vi "RAMM_merFISH_Main.vi"() -> ()   [LabVIEW 2015]
uses:
  CONTROLS/Q_main_element.ctl
  CONTROLS/Q_camera_element.ctl
  CONTROLS/Global parameters.ctl
  CONTROLS/Illumination and filters.ctl
  CONTROLS/Q_DAQ_element.ctl
  CONTROLS/Q_ASI_stage_element.ctl
  CONTROLS/Q_MCL_piezo_element.ctl
  CONTROLS/Q_PUMP_element.ctl
  CONTROLS/Q_VALVE_element.ctl
  <vilib>/vision/Image Controls.llb/IMAQ Image.ctl
  CONTROLS/Q_FPGA_element.ctl
  CONTROLS/Laser emission status.ctl
  GLOBAL/Global_MAIN.vi
  GLOBAL/Global_ABORT.vi
  GLOBAL/Global_CAMERA.vi
  GLOBAL/Global_MCL_piezo.vi
  <vilib>/regexp/Match Regular Expression.xnode
panel:
  in  "Tab general":T1(tab)
  in  "merFISH mode":u16(ring) items=["Embryo", "Single ROI"]
  in  "Close LabView?":bool caption="Close LabView at the end?"
  in  "N movies":i32=1
  in  "Piezo step (um)":dbl=0.05
  in  "Tab small":enum32{"Scanning", "Autofocus", "Fluidics"}(tab)
  in  "Define mosaic":bool
  in  "Save embryo":bool
  in  "Abort scan":bool
  out "Number steps":i32
  out "Scan slider":u8(slide) scale=0.0..100.0
  out "Laser lines manager":i32(listbox)=-1
  in  "Start scan":bool
  in  "step length (nm)":u32=250
  in  "Total  range (nm)":u32=10000
  in  "Illumination source":bool
  in  "Select laser lines":bool
  in  "Discard ROIs":bool
  out "XY positions":cluster{dbl[], dbl[]}[](graph)
  in  "Save X/Y position":bool
  in  "Load X/Y positions":bool
  in  "ROI manager":i32(listbox)
  in  "Brightfield intensity":dbl
  in  "Mosaic size X":i32(ring) items=["1", "3", "5", "7", "9", "11"]
  in  "Mosaic size Y":i32(ring) items=["1", "3", "5", "7", "9", "11"]
  in  "FOV size (um)":dbl=200.0 min=0.0 step=0.1 format="%#.1f"
  in  "Measure QPD":bool
  in  "Init":bool
  in  "PID gains":T2={"proportional gain (Kc)"=10.0, "integral time (Ti, min)"=0.5, "derivative time (Td, min)"=0.0} {"derivative time (Td, min)" format="%.3f"; "integral time (Ti, min)" format="%.3f"; "proportional gain (Kc)" format="%.3f"}
  in  "Autofocus":bool
  in  "Switch":bool
  in  "Autotune?":bool
  in  "Calib autofocus":bool caption="Calibration"
  out "Sensitivity (nm)":dbl
  out "Calibration":cluster{"Y":dbl[], "Y":dbl[]}[](graph)
  in  "Save setpoint":bool
  out "merFISH setpoint":sgl
  in  "Ref channel":u16(ring) items=["X signal", "Y signal"]
  out "Photobleaching manager":i32(listbox)
  in  "Define list":bool
  in  "Two-way valve":bool
  in  "Probe list":i32(listbox)=1
  in  "Pressure (mbar)":dbl min=0.0 max=300.0
  in  "Define injections":bool
  out "Hybridization manager":i32(listbox)
  in  "Buffer list":i32(listbox)=1
  in  "Valve H":u8(knob)=1 min=1 max=22 scale=1.0..22.0
  out "Valve position OUT":u8
  in  "Initialized":bool
  out "Initialization status":T3
  in  "Image contrast":cluster{i32, i32}(slide)={16000, 0} scale=0.0..16000.0
  in  "stop":bool
  out "Error":bool
  in  "Illumination controls":T4 {"641" min=0.0 max=100.0 step=0.1 scale=0.0..100.0; "561" min=0.0 max=100.0 step=0.1 scale=0.0..100.0; "405" min=0.0 max=100.0 step=0.1 scale=0.0..100.0; "488" min=0.0 max=100.0 step=0.1 scale=0.0..100.0; "BF" min=0.0 max=100.0 step=0.1 scale=0.0..100.0}
  in  "Saving path":path=path "E:/DATA"
  in  "Sample name":string="RAMM_Test"
  in  "Save movie":bool
  in  "N frames":i32=100
  out "Slider save movie":u8(slide) scale=0.0..100.0
  out "Frames":i32
  in  "Abort movie":bool
  out "ROI":T5(plugin-control)
  out "Intensity range":cluster{sgl, sgl}(slide) scale=0.0..16000.0
  out "Cooler ON?":bool
  in  "Start acquisition":bool
  out "Sensor Temperature (°C)":sgl
  in  "Exp time (s)":sgl=0.05 format="%#_3g"
  out "Kin time (s)":sgl format="%.3f"
  out "Image":T5(plugin-control)
  in  "Set roi":bool
  in  "Reset roi":bool
  in  "Autofocus automatic correction":bool=TRUE
  out "instruction":string
  out "Autofocus lost":bool
  in  "Alert email adress":string="sergio.espinola@cbs.cnrs.fr " caption="Recipients"
  in  "Display?":bool=TRUE
  in  "DAPI":bool
  in  "Brightfield":bool
  out "merFISH init":T6
  in  "merFISH":bool
  in  "Abort merFISH":bool
  in  "Defaut injection photobleaching":i32[][](array[numeric])=[[10, 500, 350, 0], [0, 1200, 120, 0], [10, 500, 300, 21], [5, 2000, 222, 21], [10, 1200, 300, 22], [5, 800, 350, 1], [0, 150, 100, 1]]
  in  "Q_VALVE":T7={"variant"=variant, "Instruction"=enum."VALVE_initialize"}
  out "MAIN_consumer":errorcluster
  out "ASI":errorcluster
  in  "Q_ASI_stage":T8={"variant"=variant, "Instruction"=enum."ASI_initialize"}
  in  "VISA stage port :":refnum<visa-resource-name>="COM4"
  out "Global parameters":T9 {"# repetitions" min=0; "Dt (s)" min=0 step=1; "Filter list" items=["ET665lp", "zet405/488/561/640m", "None", "None", "None", "None"]}
  out "MAIN_producer":errorcluster
  in  "Q_CAMERA":T10={"variant"=variant, "Instruction"=enum."CAMERA_initialize"}
  in  "Q_main_element":T11={"variant"=variant, "Instruction"=enum."Main_CAMERA_initialization_results"}
  in  "Q_DAQ":T12
  in  "Q_MCL_Piezo":T13
  out "Piezo":errorcluster
  out "DAQ":errorcluster
  out "sCMOS":errorcluster
  in  "Q_PUMP":T14={"variant"=variant, "Instruction"=enum."PUMP_initialize"}
  in  "VISA valve port :":refnum<visa-resource-name>="COM1"
  out "Valve":errorcluster
  out "Pump":errorcluster
  in  "Defaut injection":i32[][](array[numeric])=[[10, 500, 350, 0], [0, 1200, 120, 0], [10, 500, 300, 21], [5, 2000, 222, 21], [10, 1200, 300, 22], [5, 800, 350, 1], [0, 150, 100, 1]]
  out "FPGA":errorcluster
  # "Hamilton valve"
  # "Two-way valve"
  # "Fluigent pump"
  # "First col = Pressure (mbar)\nSecond col = injected volume (ml)\nThird col = Flow rate (µl/min)\nFourth col = valve (#0 is RT)"
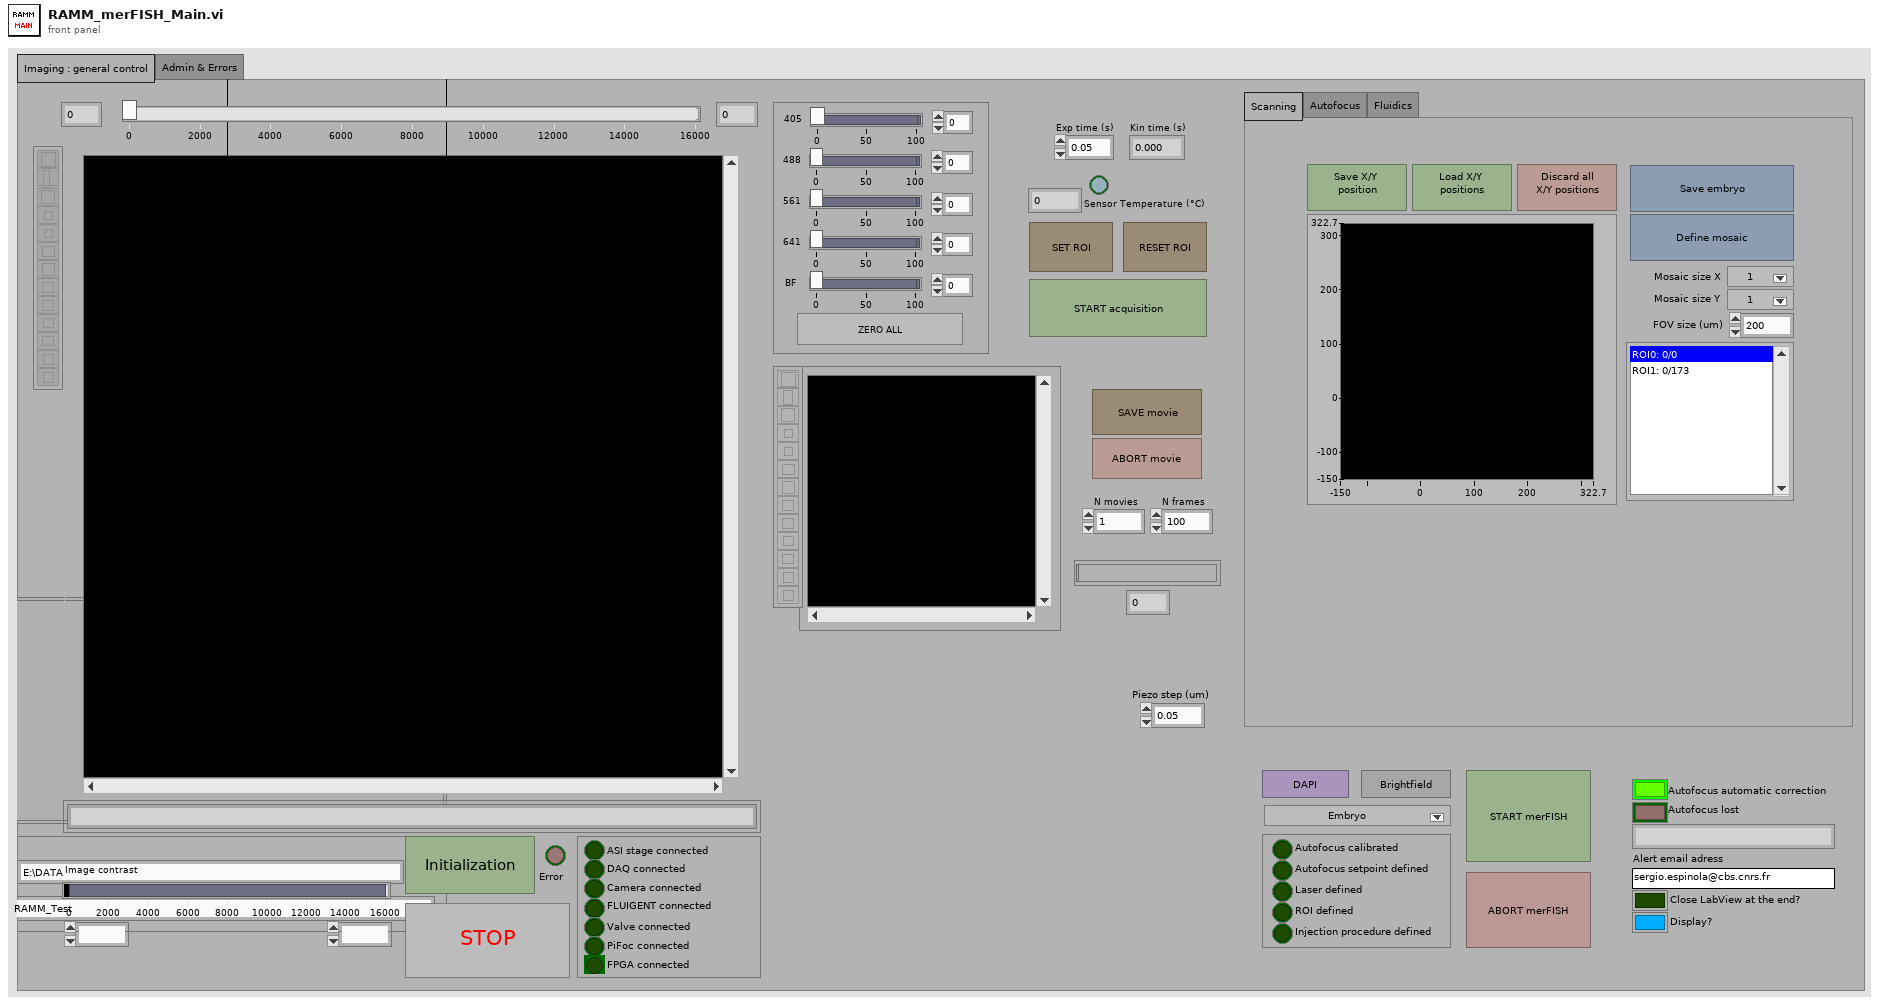
[diagram p1: front panel]
types:
  T1 = enum32{"Imaging : general control", "Admin & Errors"}
  T2 = cluster{"proportional gain (Kc)":dbl, "integral time (Ti, min)":dbl, "derivative time (Td, min)":dbl}
  T3 = cluster{"ASI":bool, "DAQ":bool, "Camera":bool, "Pump":bool, "Valve":bool, "PiFoc":bool, "FPGA":bool}
  T4 = typedef "Illumination and filters.ctl" = cluster{"BF ":dbl, "641":dbl, "561":dbl, "488":dbl, "405":dbl, "ZERO ALL":bool}
  T5 = typedef "IMAQ Image.ctl" = refnum<image>
  T6 = cluster{"Autofocus calibrated":bool, "Autofocus setpoint defined":bool, "Laser defined":bool, "ROI defined":bool, "Injection procedure defined":bool}
  T7 = typedef "Q_VALVE_element.ctl" = cluster{"variant":variant, "Instruction":enum16{"VALVE_idle", "VALVE_initialize", "VALVE_error", "VALVE_security_stop", "VALVE_change_position", "VALVE_two_way_valves", "VALVE_init_merFISH", "VALVE_stop"}}
  T8 = typedef "Q_ASI_stage_element.ctl" = cluster{"variant":variant, "Instruction":enum16{"ASI_idle", "ASI_initialize", "ASI_error", "ASI_security_stop", "ASI_read_XYZ", "ASI_up", "ASI_down", "ASI_left", "ASI_right", "ASI_save_XY", "ASI_move_to_XY", "ASI_brightfield", "ASI_init_scan", "ASI_init_merFISH", "ASI_move_to_XY_merFISH", "ASI_move_to_Z_merFISH", "ASI_init_autofocus_search_merFISH", "ASI_close_autofocus_search_merFISH", "ASI_adjust_piezo_autofocus_merFISH", "ASI_set_piezo_autofocus_to_reference_position_merFISH_TL", "ASI_close_merFISH", "ASI_stop"}}
  T9 = typedef "Global parameters.ctl" = cluster{"405":dbl, "488":dbl, "561":dbl, "641":dbl, "BF":dbl, "X":dbl, "Y":dbl, "Filter list":u16, "Exp time":sgl, "Kinetic time":sgl, "Gain":i32, "Step length (nm)":u32, "Total range (nm)":u32, "Scan illumination\n mode":bool, "Dt (s)":i32, "# repetitions":i32}
  T10 = typedef "Q_camera_element.ctl" = cluster{"variant":variant, "Instruction":enum16{"CAMERA_idle", "CAMERA_initialize", "CAMERA_error", "CAMERA_security_stop", "CAMERA_not_acquiring", "CAMERA_acquiring", "CAMERA_start_acquiring", "CAMERA_stop_acquiring", "CAMERA_change_exposure", "CAMERA_define_ROI", "CAMERA_cooler", "CAMERA_acquire_movie", "CAMERA_init_scan", "CAMERA_check_image_scan", "CAMERA_close_scan", "CAMERA_init_merFISH", "CAMERA_start_acquiring_merFISH", "CAMERA_close_scan_merFISH", "CAMERA_close_merFISH", "CAMERA_STOP"}}
  T11 = typedef "Q_main_element.ctl" = cluster{"variant":variant, "Instruction":enum16{"Main_idle", "Main_initialize", "Main_initialize_TDMS", "Main_initialize_Queue", "Main_error", "Main_DAQ_initialization_results", "Main_ASI_initialization_results", "Main_Piezo_initialization_results", "Main_Valve_initialization_results", "Main_Pump_initialization_results", "Main_CAMERA_initialization_results", "Main_FPGA_initialization_results", "Main_DAQ_error", "Main_ASI_error", "Main_Piezo_error", "Main_CAMERA_error", "Main_Valve_error", "Main_Pump_error", "Main_FPGA_error", "Main_start_acquiring", "Main_not_acquiring", "Main_acquiring", "Main_stop_acquiring", "Main_change_exposure", "Main_change_z_scan_parameters", "Main_define_ROI", "Main_define_mosaic", "Main_read_kinetic_time", "Main_cooler", "Main_read_temperature", "Main_save_XY", "Main_load_XY", "Main_discard_XY", "Main_move_to_XY", "Main_measure_QPD", "Main_autofocus_calibration", "Main_autofocus_initialization", "Main_autofocus_stop", "Main_save_PID", "Main_change_H_valve_position", "Main_two_way_valve", "Main_save_movie", "Main_init_single_scan", "Main_single_scan", "Main_stop_single_scan", "Main_merFISH_illumination_parameters", "Main_merFISH_buffer_probe_list", "Main_merFISH_injections_procedure", "Main_merFISH_save_setpoint", "Main_merFISH_DAPI_parameters", "Main_merFISH_Brightfield_parameters", "Main_merFISH_save_embryo_ROI", "Main_merFISH_init", "Main_merFISH_resume", "Main_merFISH_start_autofocus", "Main_merFISH_open_close_valve_merFISH", "Main_merFISH_open_close_valve_photobleaching", "Main_merFISH_hybridization", "Main_merFISH_move_to_ROI", "Main_merFISH_wait_stabilization", "Main_merFISH_move_to_REF", "Main_merFISH_scan", "Main_merFISH_photobleaching_injection", "Main_merFISH_photobleaching", "Main_merFISH_send_email", "Main_merFISH_close", "Main_STOP"}}
  T12 = typedef "Q_DAQ_element.ctl" = cluster{"variant":variant, "Instruction":enum16{"DAQ_idle", "DAQ_initialize", "DAQ_error", "DAQ_security_stop", "DAQ_init_single_scan", "DAQ_single_scan", "DAQ_init_merFISH", "DAQ_scan_merFISH", "DAQ_photobleaching_merFISH", "DAQ_close_merFISH", "DAQ_stop"}}
  T13 = typedef "Q_MCL_piezo_element.ctl" = cluster{"variant":variant, "Instruction":enum16{"Piezo_idle", "Piezo_initialize", "Piezo_error", "Piezo_security_stop", "Piezo_read_z", "Piezo_move_z", "Piezo_keyboard_move", "Piezo_close_autofocus_calibration_ramp", "Piezo_change_init_state", "Piezo_init_autofocus", "Piezo_init_autofocus_merFISH_TL", "Piezo_autofocus", "Piezo_autofocus_merFISH_TL", "Piezo_stop_autofocus", "Piezo_stop_autofocus_merFISH_TL", "Piezo_autofocus_lost", "Piezo_resume_autofocus_merFISH_TL", "Piezo_check_z_position_merFISH_TL", "Piezo_init_ramp", "Piezo_move_z_ramp", "Piezo_close_ramp", "Piezo_close_merFISH", "Piezo_stop"}}
  T14 = typedef "Q_PUMP_element.ctl" = cluster{"variant":variant, "Instruction":enum16{"PUMP_idle", "PUMP_initialize", "PUMP_error", "PUMP_security_stop", "PUMP_read_pressure", "PUMP_change_pressure", "PUMP_init_merFISH", "PUMP_change_presure_merFISH", "PUMP_zero_pressure_merFISH", "PUMP_close_merFISH", "PUMP_stop"}}
  T15 = typedef "Image Type" = u32
  T16 = cluster{"XY positions":dbl[][], "Laser lines array":dbl[][], "Ramp":dbl[], "Total # z steps":i32, "merFISH path":path, "merFISH init":cluster{"Autofocus calibrated":bool, "Autofocus setpoint defined":bool, "Laser defined":bool, "ROI defined":bool, "Injection procedure defined":bool}, "Hybridization procedure":i32[][], "Total # frames":i32, "Slope":dbl, "Photobleaching procedure":i32[][], "Log file":refnum<file>, "Starting time":dbl, "QPD ref":cluster{"X":sgl, "Y":sgl, "SUM":sgl, "count":u32}, "REF positions":dbl[][]}
  T17 = enum8{"Enabled", "Disabled", "Disabled and Grayed Out"}
  T18 = enum16{"Main_idle", "Main_initialize", "Main_initialize_TDMS", "Main_initialize_Queue", "Main_error", "Main_DAQ_initialization_results", "Main_ASI_initialization_results", "Main_Piezo_initialization_results", "Main_Valve_initialization_results", "Main_Pump_initialization_results", "Main_CAMERA_initialization_results", "Main_FPGA_initialization_results", "Main_DAQ_error", "Main_ASI_error", "Main_Piezo_error", "Main_CAMERA_error", "Main_Valve_error", "Main_Pump_error", "Main_FPGA_error", "Main_start_acquiring", "Main_not_acquiring", "Main_acquiring", "Main_stop_acquiring", "Main_change_exposure", "Main_change_z_scan_parameters", "Main_define_ROI", "Main_define_mosaic", "Main_read_kinetic_time", "Main_cooler", "Main_read_temperature", "Main_save_XY", "Main_load_XY", "Main_discard_XY", "Main_move_to_XY", "Main_measure_QPD", "Main_autofocus_calibration", "Main_autofocus_initialization", "Main_autofocus_stop", "Main_save_PID", "Main_change_H_valve_position", "Main_two_way_valve", "Main_save_movie", "Main_init_single_scan", "Main_single_scan", "Main_stop_single_scan", "Main_merFISH_illumination_parameters", "Main_merFISH_buffer_probe_list", "Main_merFISH_injections_procedure", "Main_merFISH_save_setpoint", "Main_merFISH_DAPI_parameters", "Main_merFISH_Brightfield_parameters", "Main_merFISH_save_embryo_ROI", "Main_merFISH_init", "Main_merFISH_resume", "Main_merFISH_start_autofocus", "Main_merFISH_open_close_valve_merFISH", "Main_merFISH_open_close_valve_photobleaching", "Main_merFISH_hybridization", "Main_merFISH_move_to_ROI", "Main_merFISH_wait_stabilization", "Main_merFISH_move_to_REF", "Main_merFISH_scan", "Main_merFISH_photobleaching_injection", "Main_merFISH_photobleaching", "Main_merFISH_send_email", "Main_merFISH_close", "Main_STOP"}
  T19 = cluster{"Saving path":path, "Sample name":string, "N frames":i32, "N movies":i32, "Start acquisition":bool, "Global parameters":T9}
  T20 = cluster{"XY positions":dbl[][], "REF positions":dbl[][]}
  T21 = cluster{"z step (nm)":u32, "Total range (nm)":u32, "N laser lines merFISH":i32, "Start acquisition":bool, "Brightfield intensity":dbl, "Autofocus":bool, "Probe List Refnum":refnum<vi>, "Injection procedure IN":i32[][], "Valve H":u8, "Measure QPD":bool, "Laser lines array":dbl[][], "Exp time (s)":sgl, "Illumination source":bool, "XY positions":dbl[][], "merFISH mode":u16}
  T22 = cluster{"Start acquisition":bool, "Frame transfer":bool, "Movie path":string}
  T23 = cluster{"Log file":refnum<file>, "Starting time":dbl, "Hybridization procedure":i32[][]}
  T24 = cluster{"XY positions":dbl[][], "Slope":dbl, "Starting time":dbl, "Log file":refnum<file>, "QPD ref":cluster{"X":sgl, "Y":sgl, "SUM":sgl, "count":u32}}
  T25 = cluster{"REF positions":dbl[][], "Slope":dbl, "Starting time":dbl, "Log file":refnum<file>, "XY positions":dbl[][], "QPD ref":cluster{"X":sgl, "Y":sgl, "SUM":sgl, "count":u32}}
  T26 = cluster{"QPD ref":cluster{"X":sgl, "Y":sgl, "SUM":sgl, "count":u32}, "Slope":dbl, "Log file":refnum<file>, "Starting time":dbl}
  T27 = cluster{"Ramp":dbl[], "merFISH path":path, "Total # frames":i32, "Display?":bool, "Probe list":refnum<vi>}
  T28 = cluster{"ROI #":i32, "Probe #":i32, "Folder# ":i32, "Embryo #":i32}
  T29 = cluster{"Photobleaching procedure":i32[][], "Log file":refnum<file>, "Starting time":dbl}
  T30 = cluster{"Hybridization procedure":i32[][], "Photobleaching procedure":i32[][], "Alert email adress":string, "Exp time (s)":sgl, "Total  range (nm)":u32, "step length (nm)":u32, "ROIs":dbl[][], "Laser lines array":dbl[][], "merFISH cluster":cluster{"Autofocus calibrated":bool, "Autofocus setpoint defined":bool, "Laser defined":bool, "ROI defined":bool, "Injection procedure defined":bool}, "Sample name":string, "FOV size":dbl, "Mosaic size":u16[], "PID gains":cluster{"proportional gain (Kc)":dbl, "integral time (Ti, min)":dbl, "derivative time (Td, min)":dbl}, "Illumination source":bool, "Brightfield intensity":dbl, "merFISH path":path, "QPD ref":cluster{"X":sgl, "Y":sgl, "SUM":sgl, "count":u32}, "REFs":dbl[][], "N movies":i32, "N frames":i32}
  T31 = cluster{"Hybridization name":string[], "Photobleaching name":string[], "Laser names":string[], "Buffer list names":string[][], "Probe list names":string[][]}
  T32 = cluster{"X":sgl, "Y":sgl, "SUM":sgl, "count":u32}
  T33 = cluster{"Global Rectangle":i32[], "Contours":cluster{"Contour Type":u32, "ROI Type":u32, "Points":i32[]}[]}
  T34 = cluster{"Maximal Value":sgl, "Minimal Value":sgl}
  T35 = cluster{"queue FPGA":refnum<queue>, "queue pump":refnum<queue>, "queue valve":refnum<queue>, "queue DAQ":refnum<queue>, "queue CAMERA":refnum<queue>, "queue ASI stage":refnum<queue>, "queue piezo":refnum<queue>}
  T36 = cluster{"Z_position_file path":path, "Movie path":path, "Acquisition_parameters path":path}
  T37 = enum16{"open", "open or create", "create or replace", "create", "open (read-only)"}
  T38 = typedef "Q_FPGA_element.ctl" = cluster{"variant":variant, "Instruction":enum16{"FPGA_idle", "FPGA_initialize", "FPGA_error", "FPGA_security_stop", "FPGA_laser", "FPGA_start_stop_measure_QPD", "FPGA_measure_QPD", "FPGA_measure_QPD_noise", "FPGA_stop_measure_QPD", "FPGA_init_autofocus", "FPGA_init_single_scan", "FPGA_stop_single_scan", "FPGA_init_merFISH", "FPGA_measure_QPD_merFISH", "FPGA_init_scan_merFISH", "FPGA_scan_merFISH", "FPGA_close_merFISH", "FPGA_stop"}}
  T39 = typedef "Laser emission status.ctl" = cluster{"405":bool, "488":bool, "561":bool, "641":bool, "BF":bool}
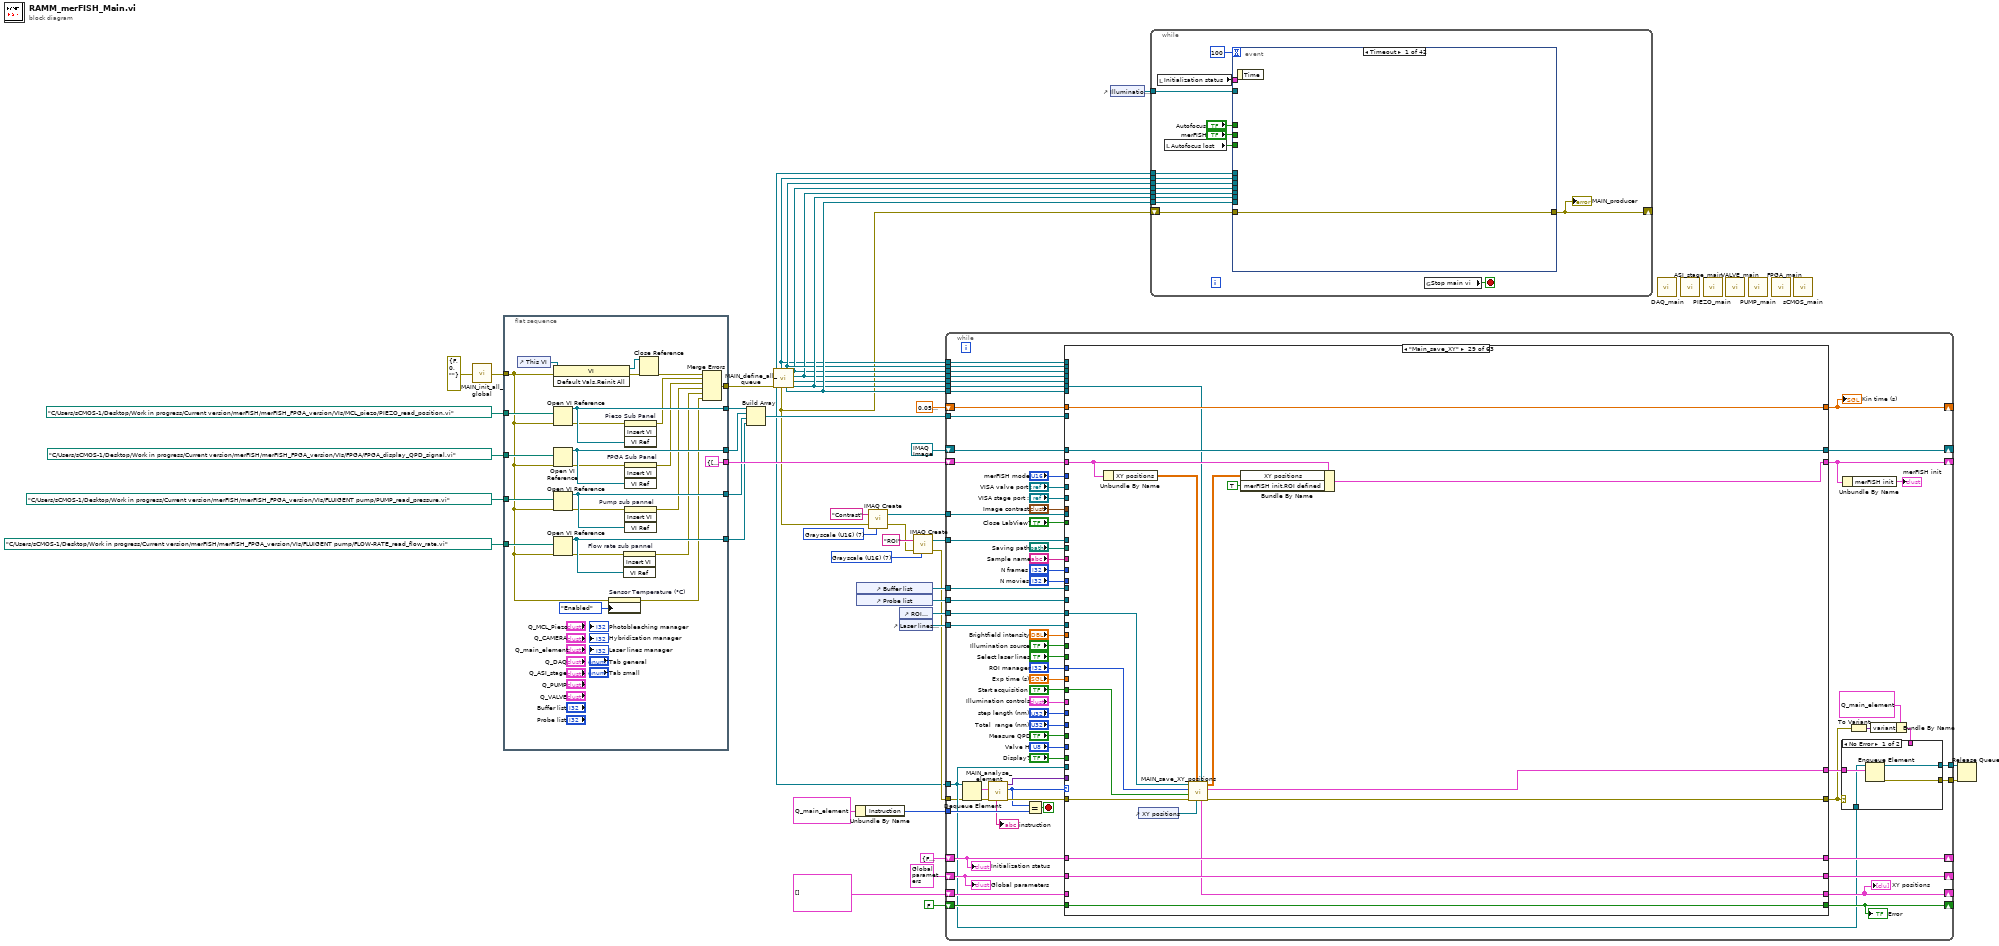
[diagram p0: block diagram]
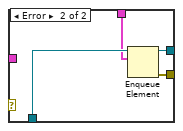
[diagram p2: hidden frame]
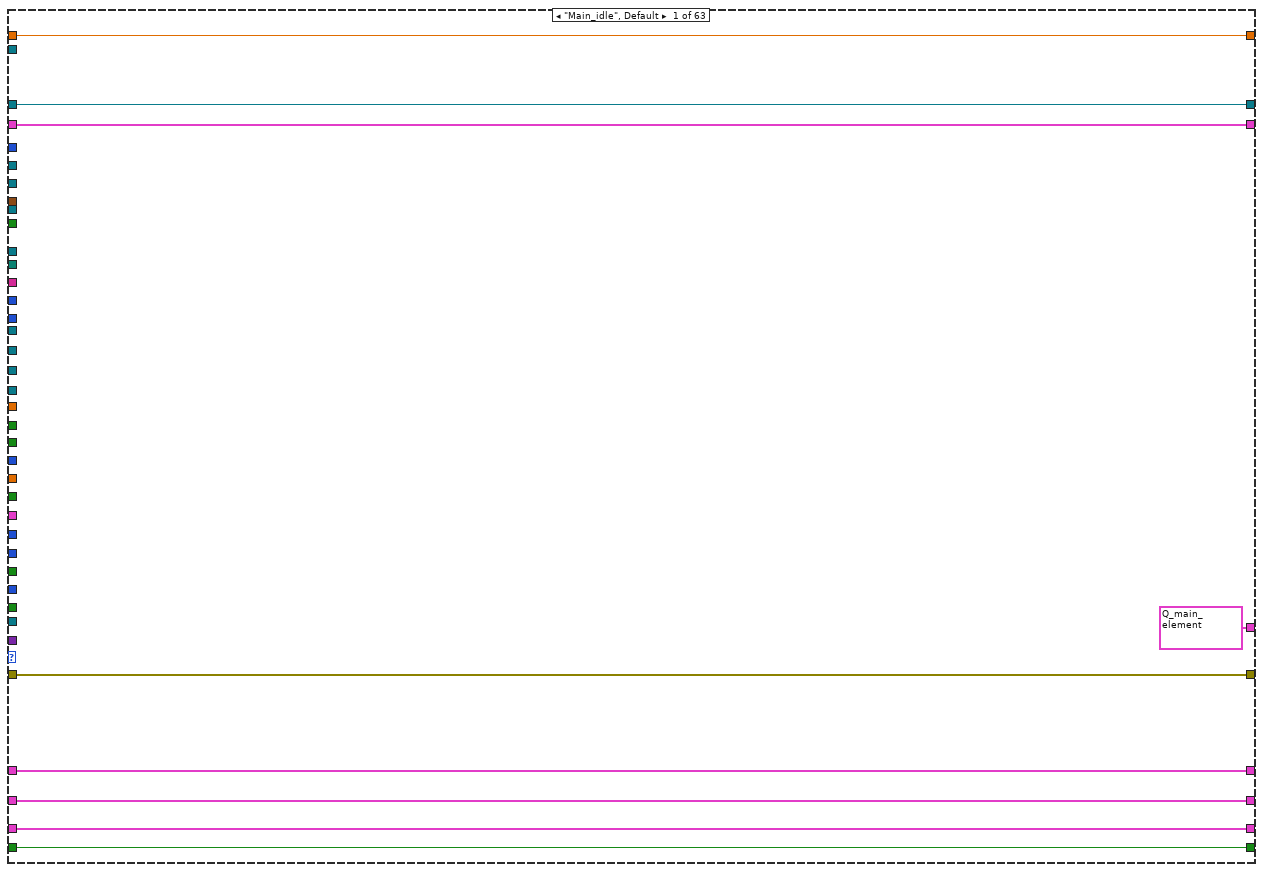
[diagram p3: hidden frame]
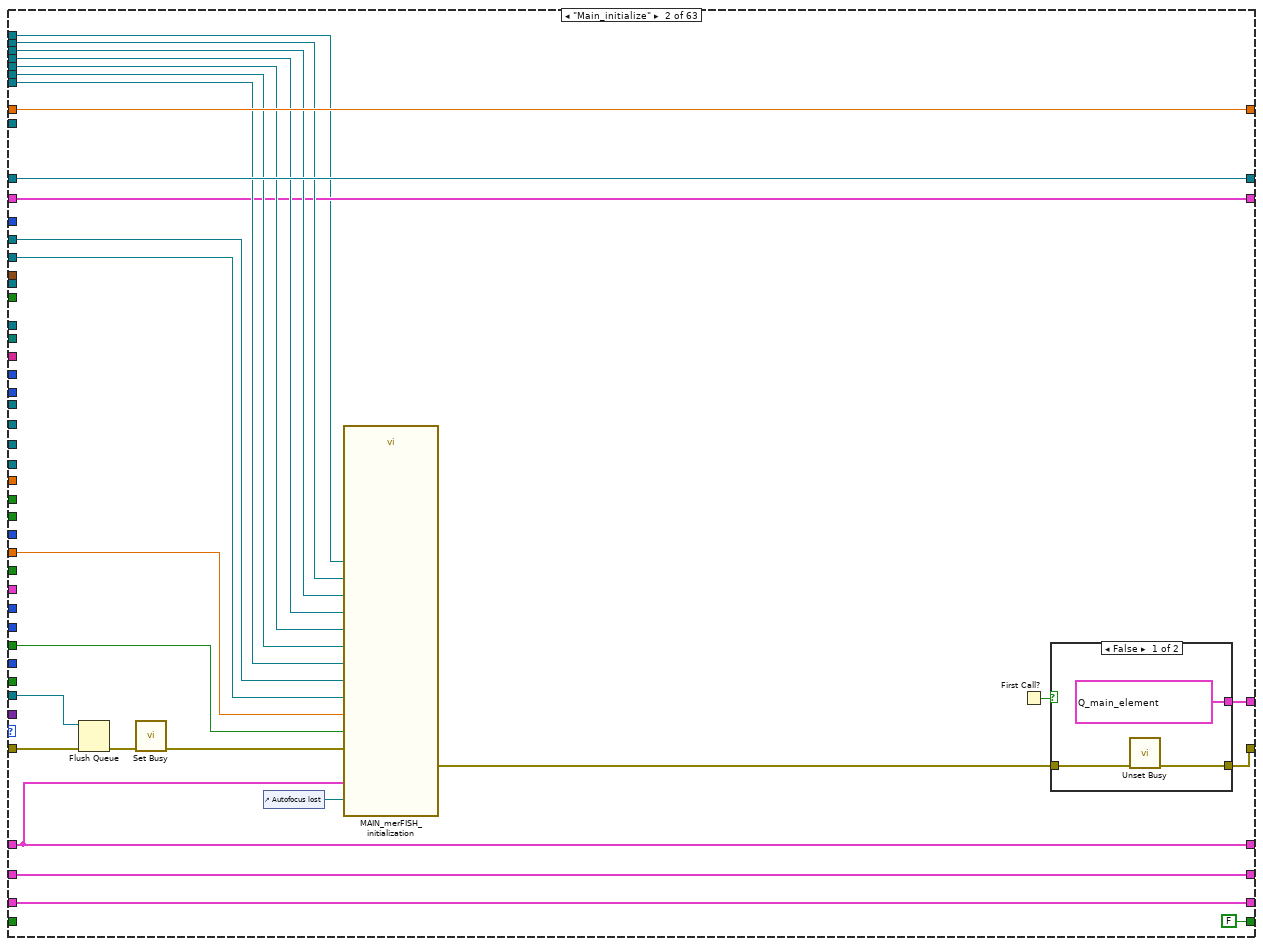
[diagram p4: hidden frame]
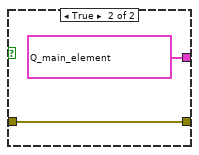
[diagram p5: hidden frame]
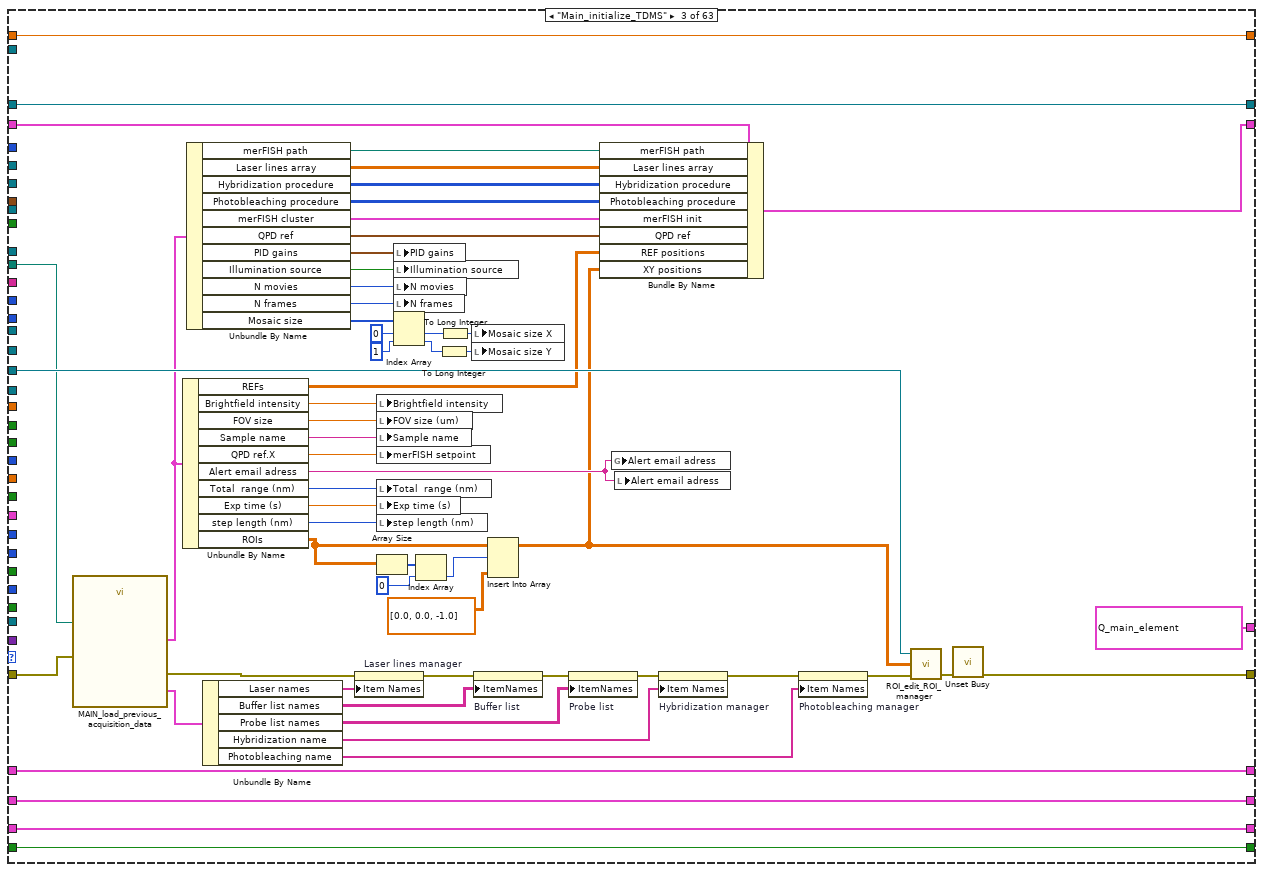
[diagram p6: hidden frame]
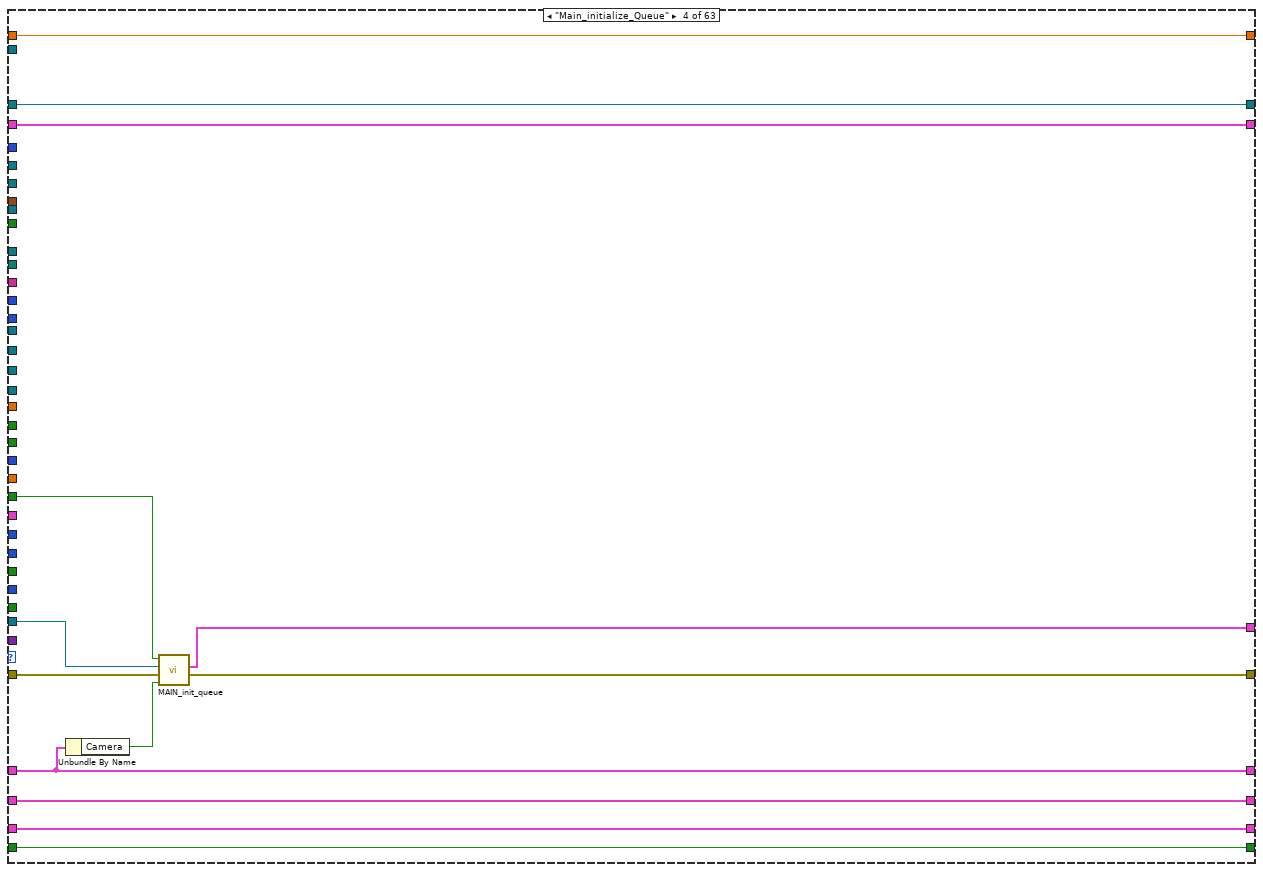
[diagram p7: hidden frame]
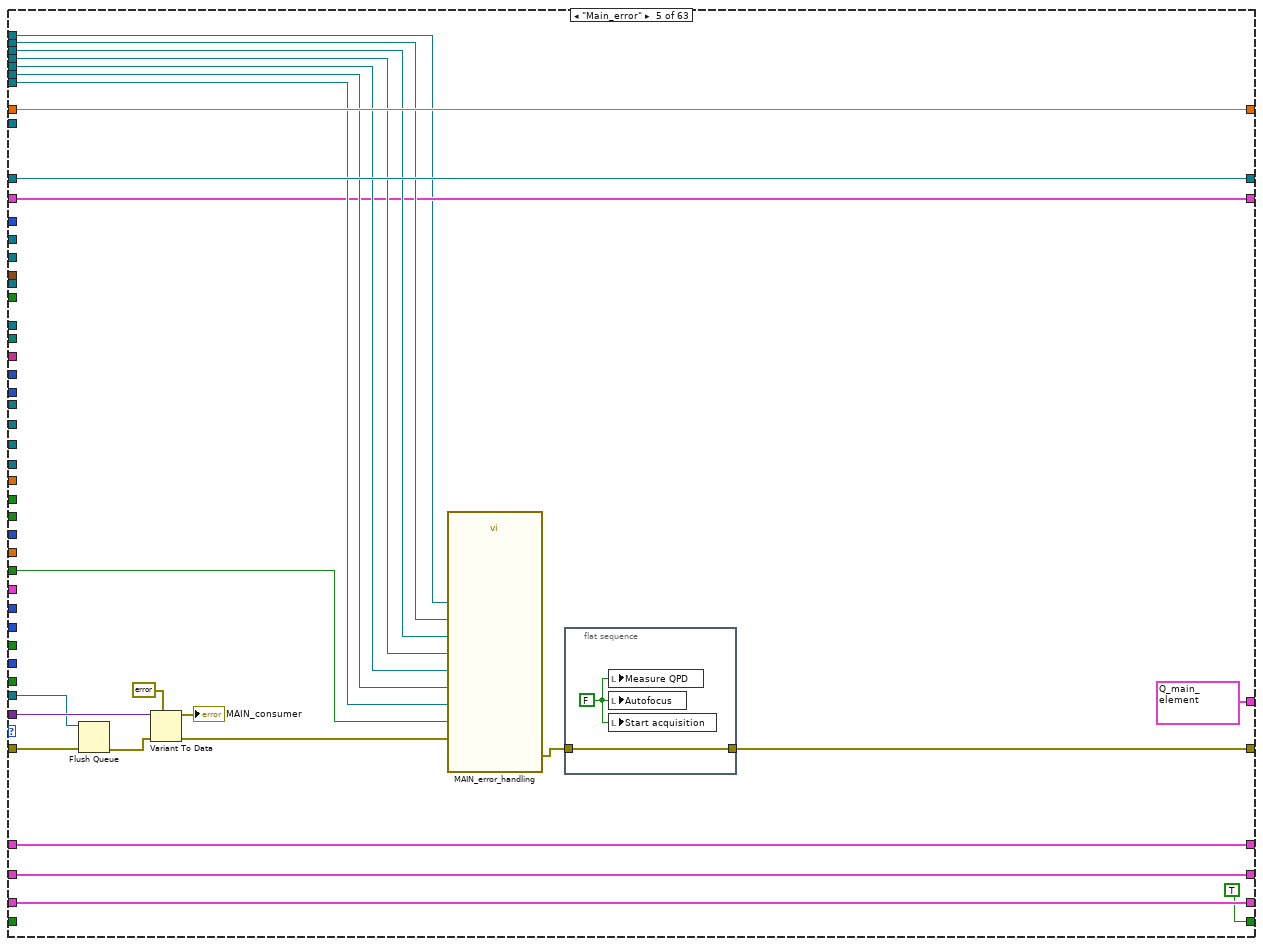
[diagram p8: hidden frame]
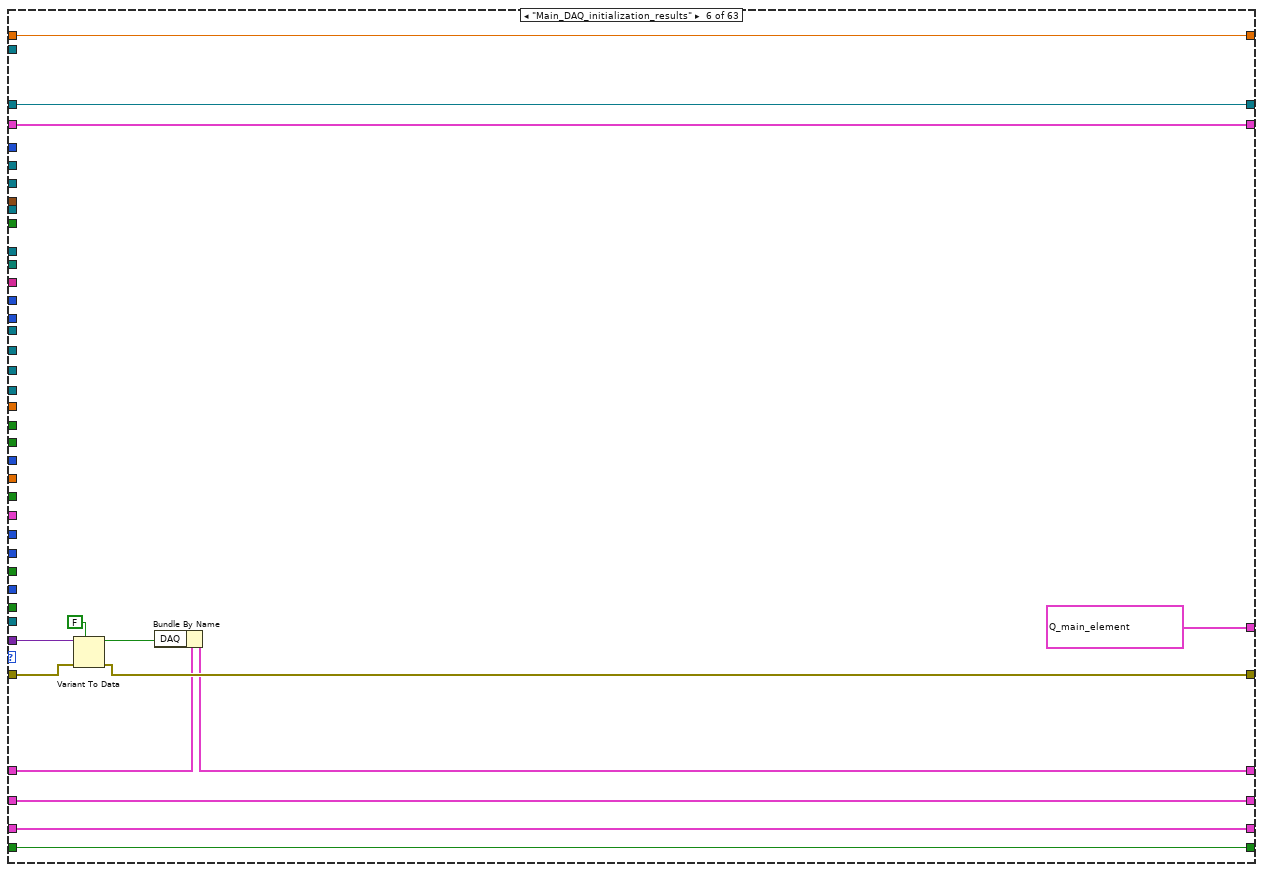
[diagram p9: hidden frame]
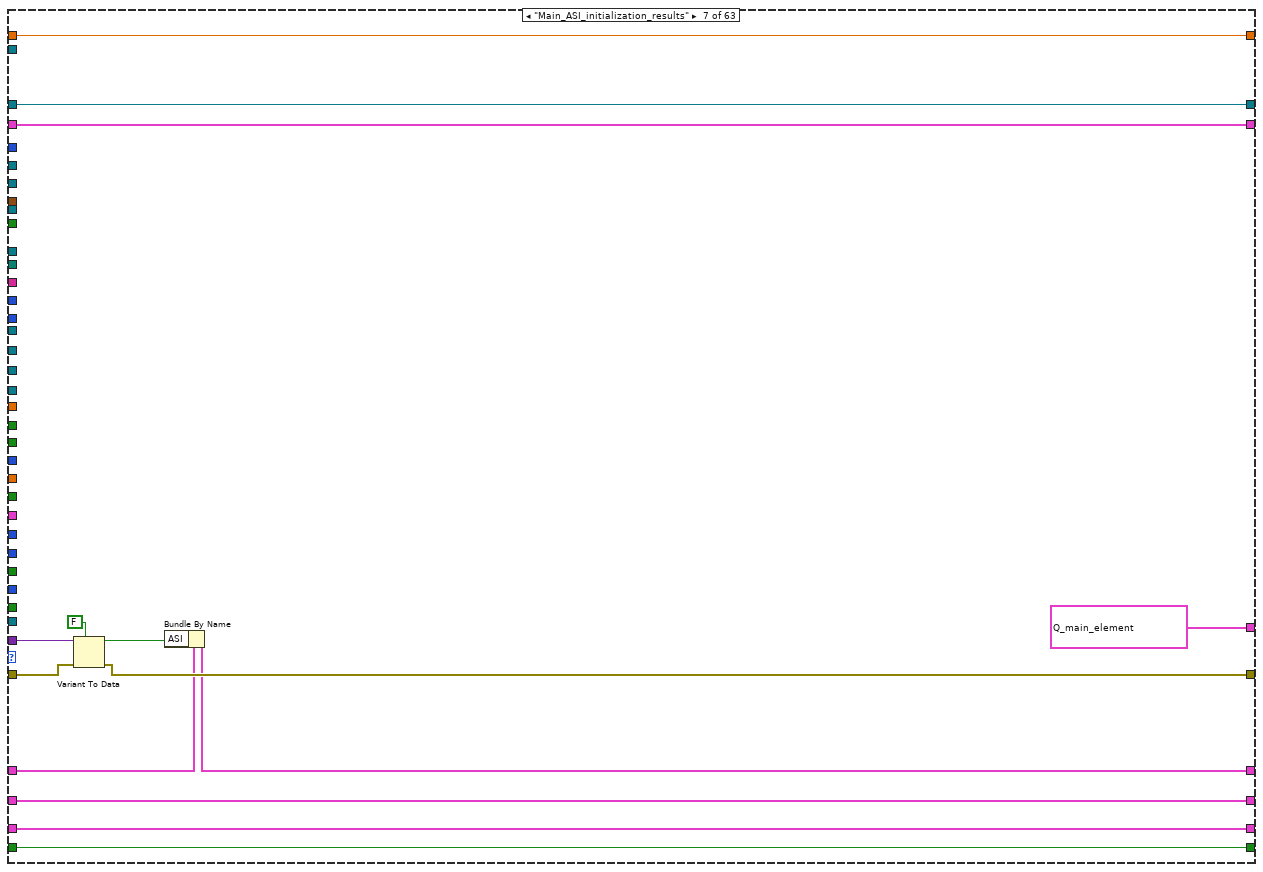
[diagram p10: hidden frame]
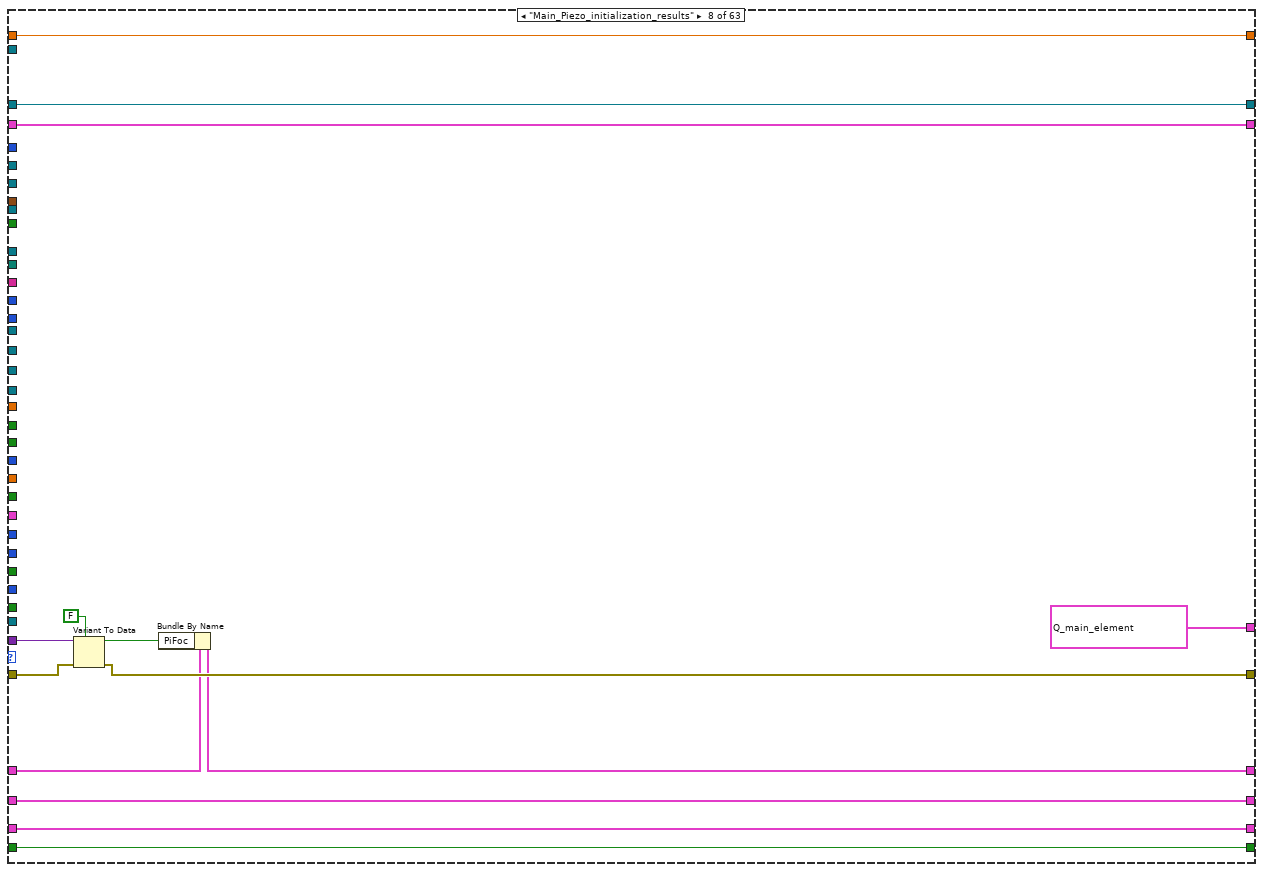
[diagram p11: hidden frame]
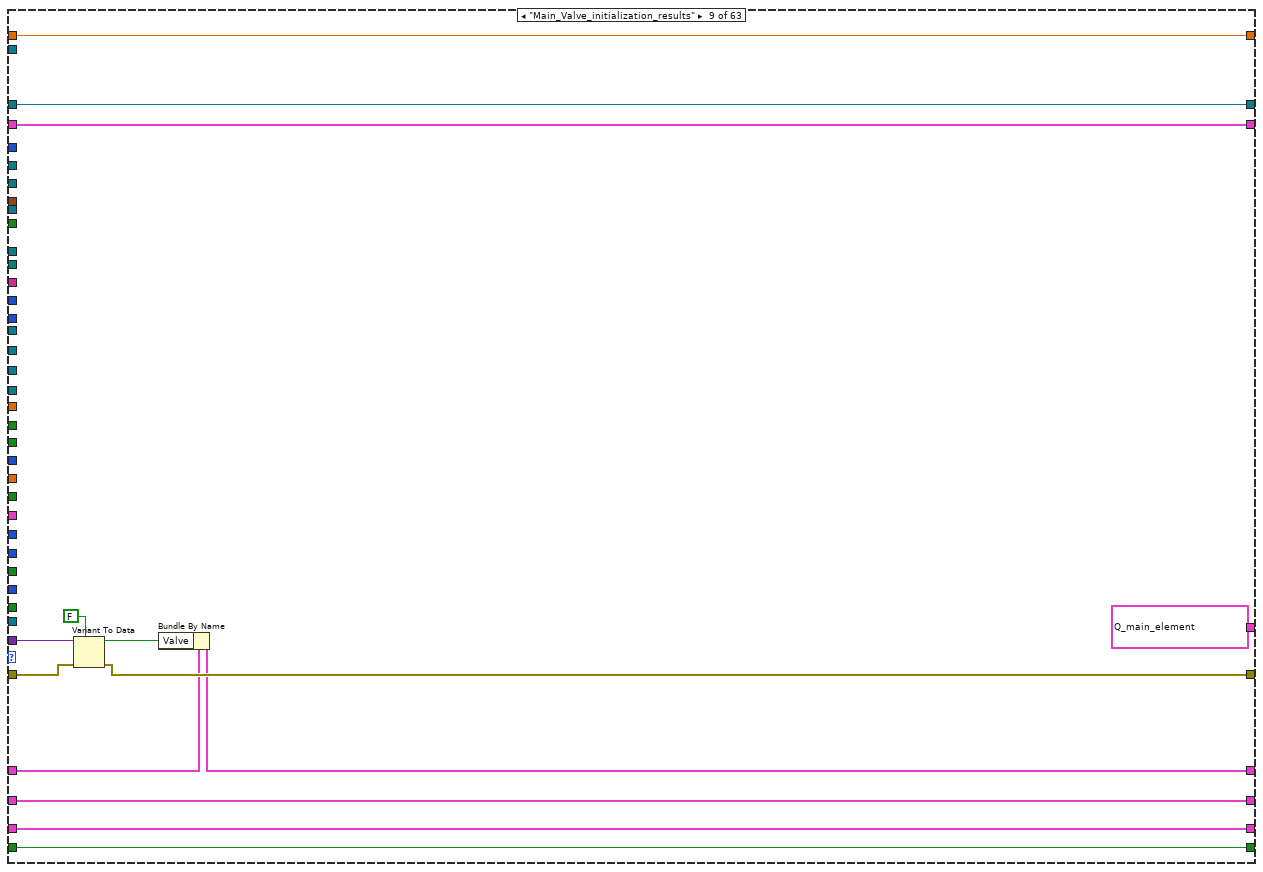
[diagram p12: hidden frame]
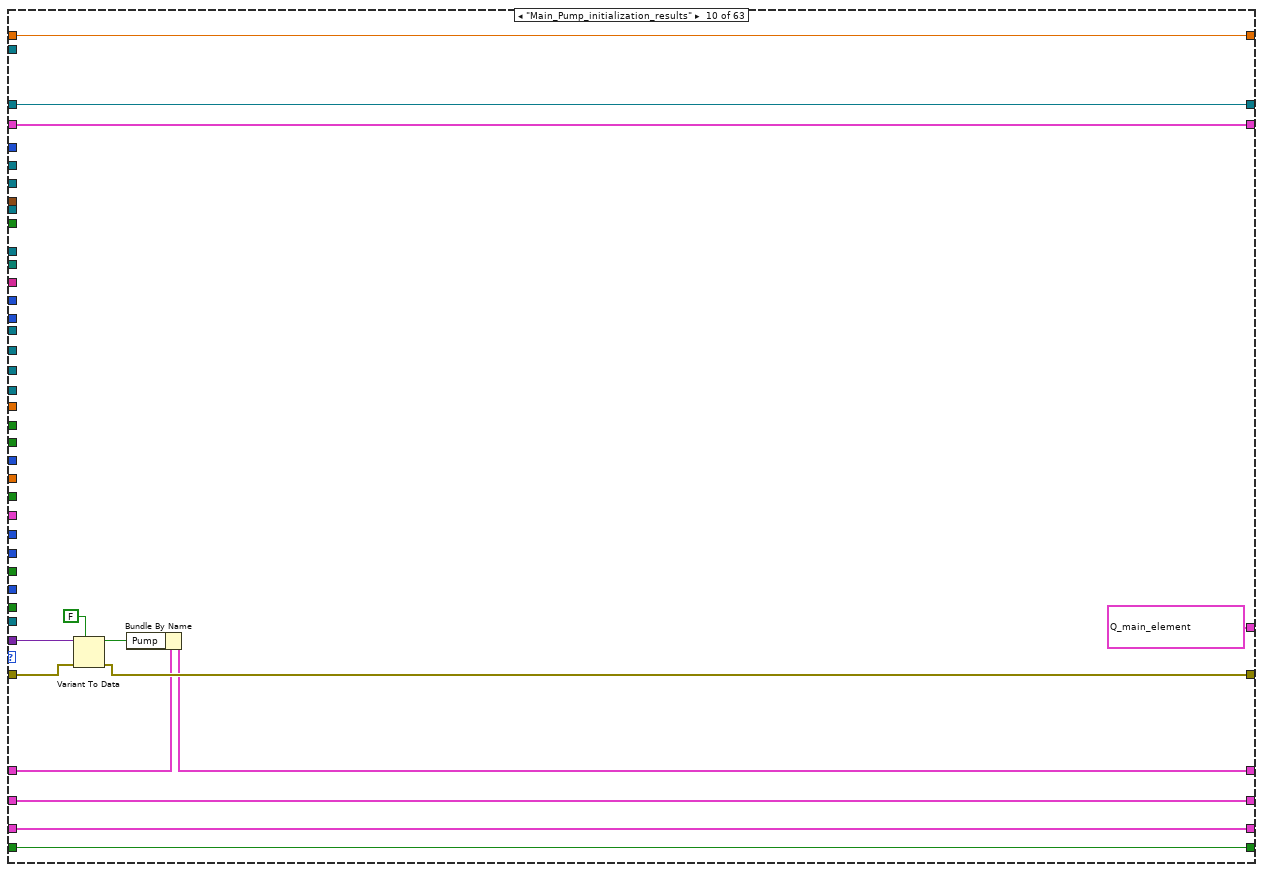
[diagram p13: hidden frame]
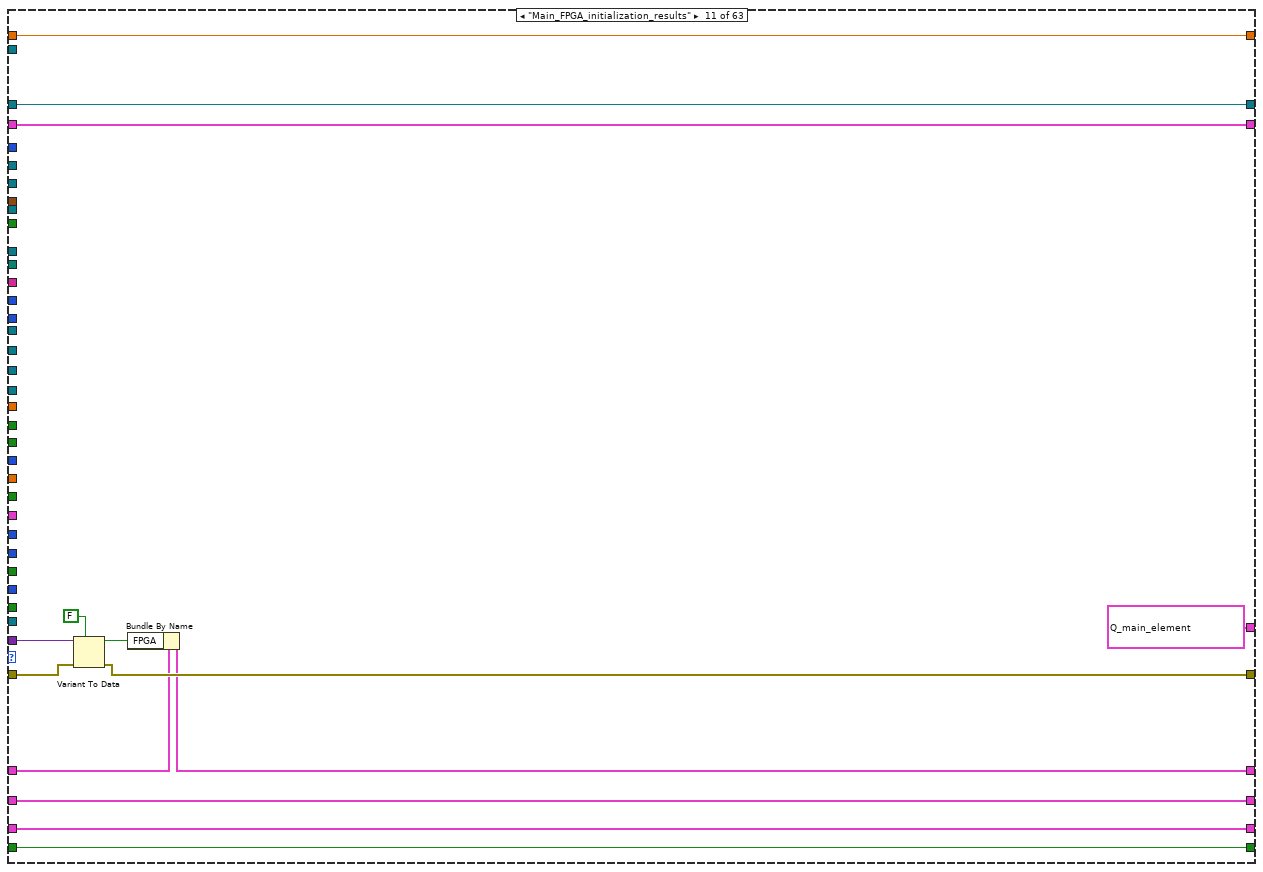
[diagram p14: hidden frame]
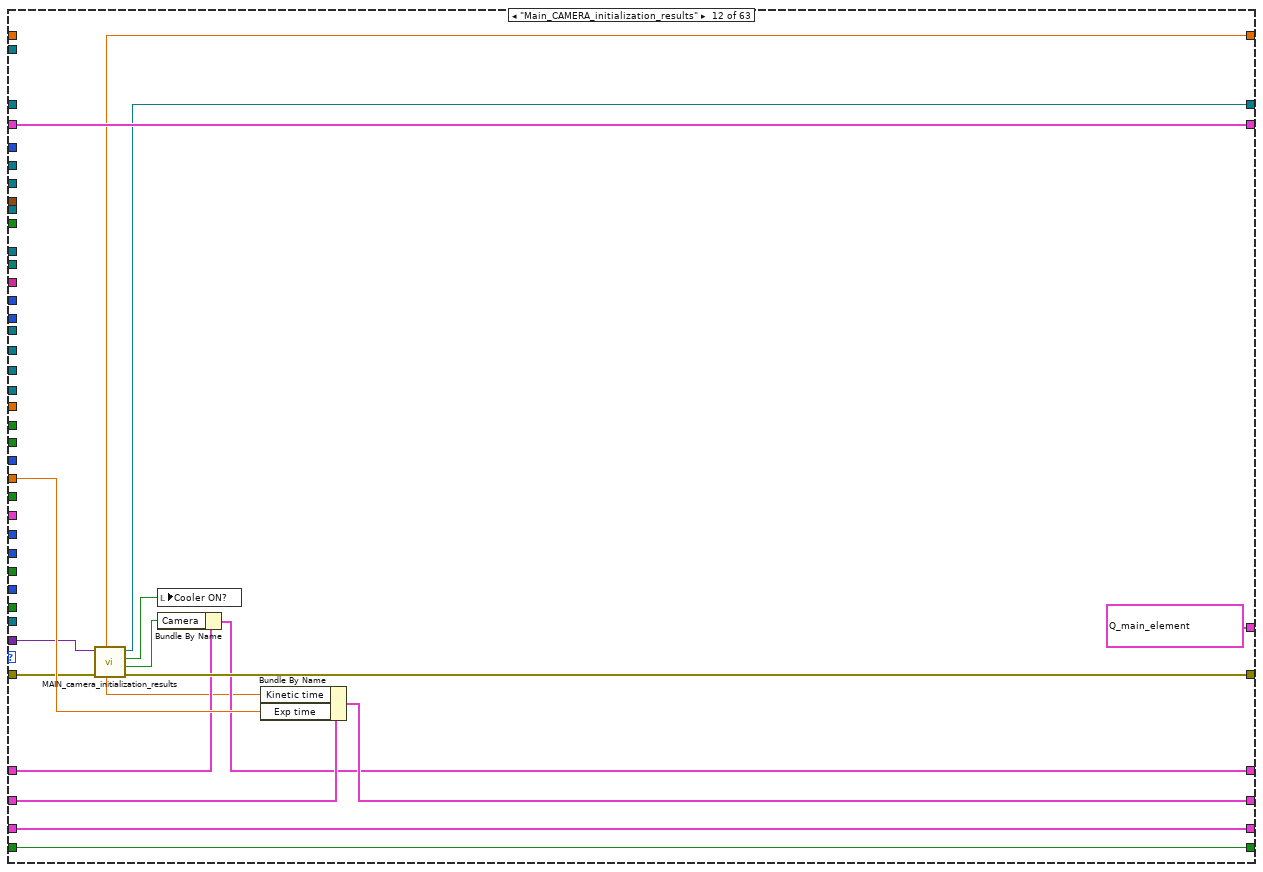
[diagram p15: hidden frame]
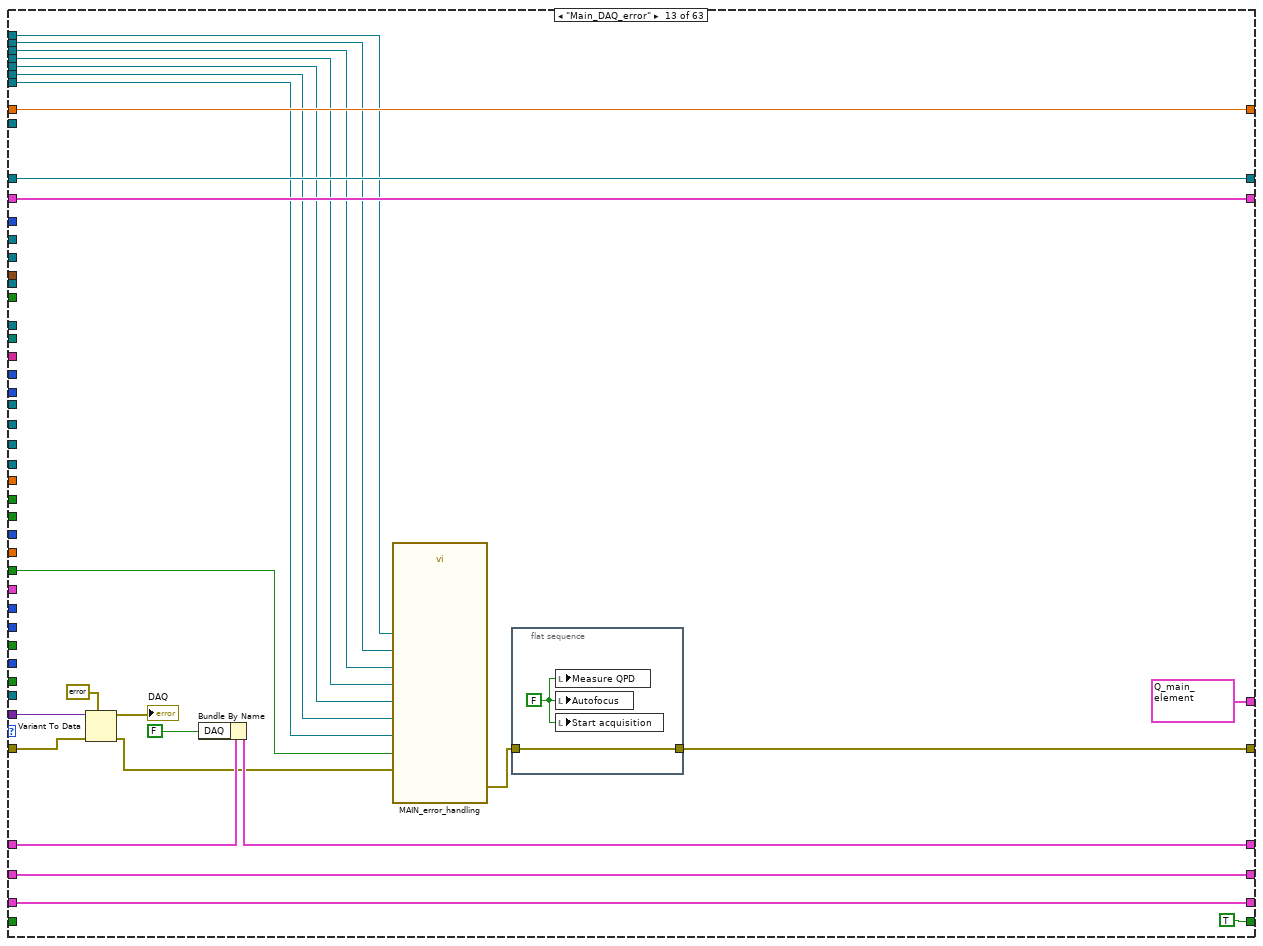
[diagram p16: hidden frame]
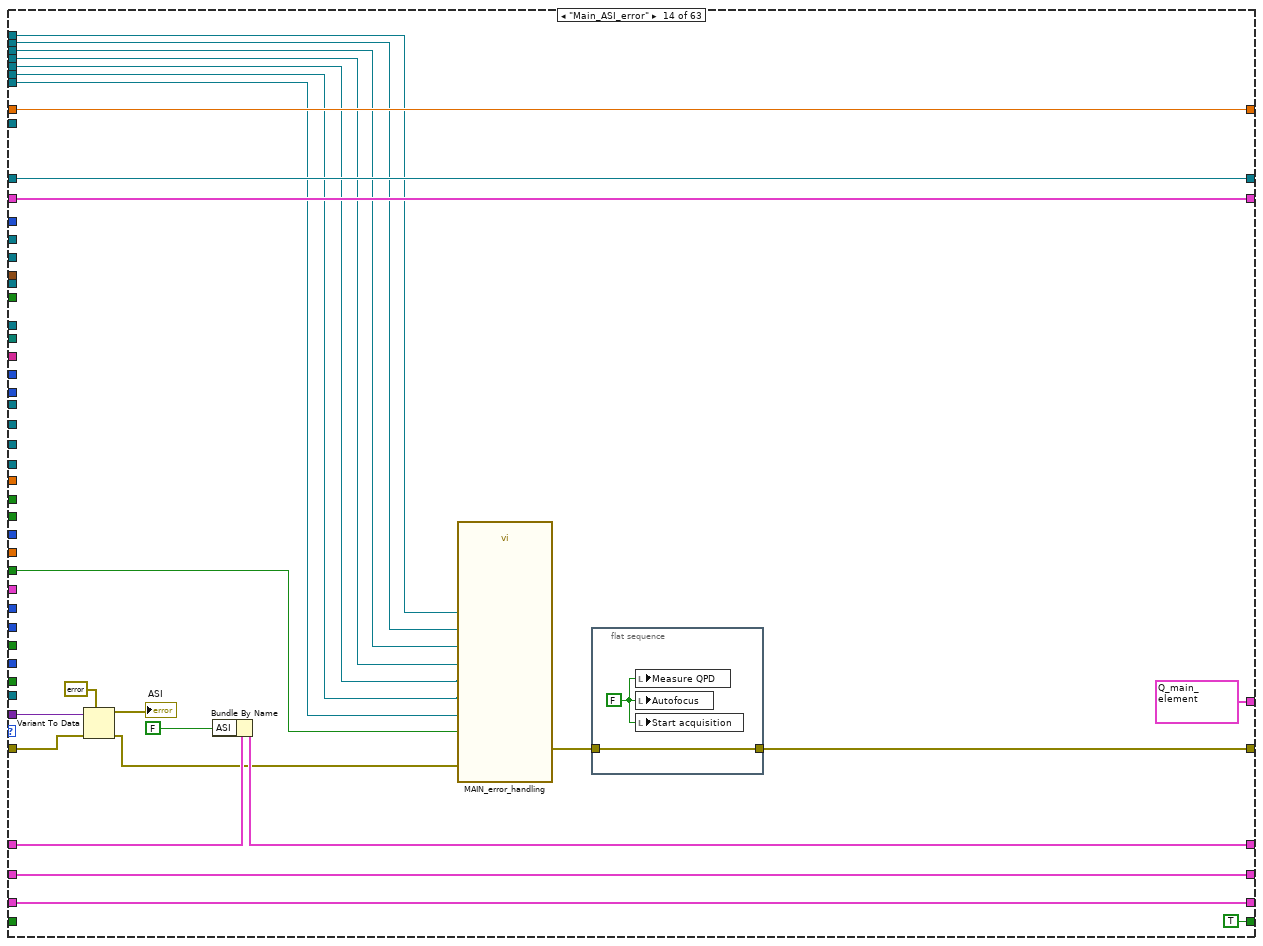
[diagram p17: hidden frame]
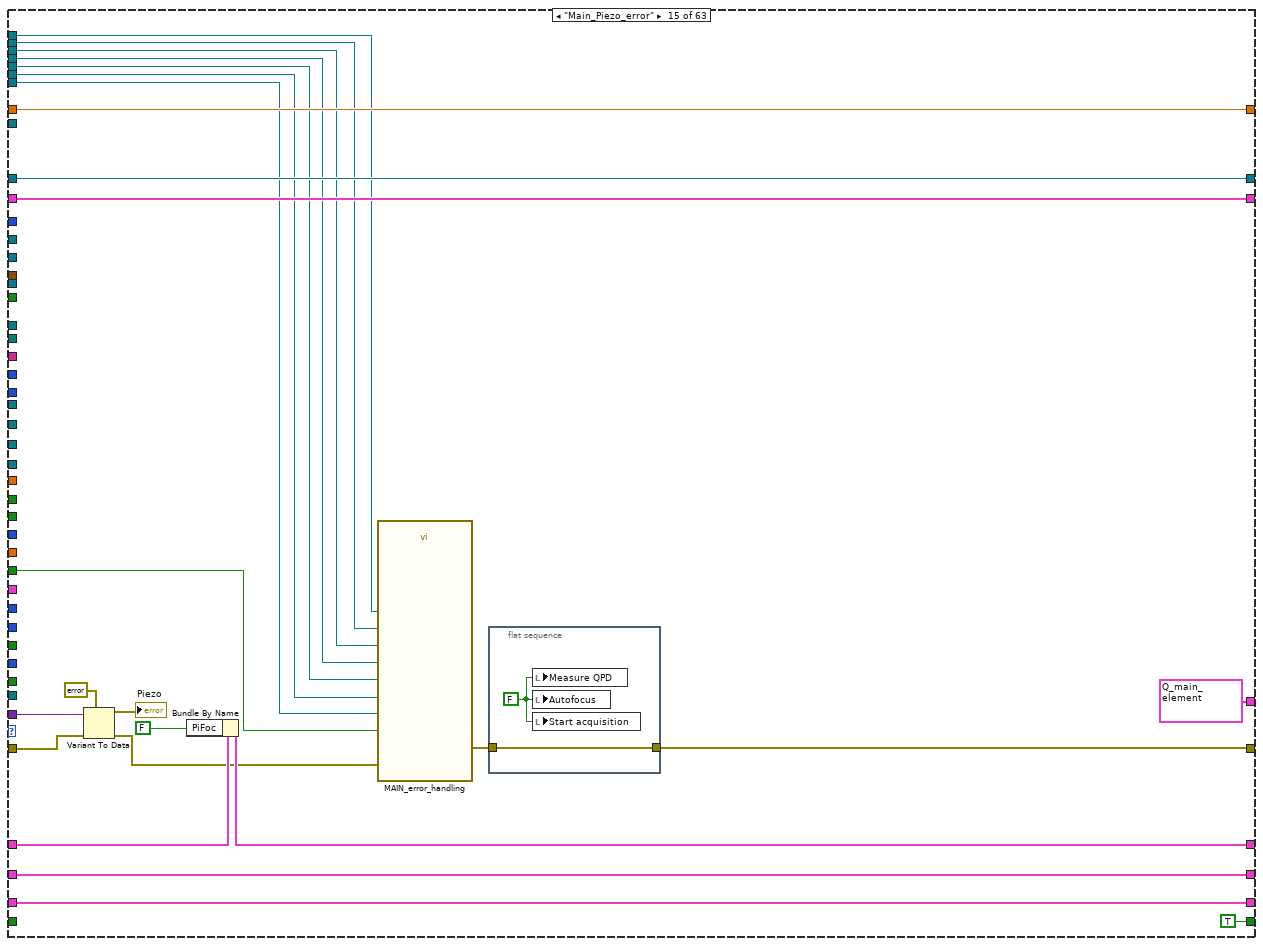
[diagram p18: hidden frame]
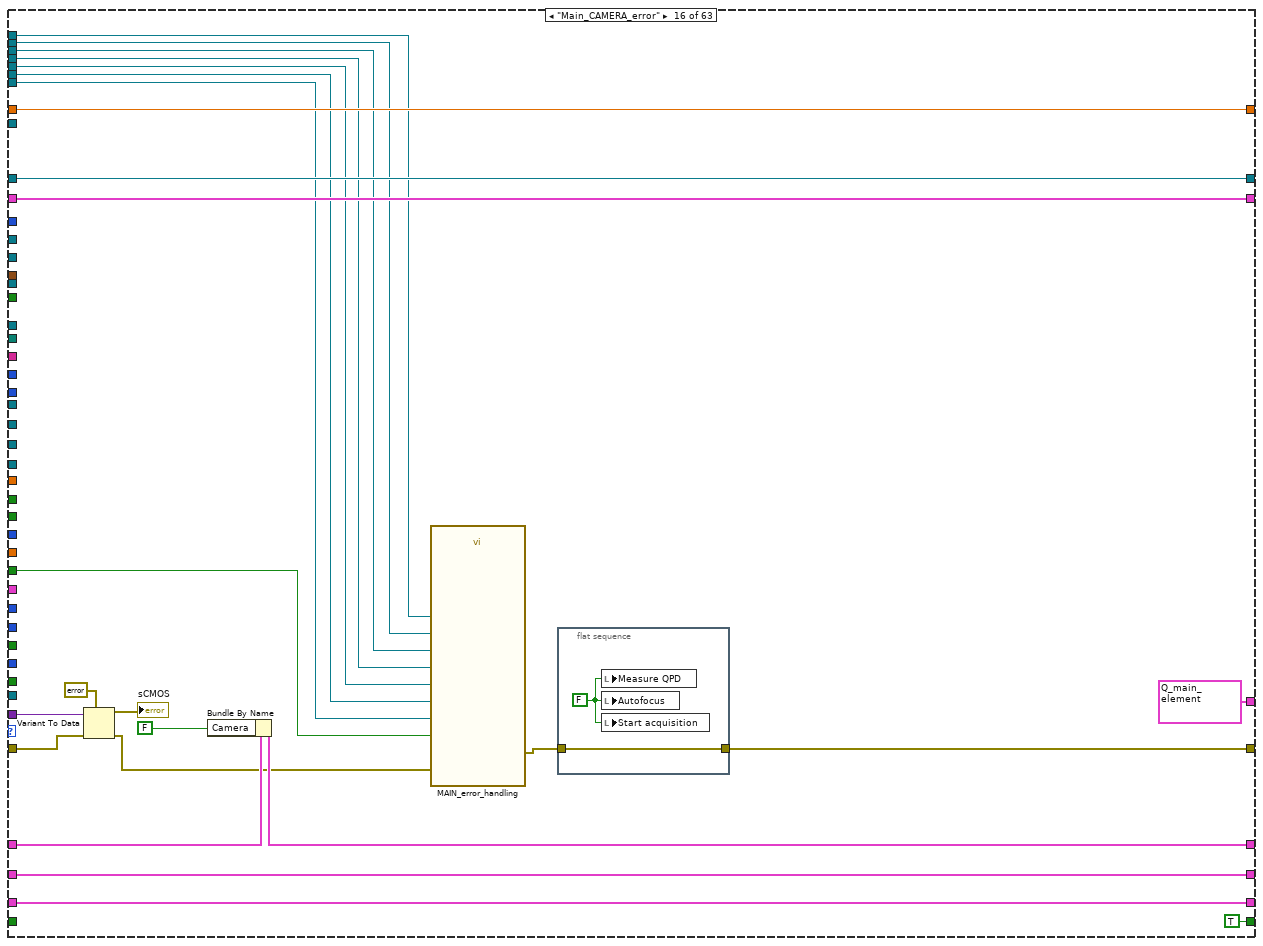
[diagram p19: hidden frame]
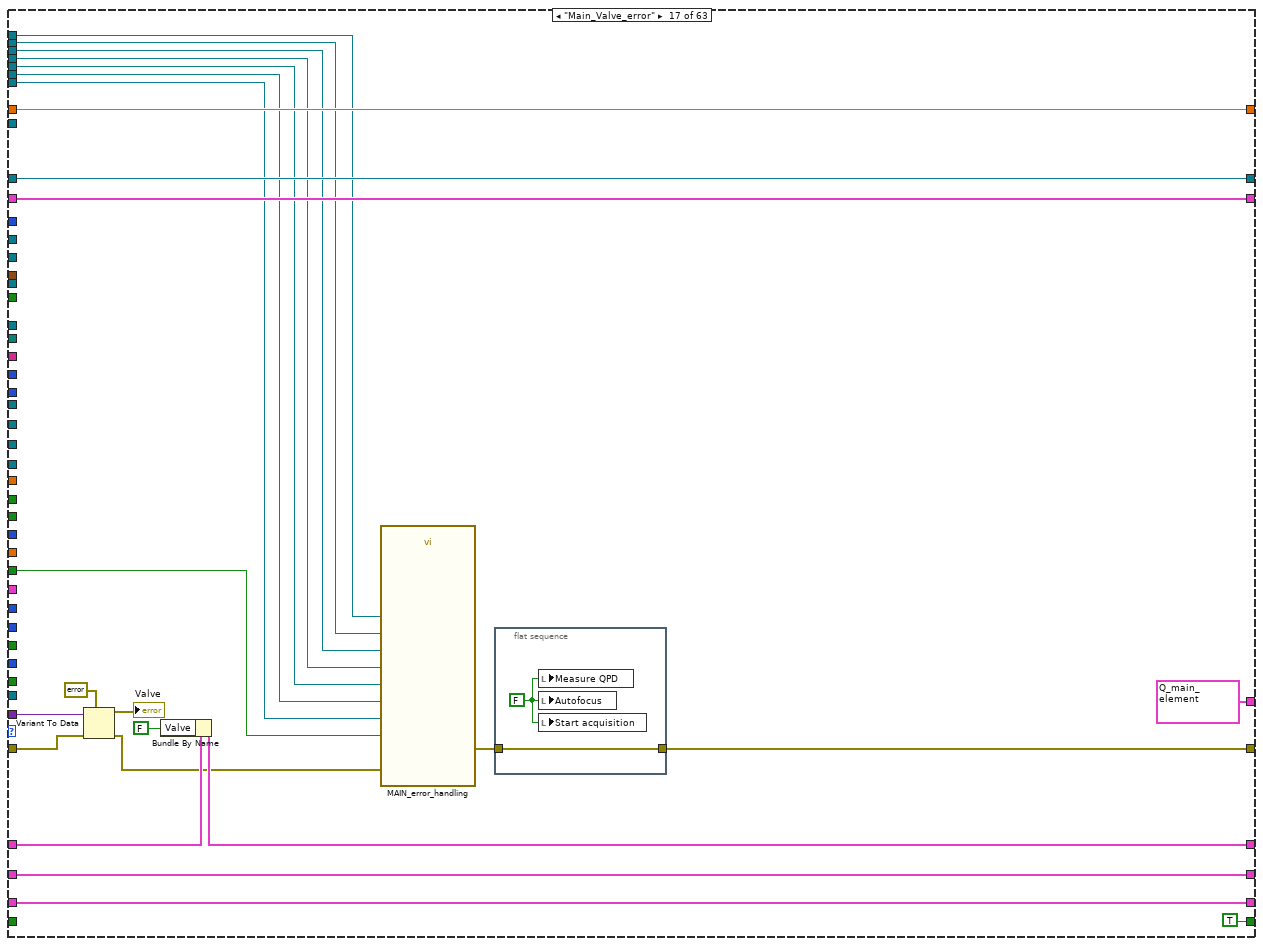
[diagram p20: hidden frame]
diagram:
  w39 = T15 7 items=["Grayscale (U8)", "Grayscale (I16)", "Grayscale (SGL)", "Complex (CSG)", "RGB (U32)", "HSL (U32)", "RGB (U64)", "Grayscale (U16)"] ("Image Type")
  w40 = T15 7 items=["Grayscale (U8)", "Grayscale (I16)", "Grayscale (SGL)", "Complex (CSG)", "RGB (U32)", "HSL (U32)", "RGB (U64)", "Grayscale (U16)"] ("Image Type")
  n1 = call "MAIN_init_all_global.vi"("error in"=errorcluster {"status"=FALSE, "code"=0, "source"=""} ("error in 1 (no error)")) -> ("error out"=w14:errorcluster)
  n2 = flat-sequence {
    tunnel: path "C:/Users/sCMOS-1/Desktop/Work in progress/Current version/merFISH/merFISH_FPGA_version/VIs/MCL_piezo/PIEZO_read_position.vi" ("vi path") -> [w70]
    tunnel: path "C:/Users/sCMOS-1/Desktop/Work in progress/Current version/merFISH/merFISH_FPGA_version/VIs/FPGA/FPGA_display_QPD_signal.vi" ("vi path") -> [w69]
    tunnel: [w68] -> w28
    tunnel: [w67] -> w27
    tunnel: [T16 {"XY positions"=[], "Laser lines array"=[], "Ramp"=[], "Total # z steps"=0, "merFISH path"=path "", "merFISH init"={"Autofocus calibrated"=FALSE, "Autofocus setpoint defined"=FALSE, "Laser defined"=FALSE, "ROI defined"=FALSE, "Injection procedure defined"=FALSE}, "Hybridization procedure"=[], "Total # frames"=0, "Slope"=0.0, "Photobleaching procedure"=[], "Log file"=refnum, "Starting time"=0.0, "QPD ref"={"X"=0.0, "Y"=0.0, "SUM"=0.0, "count"=0}, "REF positions"=[]} ("merFISH parameters")] -> w21
    tunnel: path "C:/Users/sCMOS-1/Desktop/Work in progress/Current version/merFISH/merFISH_FPGA_version/VIs/FLUIGENT pump/PUMP_read_pressure.vi" ("vi path") -> [w66]
    tunnel: [w65] -> w19
    tunnel: [w64] -> w12
    tunnel: path "C:/Users/sCMOS-1/Desktop/Work in progress/Current version/merFISH/merFISH_FPGA_version/VIs/FLUIGENT pump/FLOW-RATE_read_flow_rate.vi" ("vi path") -> [w63]
    tunnel: [w62] -> w15
    tunnel: w14 -> [w61]
    frame #0 {
      n3 = control-ref of="This VI"() -> (w58:refnum<vi>)
      n4 = Open VI Reference(vi path=w70, error in (no error)=w61) -> (vi reference=w68:refnum<vi>, error out=w57:errorcluster)  [unwired: 4 in]
      n5 = Open VI Reference(vi path=w69, error in (no error)=w61) -> (vi reference=w67:refnum<vi>, error out=w54:errorcluster)  [unwired: 4 in]
      n6 = Open VI Reference(vi path=w66, error in (no error)=w61) -> (vi reference=w65:refnum<vi>, error out=w50:errorcluster)  [unwired: 4 in]
      n7 = Open VI Reference(vi path=w63, error in (no error)=w61) -> (vi reference=w62:refnum<vi>, error out=w49:errorcluster)  [unwired: 4 in]
      n8 = invoke class="VI" method="Default Vals.Reinit All"(reference=w58, error in=w61) -> (reference out=w60:refnum<vi>, error out=w59:errorcluster)  [unwired: 1 in, 1 out]
      n9 = property on="Sensor Temperature (°C)" class="DigNum (strict)"(error in=w61, "DisabledEnum"=T17."Enabled" ("Disabled")) -> (error out=w47:errorcluster)  [unwired: 1 in, 1 out]
      n10 = invoke on="Flow rate sub pannel" class="SubPnl" method="Insert VI"(error in=w49, "VI Ref"=w62) -> (error out=w48:errorcluster)  [unwired: 2 in, 3 out]
      n11 = invoke on="Piezo Sub Panel" class="SubPnl" method="Insert VI"(error in=w57, "VI Ref"=w68) -> (error out=w56:errorcluster)  [unwired: 2 in, 3 out]
      n12 = invoke on="FPGA Sub Panel" class="SubPnl" method="Insert VI"(error in=w54, "VI Ref"=w67) -> (error out=w53:errorcluster)  [unwired: 2 in, 3 out]
      n13 = invoke on="Pump sub pannel" class="SubPnl" method="Insert VI"(error in=w50, "VI Ref"=w65) -> (error out=w52:errorcluster)  [unwired: 2 in, 3 out]
      n14 = Close Reference(reference=w60, error in (no error)=w59) -> (error out=w55:errorcluster)
      n15 = Merge Errors(w55, w56, w53, w52, w48, w47) -> (w64:errorcluster)
    }
  }
  n16 = Build Array(w28, w27, w19, w15) -> (w26:refnum<vi>[])
  n17 = call "MAIN_define_all_queue.vi"("error in"=w12) -> ("queue ASI stage"=w10:refnum<queue>, "queue CAMERA"=w9:refnum<queue>, "queue DAQ"=w6:refnum<queue>, "queue valve"=w5:refnum<queue>, "queue piezo"=w11:refnum<queue>, "queue pump"=w7:refnum<queue>, "error out"=w1:errorcluster, "queue FPGA"=w4:refnum<queue>, "queue MAIN"=w8:refnum<queue>)  [unwired: 2 in]
  n18 = Unbundle By Name(T11 {"variant"=variant, "Instruction"=enum."Main_STOP"} ("Q_main_element")) -> ("Instruction"=w22:T18)
  n19 = control-ref of="Buffer list"() -> (w17:refnum<vi>)
  n20 = control-ref of="Probe list"() -> (w18:refnum<vi>)
  n21 = call "IMAQ Create"("Image Name"="Contrast", "Image Type"=w40, "error in (no error)"=w1) -> ("New Image"=w36:T5, "error out"=w37:errorcluster)  [unwired: 2 in]
  n22 = control-ref of="ROI manager"() -> (w32:refnum<vi>)
  n23 = control-ref of="Laser lines manager"() -> (w24:refnum<vi>)
  n24 = call "IMAQ Create"("Image Name"="ROI", "Image Type"=w39, "error in (no error)"=w37) -> ("New Image"=w35:T5, "error out"=w13:errorcluster)  [unwired: 2 in]
  n25 = while {
    tunnel: [w75] -> _
    tunnel: w8 -> [w75]
    tunnel: [w136] -> w45
    tunnel: [w135] -> w44
    shift-right: [w129] -> _
    shift-left: sgl 0.05 -> [w134]
    tunnel: w13 -> [w73]
    tunnel: w9 -> [w132]
    shift-right: [w126] -> _
    shift-left: T5 refnum ("New Image") -> [w127]
    tunnel: w36 -> [w125]
    tunnel: w35 -> [w124]
    shift-right: [w119] -> _
    shift-left: T9 {"405"=0.0, "488"=0.0, "561"=0.0, "641"=0.0, "BF"=0.0, "X"=0.0, "Y"=0.0, "Filter list"=1, "Exp time"=0.0, "Kinetic time"=0.0, "Gain"=0, "Step length (nm)"=0, "Total range (nm)"=0, "Scan illumination\n mode"=FALSE, "Dt (s)"=0, "# repetitions"=0} ("Global parameters") -> [w120]
    tunnel: w6 -> [w118]
    shift-right: [w117] -> _
    shift-left: T3 {"ASI"=FALSE, "DAQ"=FALSE, "Camera"=FALSE, "Pump"=FALSE, "Valve"=FALSE, "PiFoc"=FALSE, "FPGA"=FALSE} ("Initialization status") -> [w116]
    tunnel: w10 -> [w114]
    shift-right: [w111] -> _
    shift-left: cluster{dbl[], dbl[]}[] [] ("XY positions") -> [w112]
    tunnel: w32 -> [w110]
    tunnel: w11 -> [w108]
    tunnel: w26 -> [w107]
    shift-right: [w101] -> _
    shift-left: FALSE ("Error") -> [w102]
    tunnel: w24 -> [w94]
    tunnel: w22 -> [w93]
    tunnel: w5 -> [w91]
    tunnel: w7 -> [w92]
    shift-right: [w77] -> _
    shift-left: w21 -> [w89]
    tunnel: w18 -> [w86]
    tunnel: w17 -> [w85]
    tunnel: w4 -> [w72]
    stop <- w133 stop-if-true
    n26 = Dequeue Element(queue=w75, error in (no error)=w73) -> (element=w81:T11, error out=w84:errorcluster)  [unwired: 1 in, 2 out]
    n27 = call "MAIN_analyse_element.vi"("error in"=w84, "element"=w81) -> ("error out"=w83:errorcluster, 2:"Instruction"=w80:T18, "variant"=w82:variant, 6:"Instruction"=→"instruction":string)  [unwired: 6 in]
    n28 = Equal?(x=w80, y=w93) -> (x = y?=w133:bool)
    n29 = case shown="\"Main_save_XY\"" w80 {
      tunnel: w83 -> [w150 w166 w239 w250 w262 w298 w312 w326 w340 w354 w368 w378 w406 w436 w463 w490 w517 w544 w571 w579 w598 w627 w655 w669 w686 w701 w723 w740 w752 w777 w791 w809 w822 w858 w880 w894 w908 w927 w943 w957 w1022 w1105 w1165 w1191 w1241 w1271 w1276 w1315 w1336 w1370 w1384 w1509 w1539 w1564 w1592 w1615 w1645 w1661 w1692 w1779 w1924 w1942 w1975]
      tunnel: [w150 w160 w202 w247 w268 w296 w310 w325 w339 w353 w367 w376 w397 w424 w451 w478 w505 w532 w559 w575 w592 w650 w652 w665 w679 w703 w721 w738 w751 w776 w790 w807 w829 w862 w871 w893 w905 w922 w940 w970 w1035 w1092 w1151 w1182 w1237 w1259 w1275 w1303 w1325 w1369 w1421 w1508 w1537 w1554 w1591 w1599 w1644 w1654 w1696 w1778 w1923 w1938 w1988] -> w103
      tunnel: [T11 {"variant"=variant, "Instruction"=enum."Main_idle"} ("Q_main_element") w178 T11 {"variant"=variant, "Instruction"=enum."Main_initialize_Queue"} ("Q_main_element") w246 T11 {"variant"=variant, "Instruction"=enum."Main_idle"} ("Q_main_element") T11 {"variant"=variant, "Instruction"=enum."Main_not_acquiring"} ("Q_main_element") T11 {"variant"=variant, "Instruction"=enum."Main_not_acquiring"} ("Q_main_element") T11 {"variant"=variant, "Instruction"=enum."Main_not_acquiring"} ("Q_main_element") T11 {"variant"=variant, "Instruction"=enum."Main_not_acquiring"} ("Q_main_element") T11 {"variant"=variant, "Instruction"=enum."Main_not_acquiring"} ("Q_main_element") T11 {"variant"=variant, "Instruction"=enum."Main_not_acquiring"} ("Q_main_element") T11 {"variant"=variant, "Instruction"=enum."Main_not_acquiring"} ("Q_main_element") T11 {"variant"=variant, "Instruction"=enum."Main_idle"} ("Q_main_element") T11 {"variant"=variant, "Instruction"=enum."Main_idle"} ("Q_main_element") T11 {"variant"=variant, "Instruction"=enum."Main_idle"} ("Q_main_element") T11 {"variant"=variant, "Instruction"=enum."Main_idle"} ("Q_main_element") T11 {"variant"=variant, "Instruction"=enum."Main_idle"} ("Q_main_element") T11 {"variant"=variant, "Instruction"=enum."Main_idle"} ("Q_main_element") T11 {"variant"=variant, "Instruction"=enum."Main_idle"} ("Q_main_element") T11 {"variant"=variant, "Instruction"=enum."Main_acquiring"} ("Q_main_element") T11 {"variant"=variant, "Instruction"=enum."Main_not_acquiring"} ("Q_main_element") T11 {"variant"=variant, "Instruction"=enum."Main_acquiring"} ("Q_main_element") T11 {"variant"=variant, "Instruction"=enum."Main_not_acquiring"} ("Q_main_element") w664 w687 w702 w714 T11 {"variant"=variant, "Instruction"=enum."Main_not_acquiring"} ("Q_main_element") w742 w763 w789 w806 w831 w846 w870 w888 w903 w919 w939 w953 w1034 T11 {"variant"=variant, "Instruction"=enum."Main_stop_single_scan"} ("Q_main_element") w1155 w1185 w1235 w1250 w1273 T11 {"variant"=variant, "Instruction"=enum."Main_merFISH_illumination_parameters"} ("Q_main_element") T11 {"variant"=variant, "Instruction"=enum."Main_merFISH_illumination_parameters"} ("Q_main_element") w1356 w1420 w1512 w1528 w1555 w1576 w1607 w1637 w1655 w1695 w1777 w1922 w1948 T11 {"variant"=variant, "Instruction"=enum."Main_idle"} ("Q_main_element")] -> w137
      tunnel: "Exp time (s)" -> [_ w162 _ _ _ _ _ _ _ _ _ w382 _ _ _ _ _ _ _ _ _ _ _ w667 _ _ _ _ _ _ _ _ _ _ _ _ _ _ _ _ w1018 _ _ _ _ _ _ _ _ _ w1389 _ _ _ _ _ _ _ w1703 _ _ _ _]
      tunnel: [w153 w180 w245 w258 w277 w294 w308 w323 w337 w351 w365 w373 w400 w432 w459 w486 w513 w540 w567 w587 w614 w648 w663 w677 w693 w710 w718 w733 w759 w782 w797 w815 w833 w867 w887 w901 w915 w934 w950 w976 w1042 w1103 w1171 w1190 w1247 w1270 w1280 w1317 w1339 w1374 w1427 w1519 w1550 w1575 w1598 w1625 w1653 w1668 w1710 w1788 w1930 w1954 w1997] -> w129
      tunnel: w134 -> [w153 w180 w245 w258 w277 w294 w308 w323 w337 w351 w365 _ w400 w432 w459 w486 w513 w540 w567 w587 w614 w648 w663 w677 w693 w710 w722 w733 w759 w782 w797 w815 w833 w867 w887 w901 w915 w934 w950 w977 w1042 w1103 w1171 w1190 w1247 w1270 w1280 w1317 w1339 w1374 w1427 w1519 w1550 w1575 w1598 w1625 w1653 w1668 w1710 w1788 w1930 w1954 w1997]
      tunnel: w132 -> [_ w175 _ _ w272 _ _ _ _ _ _ _ w390 w417 w444 w471 w498 w525 w552 w576 _ _ w653 w666 _ w696 _ _ _ _ _ _ _ _ _ _ _ _ _ w954 w1032 _ w1157 _ _ _ _ _ _ _ w1397 _ _ _ _ _ _ _ w1676 _ _ w1945 w1985]
      tunnel: w82 -> [_ _ _ _ w283 w299 w313 w327 w341 w355 w369 w377 w407 w437 w464 w491 w518 w545 w572 _ _ _ _ _ _ _ w724 w741 _ _ _ _ _ _ _ _ w909 w926 _ _ _ w1108 _ _ _ _ _ _ _ _ _ _ w1536 w1563 w1587 w1614 w1643 _ w1691 w1776 _ _ _]
      tunnel: "Start acquisition" -> [_ _ _ w248 w265 _ _ _ _ _ _ _ w393 w420 w447 w474 w501 w528 w555 _ _ _ _ w668 w689 w697 w713 _ w748 w771 _ _ w830 w848 w874 w891 w904 w925 w941 w969 w1033 _ w1164 w1186 w1236 w1253 w1274 _ _ w1365 w1419 _ _ _ _ _ _ _ _ _ _ w1947 w1977]
      tunnel: "Image contrast" -> [_ _ _ _ _ _ _ _ _ _ _ _ _ _ _ _ _ _ _ w577 _ w623 _ _ _ _ _ _ _ _ _ _ _ _ _ _ _ _ _ w975 _ _ _ _ _ _ _ _ _ w1359 _ _ _ _ _ _ _ _ w1705 _ _ _ _]
      tunnel: w127 -> [w152 w179 w244 w257 w276 w293 w307 w322 w336 w350 w364 _ w399 w431 w458 w485 w512 w539 w566 w586 w612 w622 w661 w676 w692 w709 w720 w732 w758 w781 w796 w814 w832 w866 w886 w900 w914 w933 w949 w978 w1041 w1104 w1170 w1183 w1246 w1269 w1279 w1316 w1338 w1358 w1426 w1520 w1549 w1574 w1597 w1624 w1652 w1667 w1704 w1787 w1929 w1953 w1996]
      tunnel: [w152 w179 w244 w257 w276 w293 w307 w322 w336 w350 w364 w372 w399 w431 w458 w485 w512 w539 w566 w586 w612 w622 w661 w676 w692 w709 w720 w732 w758 w781 w796 w814 w832 w866 w886 w900 w914 w933 w949 w972 w1041 w1104 w1170 w1183 w1246 w1269 w1279 w1316 w1338 w1358 w1426 w1520 w1549 w1574 w1597 w1624 w1652 w1667 w1704 w1787 w1929 w1953 w1996] -> w126
      tunnel: w125 -> [_ _ _ _ _ _ _ _ _ _ _ _ _ _ _ _ _ _ _ _ _ w624 _ _ _ _ _ _ _ _ _ _ _ _ _ _ _ _ _ w974 _ w1106 _ _ _ _ _ _ _ w1360 _ _ _ _ _ _ _ _ w1706 _ _ _ w1992]
      tunnel: w124 -> [_ _ _ _ _ _ _ _ _ _ _ _ _ _ _ _ _ _ _ _ _ w625 _ _ _ _ _ _ _ _ _ _ _ _ _ _ _ _ _ w973 _ w1107 _ _ _ _ _ _ _ _ _ _ _ _ _ _ _ _ _ _ _ _ w1994]
      tunnel: "Saving path" -> [_ _ w235 _ _ _ _ _ _ _ _ _ _ _ _ _ _ _ _ _ _ _ _ _ _ _ _ _ _ _ _ _ _ _ _ _ _ _ _ w963 w1024 _ w1160 _ _ _ _ _ _ _ w1405 _ _ _ _ _ _ _ _ _ _ _ _]
      tunnel: "Sample name" -> [_ _ _ _ _ _ _ _ _ _ _ _ _ _ _ _ _ _ _ _ _ _ _ _ _ _ _ _ _ _ _ _ _ _ _ _ _ _ _ w962 w1023 _ w1161 _ _ _ _ _ _ _ w1404 _ _ _ _ _ _ _ _ _ _ _ _]
      tunnel: "N frames" -> [_ _ _ _ _ _ _ _ _ _ _ _ _ _ _ _ _ _ _ _ _ _ _ _ _ _ _ _ _ _ _ _ _ _ _ _ _ _ _ w961 _ _ _ _ _ _ _ _ _ _ _ _ _ _ _ _ _ _ _ _ _ _ _]
      tunnel: w120 -> [w151 w181 w242 w256 w280 w292 w306 w321 w335 w349 w363 w384 w405 w435 w462 w489 w516 w543 w570 w585 w608 w638 w660 w675 w683 w705 w719 w731 w760 w779 w799 w816 w835 w855 w883 w897 w913 w930 w947 w964 w1027 w1102 w1152 w1178 w1244 w1267 w1281 w1318 w1340 w1372 w1409 w1521 w1547 w1572 w1595 w1613 w1642 w1672 w1688 w1785 w1927 w1949 w1995]
      tunnel: [w151 w181 w242 w256 w280 w292 w306 w321 w335 w349 w363 w383 w405 w435 w462 w489 w516 w543 w570 w585 w610 w645 w660 w674 w683 w705 w717 w731 w760 w779 w799 w816 w835 w855 w883 w897 w913 w930 w947 w964 w1026 w1102 w1152 w1177 w1244 w1267 w1281 w1318 w1340 w1372 w1423 w1521 w1547 w1572 w1595 w1611 w1641 w1672 w1688 w1785 w1927 w1949 w1995] -> w119
      tunnel: w75 -> [_ w165 _ w251 w261 _ _ _ _ _ _ _ _ _ _ _ _ _ _ w578 _ _ w654 _ _ _ _ _ _ _ _ _ _ _ _ _ _ _ _ _ _ _ _ _ _ _ _ _ _ _ w1383 _ _ _ _ _ _ _ _ _ _ _ _]
      tunnel: w118 -> [_ w173 _ _ w271 _ _ _ _ _ _ _ w389 w416 w443 w470 w497 w524 w551 _ _ _ _ _ _ _ _ _ _ _ _ _ _ _ _ _ _ _ _ _ w1030 w1087 _ _ _ _ _ _ _ _ w1400 _ _ _ _ _ _ _ w1699 _ _ w1944 w1984]
      tunnel: w116 -> [w149 w156 w243 w252 w279 w291 w305 w320 w334 w348 w362 w375 w403 w434 w461 w488 w515 w542 w569 w582 w611 w649 w659 w671 w688 w706 w716 w730 w756 w780 w793 w817 w836 w854 w884 w898 w912 w929 w948 w968 w1038 w1101 w1167 w1189 w1245 w1268 w1282 w1319 w1341 w1373 w1411 w1522 w1548 w1573 w1596 w1622 w1650 w1671 w1707 w1786 w1928 w1950 w1991]
      tunnel: [w149 w156 w243 w252 w279 w289 w303 w319 w333 w347 w361 w374 w404 w433 w460 w487 w514 w541 w568 w582 w611 w649 w659 w671 w688 w706 w716 w730 w756 w780 w793 w817 w836 w854 w884 w898 w912 w929 w948 w968 w1038 w1101 w1167 w1189 w1245 w1268 w1282 w1319 w1341 w1373 w1410 w1522 w1548 w1573 w1596 w1622 w1650 w1671 w1707 w1786 w1928 w1950 w1991] -> w117
      tunnel: "VISA stage port :" -> [_ w177 _ _ _ _ _ _ _ _ _ _ _ _ _ _ _ _ _ _ _ _ _ _ _ _ _ _ _ _ _ _ _ _ _ _ _ _ _ _ _ _ _ _ _ _ _ _ _ _ _ _ _ _ _ _ _ _ _ _ _ _ _]
      tunnel: w114 -> [_ w176 _ _ w273 _ _ _ _ _ _ _ w391 w418 w445 w472 w499 w526 w553 _ _ _ _ _ _ _ _ _ w744 w767 w786 _ _ _ _ _ _ _ _ _ w1036 _ w1158 _ _ _ _ _ _ w1357 w1399 _ w1529 w1556 _ w1609 w1639 w1656 _ _ _ w1946 w1986]
      tunnel: w89 -> [w146 w158 w193 w253 w264 w286 w300 w314 w328 w342 w356 w379 w396 w423 w450 w477 w504 w531 w558 w580 w600 w635 w656 w670 w678 w704 w711 w727 w755 w766 w794 w812 w826 w863 w885 w899 w902 w928 w944 w967 w1017 w1094 w1166 w1181 w1238 w1264 w1278 w1310 w1331 w1349 w1394 w1518 w1540 w1565 w1584 w1606 w1636 w1660 w1684 w1773 w1917 w1937 w1976]
      tunnel: [w146 w158 w201 w253 w264 w286 w300 w314 w328 w342 w356 w379 w396 w423 w450 w477 w504 w531 w558 w580 w599 w634 w656 w670 w678 w704 w711 w727 w753 w765 w792 w810 w821 w859 w885 w899 w902 w928 w944 w958 w1017 w1094 w1166 w1176 w1238 w1258 w1277 w1308 w1330 w1348 w1388 w1518 w1540 w1565 w1584 w1604 w1634 w1660 w1684 w1773 w1917 w1937 w1976] -> w77
      tunnel: "ROI manager" -> [_ _ _ _ _ _ _ _ _ _ _ _ _ _ _ _ _ _ _ _ w596 w632 _ _ _ _ _ _ w747 w770 w783 w803 _ _ _ _ _ _ _ _ _ _ _ _ _ _ _ _ _ w1362 _ _ _ _ _ _ w1628 _ _ _ _ _ _]
      tunnel: w112 -> [w148 w174 w241 w255 w278 w288 w302 w318 w332 w346 w360 w381 w402 w430 w457 w484 w511 w538 w565 w584 _ _ w658 w673 w691 w708 w715 w729 _ _ w798 _ w837 w865 w882 w896 w911 w932 w946 w966 w1039 w1100 w1169 w1188 w1243 w1266 w1283 w1320 w1342 w1364 w1424 w1523 w1546 w1571 w1594 _ _ w1670 w1708 w1784 w1926 w1951 w1990]
      tunnel: [w148 w174 w241 w255 w278 w288 w302 w318 w332 w346 w360 w381 w402 w430 w457 w484 w511 w538 w565 w584 w593 w630 w658 w673 w691 w708 w715 w729 w750 w762 w798 w800 w837 w865 w882 w896 w911 w932 w946 w966 w1039 w1100 w1169 w1188 w1243 w1266 w1283 w1320 w1342 w1368 w1424 w1523 w1546 w1571 w1594 w1608 w1638 w1670 w1708 w1784 w1926 w1951 w1990] -> w111
      tunnel: w110 -> [_ _ w236 _ _ _ _ _ _ _ _ _ _ _ _ _ _ _ _ _ _ _ _ _ _ _ _ _ w746 w769 w784 w802 w824 _ _ _ _ _ _ _ _ _ _ _ _ _ _ _ _ w1361 _ _ _ _ _ w1612 _ _ w1681 _ _ _ w1972]
      tunnel: "Illumination controls" -> [_ _ _ _ _ _ _ _ _ _ _ _ _ _ _ _ _ _ _ _ w609 w639 _ _ _ _ _ _ _ _ _ _ _ _ _ _ _ _ _ _ _ _ _ _ _ _ _ _ _ _ _ _ _ _ _ _ _ _ _ _ _ _ _]
      tunnel: w108 -> [_ w172 _ _ w274 _ _ _ _ _ _ _ w392 w419 w446 w473 w500 w527 w554 _ _ _ _ _ _ _ _ _ _ _ _ _ _ w850 w873 w890 _ _ _ _ w1037 w1088 w1159 _ _ _ _ _ _ _ w1398 w1514 w1530 w1557 _ w1610 w1640 w1657 w1675 _ _ w1941 w1987]
      tunnel: w107 -> [_ _ _ _ _ _ _ _ _ _ _ _ _ _ _ _ _ _ _ _ _ _ _ _ _ _ _ _ _ _ _ _ _ _ _ _ _ _ _ _ _ _ _ _ _ _ _ _ _ _ _ _ _ _ _ _ _ _ _ _ _ _ w1982]
      tunnel: w102 -> [w147 _ w240 w254 _ w287 w301 w315 w329 w343 w357 w380 _ _ _ _ _ _ _ w583 w601 w636 w657 w672 w690 w707 w712 w728 w757 w778 w795 w813 w827 w864 w881 w895 w910 w931 w945 w965 w1040 w1099 w1168 w1187 w1242 w1265 w1284 w1321 w1343 w1371 w1425 w1524 w1545 w1570 w1593 w1623 w1651 w1669 w1709 w1783 w1925 w1952 w1980]
      tunnel: [w147 FALSE ("Error") w240 w254 TRUE ("Error") w287 w301 w315 w329 w343 w357 w380 TRUE ("Error") TRUE ("Error") TRUE ("Error") TRUE ("Error") TRUE ("Error") TRUE ("Error") TRUE ("Error") w583 w601 w636 w657 w672 w690 w707 w712 w728 w757 w778 w795 w813 w827 w864 w881 w895 w910 w931 w945 w965 w1040 w1099 w1168 w1187 w1242 w1265 w1284 w1321 w1343 w1371 w1425 w1524 w1545 w1570 w1593 w1623 w1651 w1669 w1709 w1783 w1925 w1952 w1980] -> w101
      tunnel: "Illumination source" -> [_ _ _ _ _ _ _ _ _ _ _ _ _ _ _ _ _ _ _ _ _ _ _ _ _ _ _ _ _ _ _ _ _ _ _ _ _ _ _ _ w1010 _ w1163 w1179 _ _ _ _ _ _ w1377 _ _ _ _ _ _ _ _ _ _ _ _]
      tunnel: "Select laser lines" -> [_ _ _ _ _ _ _ _ _ _ _ _ _ _ _ _ _ _ _ _ _ _ _ _ _ _ _ _ _ _ _ _ _ _ _ _ _ _ _ _ _ _ _ w1184 _ _ _ _ _ _ _ _ _ _ _ _ _ _ _ _ _ _ _]
      tunnel: "Brightfield intensity" -> [_ _ _ _ _ _ _ _ _ _ _ _ _ _ _ _ _ _ _ _ _ _ _ _ _ _ _ _ _ _ _ _ _ _ _ _ _ _ _ _ w1019 _ _ _ _ _ _ _ _ _ w1422 _ _ _ _ _ _ _ _ _ _ _ _]
      tunnel: "step length (nm)" -> [_ _ _ _ _ _ _ _ _ _ _ _ _ _ _ _ _ _ _ _ _ _ _ _ w682 _ _ _ _ _ _ _ _ _ _ _ _ _ _ _ w1028 _ _ _ _ _ _ _ _ _ w1406 _ _ _ _ _ _ _ _ _ _ _ _]
      tunnel: "Total  range (nm)" -> [_ _ _ _ _ _ _ _ _ _ _ _ _ _ _ _ _ _ _ _ _ _ _ _ w681 _ _ _ _ _ _ _ _ _ _ _ _ _ _ _ w1029 _ _ _ _ _ _ _ _ _ w1407 _ _ _ _ _ _ _ _ _ _ _ _]
      tunnel: w94 -> [_ _ _ _ _ _ _ _ _ _ _ _ _ _ _ _ _ _ _ _ _ _ _ _ _ _ _ _ _ _ _ _ _ _ _ _ _ _ _ _ _ _ w1162 _ _ _ _ w1312 w1333 _ _ _ _ _ _ _ _ _ w1689 _ _ _ w1974]
      tunnel: w92 -> [_ w168 _ _ w266 _ _ _ _ _ _ _ w387 w414 w441 w468 w495 w522 w549 _ _ _ _ _ _ _ _ _ _ _ _ _ _ _ _ _ _ _ _ _ _ _ _ _ _ _ _ _ _ _ w1402 _ _ _ w1577 _ _ _ _ _ w1910 w1940 w1978]
      tunnel: w91 -> [_ w169 _ _ w267 _ _ _ _ _ _ _ w388 w415 w442 w469 w496 w523 w550 _ _ _ _ _ _ _ _ _ _ _ _ _ _ _ _ _ _ w924 w938 _ _ _ _ _ _ _ _ _ _ _ w1401 _ w1527 w1553 w1578 _ _ _ _ _ w1911 _ w1979]
      tunnel: "VISA valve port :" -> [_ w170 _ _ _ _ _ _ _ _ _ _ _ _ _ _ _ _ _ _ _ _ _ _ _ _ _ _ _ _ _ _ _ _ _ _ _ _ _ _ _ _ _ _ _ _ _ _ _ _ _ _ _ _ _ _ _ _ _ _ _ _ _]
      tunnel: "Measure QPD" -> [_ w167 _ _ _ _ _ _ _ _ _ _ _ _ _ _ _ _ _ _ _ _ _ _ _ _ _ _ _ _ _ _ _ w843 w875 w892 _ _ _ _ w1008 _ w1154 _ _ _ w1272 _ _ _ w1390 _ w1535 w1562 _ _ _ w1664 _ _ _ w1934 _]
      tunnel: "Valve H" -> [_ _ _ _ _ _ _ _ _ _ _ _ _ _ _ _ _ _ _ _ _ _ _ _ _ _ _ _ _ _ _ _ _ _ _ _ _ _ _ _ _ _ _ _ _ _ _ _ _ _ w1395 _ _ _ w1586 _ _ _ _ _ w1918 _ _]
      tunnel: w86 -> [_ _ _ _ _ _ _ _ _ _ _ _ _ _ _ _ _ _ _ _ _ _ _ _ _ _ _ _ _ _ _ _ _ _ _ _ _ _ _ _ _ _ _ _ w1240 _ _ w1311 w1332 _ w1379 _ _ _ w1585 _ _ _ w1680 _ _ _ w1970]
      tunnel: w85 -> [_ _ _ _ _ _ _ _ _ _ _ _ _ _ _ _ _ _ _ _ _ _ _ _ _ _ _ _ _ _ _ _ _ _ _ _ _ _ _ _ _ _ _ _ w1239 w1254 _ _ _ _ _ _ _ _ _ _ _ _ _ _ _ _ w1968]
      tunnel: "N movies" -> [_ _ _ _ _ _ _ _ _ _ _ _ _ _ _ _ _ _ _ _ _ _ _ _ _ _ _ _ _ _ _ _ _ _ _ _ _ _ _ w960 _ _ _ _ _ _ _ _ _ _ _ _ _ _ _ _ _ _ _ _ _ _ _]
      tunnel: "Close LabView?" -> [_ _ _ _ _ _ _ _ _ _ _ _ _ _ _ _ _ _ _ _ _ _ _ _ _ _ _ _ _ _ _ _ _ _ _ _ _ _ _ _ _ _ _ _ _ _ _ _ _ _ _ _ _ _ _ _ _ _ _ _ _ w1936 _]
      tunnel: "Display?" -> [_ _ _ _ _ _ _ _ _ _ _ _ _ _ _ _ _ _ _ _ _ _ _ _ _ _ _ _ _ _ _ _ _ _ _ _ _ _ _ _ w1007 w1086 _ _ _ _ _ _ _ _ _ _ _ _ _ _ _ _ w1677 _ _ _ _]
      tunnel: w72 -> [_ w155 _ _ w259 _ _ _ _ _ _ _ w386 w413 w440 w467 w494 w521 w548 _ _ _ _ _ _ _ _ _ _ _ _ _ _ w845 w872 w889 _ _ _ _ w1009 _ w1156 _ _ _ _ _ _ _ w1376 w1510 _ _ _ _ _ _ _ _ _ w1935 w1967]
      tunnel: "merFISH mode" -> [_ _ _ _ _ _ _ _ _ _ _ _ _ _ _ _ _ _ _ _ _ _ _ _ _ _ _ _ _ _ _ _ _ _ _ _ _ _ _ _ _ _ _ _ _ _ _ _ _ _ w1375 _ _ _ _ w1601 _ _ _ _ _ _ _]
      frame "Main_idle", Default {
      }
      frame "Main_initialize" {
        n30 = Flush Queue(queue=w165, error in (no error)=w166) -> (error out=w163:errorcluster)  [unwired: 2 out]
        n31 = call <vilib>:"Set Busy.vi"("error in (no error)"=w163) -> ("error out"=w157:errorcluster)  [unwired: 9 in, 1 out]
        n32 = control-ref of="Autofocus lost"() -> (w164:refnum<vi>)
        n33 = call "MAIN_merFISH_initialization.vi"("queue DAQ"=w173, "queue ASI stage"=w176, "Measure QPD"=w167, "queue CAMERA"=w175, "VISA stage port"=w177, "queue FPGA"=w155, "error in"=w157, "queue valve"=w169, "queue pump"=w168, "Initialization status"=w156, "queue piezo"=w172, "Exp time (s)"=w162, "VISA resource Valve"=w170, "Autofocus lost Refnum"=w164) -> ("error out"=w159:errorcluster)  [unwired: 5 in]
        n34 = First Call?() -> (First Call?: T/F=w161:bool)
        n35 = case shown="False" w161 {
          tunnel: [T11 {"variant"=variant, "Instruction"=enum."Main_not_acquiring"} ("Q_main_element") T11 {"variant"=variant, "Instruction"=enum."Main_initialize_TDMS"} ("Q_main_element")] -> w178
          tunnel: [w182 w185] -> w160
          tunnel: w159 -> [w183 w185]
          frame False {
            n36 = call <vilib>:"Unset Busy.vi"("error in (no error)"=w183) -> ("error out"=w182:errorcluster)  [unwired: 10 in]
          }
          frame True {
          }
        }
      }
      frame "Main_initialize_TDMS" {
        n37 = call "MAIN_load_previous_acquisition_data.vi"("error in"=w239, "Path to the saving folder"=w235) -> ("error out"=w233:errorcluster, "Data cluster"=w215:T30, "Menu names cluster"=w227:T31)  [unwired: 1 in]
        n38 = Unbundle By Name(w215) -> ("REFs"=w190:dbl[][], "Brightfield intensity"=w196:dbl, "FOV size"=w197:dbl, "Sample name"=w208:string, "QPD ref.X"=w210:sgl, "Alert email adress"=w192:string, "Total  range (nm)"=w221:u32, "Exp time (s)"=w220:sgl, "step length (nm)"=w219:u32, "ROIs"=w218:dbl[][])
        n39 = Unbundle By Name(w215) -> ("merFISH path"=w200:path, "Laser lines array"=w214:dbl[][], "Hybridization procedure"=w213:i32[][], "Photobleaching procedure"=w212:i32[][], "merFISH cluster"=w211:T6, "QPD ref"=w209:T32, "PID gains"=w195:T2, "Illumination source"=w194:bool, "N movies"=w188:i32, "N frames"=w187:i32, "Mosaic size"=w189:u16[])
        n40 = Unbundle By Name(w227) -> ("Laser names"=w226:string[], "Buffer list names"=w225:string[][], "Probe list names"=w224:string[][], "Hybridization name"=w223:string[], "Photobleaching name"=w222:string[])
        n41 = property on="Laser lines manager" class="LstBox (strict)"(error in=w233, "Item Names"=w226) -> (error out=w232:errorcluster)  [unwired: 1 in, 1 out]
        n42 = local write "Brightfield intensity"(w196) -> ()
        n43 = local write "FOV size (um)"(w197) -> ()
        n44 = local write "Sample name"(w208) -> ()
        n45 = local write "merFISH setpoint"(w210) -> ()
        n46 = local write "Total  range (nm)"(w221) -> ()
        n47 = local write "Exp time (s)"(w220) -> ()
        n48 = local write "step length (nm)"(w219) -> ()
        n49 = Array Size(array=w218) -> (size(s)=w217:i32[])
        n50 = local write "PID gains"(w195) -> ()
        n51 = local write "Illumination source"(w194) -> ()
        n52 = local write "N movies"(w188) -> ()
        n53 = local write "N frames"(w187) -> ()
        n54 = Index Array(array=w189, index #1=0 ("index"), index #2=1 ("index")) -> (element #1=w205:u16, element #2=w204:u16)
        n55 = Index Array(array=w217, index=0) -> (element=w216:i32)
        n56 = To Long Integer(number=w204) -> (32bit integer=w198:i32)
        n57 = To Long Integer(number=w205) -> (32bit integer=w199:i32)
        n58 = local write "Mosaic size X"(w199) -> ()
        n59 = local write "Mosaic size Y"(w198) -> ()
        n60 = property on="Buffer list" class="MCListbox (strict)"(error in=w232, "ItemNames"=w225) -> (error out=w231:errorcluster)  [unwired: 1 in, 1 out]
        n61 = Insert Into Array(array=w218, index (row)=w216, new element=dbl[][] [[0.0, 0.0, -1.0]] ("Laser lines array")) -> (w191:dbl[][])  [unwired: 1 in]
        n62 = property on="Probe list" class="MCListbox (strict)"(error in=w231, "ItemNames"=w224) -> (error out=w230:errorcluster)  [unwired: 1 in, 1 out]
        n63 = Bundle By Name(cluster=w193, "merFISH path"=w200, "Laser lines array"=w214, "Hybridization procedure"=w213, "Photobleaching procedure"=w212, "merFISH init"=w211, "QPD ref"=w209, "REF positions"=w190, "XY positions"=w191) -> (w201:T16)
        n64 = global write "Global_MAIN.vi" "Alert email adress"(w192) -> ()
        n65 = local write "Alert email adress"(w192) -> ()
        n66 = property on="Hybridization manager" class="LstBox (strict)"(error in=w230, "Item Names"=w223) -> (error out=w229:errorcluster)  [unwired: 1 in, 1 out]
        n67 = property on="Photobleaching manager" class="LstBox (strict)"(error in=w229, "Item Names"=w222) -> (error out=w228:errorcluster)  [unwired: 1 in, 1 out]
        n68 = call "ROI_edit_ROI_manager.vi"("error in"=w228, "XY positions"=w191, "ROI Refnum"=w236) -> ("error out"=w203:errorcluster)  [unwired: 2 in]
        n69 = call <vilib>:"Unset Busy.vi"("error in (no error)"=w203) -> ("error out"=w202:errorcluster)  [unwired: 10 in]
      }
      frame "Main_initialize_Queue" {
        n70 = Unbundle By Name(w252) -> ("Camera"=w249:bool)
        n71 = call "MAIN_init_queue.vi"("Camera"=w249, "error in"=w250, "queue MAIN"=w251, "Start acquisition"=w248) -> ("error out"=w247:errorcluster, "Next task"=w246:T11)  [unwired: 2 in]
      }
      frame "Main_error" {
        n72 = Flush Queue(queue=w261, error in (no error)=w262) -> (error out=w260:errorcluster)  [unwired: 2 out]
        n73 = Variant To Data(error in=w260, type=errorcluster {"status"=FALSE, "code"=0, "source"=""} ("error out"), Variant=w283) -> (data=→"MAIN_consumer":errorcluster, error out=w275:errorcluster)
        n74 = call "MAIN_error_handling.vi"("queue FPGA"=w259, "Start acquisition"=w265, "queue pump"=w266, "error in"=w275, "queue valve"=w267, "queue piezo"=w274, "queue camera"=w272, "queue ASI stage"=w273, "queue DAQ"=w271) -> ("error out"=w269:errorcluster)  [unwired: 2 in]
        n75 = flat-sequence {
          tunnel: w269 -> [w284]
          tunnel: [w284] -> w268
          frame #0 {
            w285 = FALSE ("Autofocus")
            n76 = local write "Measure QPD"(w285) -> ()
            n77 = local write "Autofocus"(w285) -> ()
            n78 = local write "Start acquisition"(w285) -> ()
          }
        }
      }
      frame "Main_DAQ_initialization_results" {
        n79 = Variant To Data(error in=w298, type=FALSE, Variant=w299) -> (data=w290:bool, error out=w296:errorcluster)
        n80 = Bundle By Name(cluster=w291, "DAQ"=w290) -> (w289:T3)
      }
      frame "Main_ASI_initialization_results" {
        n81 = Variant To Data(error in=w312, type=FALSE, Variant=w313) -> (data=w304:bool, error out=w310:errorcluster)
        n82 = Bundle By Name(cluster=w305, "ASI"=w304) -> (w303:T3)
      }
      frame "Main_Piezo_initialization_results" {
        n83 = Variant To Data(error in=w326, type=FALSE ("PiFoc Connected"), Variant=w327) -> (data=w316:bool, error out=w325:errorcluster)
        n84 = Bundle By Name(cluster=w320, "PiFoc"=w316) -> (w319:T3)
      }
      frame "Main_Valve_initialization_results" {
        n85 = Variant To Data(error in=w340, type=FALSE ("PiFoc Connected"), Variant=w341) -> (data=w330:bool, error out=w339:errorcluster)
        n86 = Bundle By Name(cluster=w334, "Valve"=w330) -> (w333:T3)
      }
      frame "Main_Pump_initialization_results" {
        n87 = Variant To Data(error in=w354, type=FALSE ("PiFoc Connected"), Variant=w355) -> (data=w344:bool, error out=w353:errorcluster)
        n88 = Bundle By Name(cluster=w348, "Pump"=w344) -> (w347:T3)
      }
      frame "Main_FPGA_initialization_results" {
        n89 = Variant To Data(error in=w368, type=FALSE ("PiFoc Connected"), Variant=w369) -> (data=w358:bool, error out=w367:errorcluster)
        n90 = Bundle By Name(cluster=w362, "FPGA"=w358) -> (w361:T3)
      }
      frame "Main_CAMERA_initialization_results" {
        n91 = call "MAIN_camera_initialization_results.vi"("error in"=w378, "variant"=w377) -> ("error out"=w376:errorcluster, "Error"=w370:bool, "Cooler status"=w371:bool, "Real time image"=w372:T5, "Total kinetic time (s)"=w373:sgl)  [unwired: 2 in]
        n92 = local write "Cooler ON?"(w371) -> ()
        n93 = Bundle By Name(cluster=w375, "Camera"=w370) -> (w374:T3)
        n94 = Bundle By Name(cluster=w384, "Kinetic time"=w373, "Exp time"=w382) -> (w383:T9)
      }
      frame "Main_DAQ_error" {
        n95 = Variant To Data(error in=w406, type=errorcluster {"status"=FALSE, "code"=0, "source"=""} ("error out"), Variant=w407) -> (data=→"DAQ":errorcluster, error out=w395:errorcluster)
        n96 = Bundle By Name(cluster=w403, "DAQ"=FALSE ("ASI stage connected")) -> (w404:T3)
        n97 = call "MAIN_error_handling.vi"("queue FPGA"=w386, "Start acquisition"=w393, "queue pump"=w387, "error in"=w395, "queue valve"=w388, "queue piezo"=w392, "queue camera"=w390, "queue ASI stage"=w391, "queue DAQ"=w389) -> ("error out"=w394:errorcluster)  [unwired: 2 in]
        n98 = flat-sequence {
          tunnel: [w411] -> w397
          tunnel: w394 -> [w411]
          frame #0 {
            w412 = FALSE ("Autofocus")
            n99 = local write "Measure QPD"(w412) -> ()
            n100 = local write "Autofocus"(w412) -> ()
            n101 = local write "Start acquisition"(w412) -> ()
          }
        }
      }
      frame "Main_ASI_error" {
        n102 = Variant To Data(error in=w436, type=errorcluster {"status"=FALSE, "code"=0, "source"=""} ("error out"), Variant=w437) -> (data=→"ASI":errorcluster, error out=w422:errorcluster)
        n103 = Bundle By Name(cluster=w434, "ASI"=FALSE ("ASI stage connected")) -> (w433:T3)
        n104 = call "MAIN_error_handling.vi"("queue FPGA"=w413, "Start acquisition"=w420, "queue pump"=w414, "error in"=w422, "queue valve"=w415, "queue piezo"=w419, "queue camera"=w417, "queue ASI stage"=w418, "queue DAQ"=w416) -> ("error out"=w421:errorcluster)  [unwired: 2 in]
        n105 = flat-sequence {
          tunnel: [w438] -> w424
          tunnel: w421 -> [w438]
          frame #0 {
            w439 = FALSE ("Autofocus")
            n106 = local write "Measure QPD"(w439) -> ()
            n107 = local write "Autofocus"(w439) -> ()
            n108 = local write "Start acquisition"(w439) -> ()
          }
        }
      }
      frame "Main_Piezo_error" {
        n109 = Variant To Data(error in=w463, type=errorcluster {"status"=FALSE, "code"=0, "source"=""} ("error out"), Variant=w464) -> (data=→"Piezo":errorcluster, error out=w448:errorcluster)
        n110 = Bundle By Name(cluster=w461, "PiFoc"=FALSE ("ASI stage connected")) -> (w460:T3)
        n111 = call "MAIN_error_handling.vi"("queue FPGA"=w440, "Start acquisition"=w447, "queue pump"=w441, "error in"=w448, "queue valve"=w442, "queue piezo"=w446, "queue camera"=w444, "queue ASI stage"=w445, "queue DAQ"=w443) -> ("error out"=w449:errorcluster)  [unwired: 2 in]
        n112 = flat-sequence {
          tunnel: [w465] -> w451
          tunnel: w449 -> [w465]
          frame #0 {
            w466 = FALSE ("Autofocus")
            n113 = local write "Measure QPD"(w466) -> ()
            n114 = local write "Autofocus"(w466) -> ()
            n115 = local write "Start acquisition"(w466) -> ()
          }
        }
      }
      frame "Main_CAMERA_error" {
        n116 = Variant To Data(error in=w490, type=errorcluster {"status"=FALSE, "code"=0, "source"=""} ("error out"), Variant=w491) -> (data=→"sCMOS":errorcluster, error out=w476:errorcluster)
        n117 = Bundle By Name(cluster=w488, "Camera"=FALSE ("ASI stage connected")) -> (w487:T3)
        n118 = call "MAIN_error_handling.vi"("queue FPGA"=w467, "Start acquisition"=w474, "queue pump"=w468, "error in"=w476, "queue valve"=w469, "queue piezo"=w473, "queue camera"=w471, "queue ASI stage"=w472, "queue DAQ"=w470) -> ("error out"=w475:errorcluster)  [unwired: 2 in]
        n119 = flat-sequence {
          tunnel: w475 -> [w492]
          tunnel: [w492] -> w478
          frame #0 {
            w493 = FALSE ("Autofocus")
            n120 = local write "Measure QPD"(w493) -> ()
            n121 = local write "Autofocus"(w493) -> ()
            n122 = local write "Start acquisition"(w493) -> ()
          }
        }
      }
      frame "Main_Valve_error" {
        n123 = Variant To Data(error in=w517, type=errorcluster {"status"=FALSE, "code"=0, "source"=""} ("error out"), Variant=w518) -> (data=→"Valve":errorcluster, error out=w503:errorcluster)
        n124 = Bundle By Name(cluster=w515, "Valve"=FALSE ("ASI stage connected")) -> (w514:T3)
        n125 = call "MAIN_error_handling.vi"("queue FPGA"=w494, "Start acquisition"=w501, "queue pump"=w495, "error in"=w503, "queue valve"=w496, "queue piezo"=w500, "queue camera"=w498, "queue ASI stage"=w499, "queue DAQ"=w497) -> ("error out"=w502:errorcluster)  [unwired: 2 in]
        n126 = flat-sequence {
          tunnel: w502 -> [w519]
          tunnel: [w519] -> w505
          frame #0 {
            w520 = FALSE ("Autofocus")
            n127 = local write "Measure QPD"(w520) -> ()
            n128 = local write "Autofocus"(w520) -> ()
            n129 = local write "Start acquisition"(w520) -> ()
          }
        }
      }
      frame "Main_Pump_error" {
        n130 = Variant To Data(error in=w544, type=errorcluster {"status"=FALSE, "code"=0, "source"=""} ("error out"), Variant=w545) -> (data=→"Pump":errorcluster, error out=w530:errorcluster)
        n131 = Bundle By Name(cluster=w542, "Pump"=FALSE ("ASI stage connected")) -> (w541:T3)
        n132 = call "MAIN_error_handling.vi"("queue FPGA"=w521, "Start acquisition"=w528, "queue pump"=w522, "error in"=w530, "queue valve"=w523, "queue piezo"=w527, "queue camera"=w525, "queue ASI stage"=w526, "queue DAQ"=w524) -> ("error out"=w529:errorcluster)  [unwired: 2 in]
        n133 = flat-sequence {
          tunnel: w529 -> [w546]
          tunnel: [w546] -> w532
          frame #0 {
            w547 = FALSE ("Autofocus")
            n134 = local write "Measure QPD"(w547) -> ()
            n135 = local write "Autofocus"(w547) -> ()
            n136 = local write "Start acquisition"(w547) -> ()
          }
        }
      }
      frame "Main_FPGA_error" {
        n137 = Variant To Data(error in=w571, type=errorcluster {"status"=FALSE, "code"=0, "source"=""} ("error out"), Variant=w572) -> (data=→"FPGA":errorcluster, error out=w557:errorcluster)
        n138 = Bundle By Name(cluster=w569, "FPGA"=FALSE ("ASI stage connected")) -> (w568:T3)
        n139 = call "MAIN_error_handling.vi"("queue FPGA"=w548, "Start acquisition"=w555, "queue pump"=w549, "error in"=w557, "queue valve"=w550, "queue piezo"=w554, "queue camera"=w552, "queue ASI stage"=w553, "queue DAQ"=w551) -> ("error out"=w556:errorcluster)  [unwired: 2 in]
        n140 = flat-sequence {
          tunnel: w556 -> [w573]
          tunnel: [w573] -> w559
          frame #0 {
            w574 = FALSE ("Autofocus")
            n141 = local write "Measure QPD"(w574) -> ()
            n142 = local write "Autofocus"(w574) -> ()
            n143 = local write "Start acquisition"(w574) -> ()
          }
        }
      }
      frame "Main_start_acquiring" {
        n144 = call "MAIN_start_acquiring.vi"("error in"=w579, "queue MAIN"=w578, "Image contrast"=w577, "queue CAMERA"=w576) -> ("error out"=w575:errorcluster)  [unwired: 3 in]
      }
      frame "Main_not_acquiring" {
        n145 = Unbundle By Name(w600) -> ("XY positions"=w595:dbl[][])
        n146 = control-ref of="XY positions"() -> (w597:refnum<vi>)
        n147 = call "MAIN_check_XY_stage_positions.vi"("Update display properties?"=FALSE, "error in"=w598, 7:"XY positions"=w597, "ROI manager"=w596, 9:"XY positions"=w595) -> ("error out"=w592:errorcluster, "XYZ"=w591:cluster{"x(um)":dbl, "y(um)":dbl, "z(um)":dbl}, "XY positions OUT"=w594:dbl[][], "XY graph"=w593:cluster{dbl[], dbl[]}[])  [unwired: 1 in]
        n148 = Bundle By Name(cluster=w600, "XY positions"=w594) -> (w599:T16)
        n149 = Unbundle By Name(w609) -> ("BF"=w606:dbl, "641"=w605:dbl, "561"=w604:dbl, "488"=w603:dbl, "405"=w602:dbl)
        n150 = Bundle By Name(cluster=w608, "BF"=w606, "641"=w605, "561"=w604, "488"=w603, "405"=w602) -> (w607:T9)
        n151 = Unbundle By Name(w591) -> ("x(um)"=w590:dbl, "y(um)"=w589:dbl)
        n152 = Bundle By Name(cluster=w607, "X"=w590, "Y"=w589) -> (w610:T9)
      }
      frame "Main_acquiring" {
        n153 = property on="Image" class="ImageControl"(error in=w627) -> (error out=w626:errorcluster, "ROI"=w628:T33)  [unwired: 1 in, 1 out]
        n154 = call "MAIN_display_new_image.vi"("ROI"=w628, "Real time image"=w622, "error in"=w626, "ROI Image"=w625, "Contrast image"=w624, "Image contrast"=w623) -> ("error out"=w618:errorcluster, "ROI"=→"ROI":T5, "Image"=→"Image":T5, "Intensity range"=→"Intensity range":cluster{sgl, sgl})
        n155 = Unbundle By Name(w639) -> ("BF"=w644:dbl, "641"=w643:dbl, "561"=w642:dbl, "488"=w641:dbl, "405"=w640:dbl)
        n156 = Bundle By Name(cluster=w638, "BF"=w644, "641"=w643, "561"=w642, "488"=w641, "405"=w640) -> (w637:T9)
        n157 = Unbundle By Name(w635) -> ("XY positions"=w631:dbl[][])
        n158 = control-ref of="XY positions"() -> (w633:refnum<vi>)
        n159 = call "MAIN_check_XY_stage_positions.vi"("Update display properties?"=FALSE, "error in"=w618, 7:"XY positions"=w633, "ROI manager"=w632, 9:"XY positions"=w631) -> ("error out"=w629:errorcluster, "XYZ"=w616:cluster{"x(um)":dbl, "y(um)":dbl, "z(um)":dbl}, "XY positions OUT"=w617:dbl[][], "XY graph"=w630:cluster{dbl[], dbl[]}[])  [unwired: 1 in]
        n160 = Bundle By Name(cluster=w635, "XY positions"=w617) -> (w634:T16)
        n161 = Unbundle By Name(w616) -> ("x(um)"=w647:dbl, "y(um)"=w646:dbl)
        n162 = call <vilib>:"Simple Error Handler.vi"("error in (no error)"=w629) -> ("error out"=w650:errorcluster)  [unwired: 4 in, 4 out]
        n163 = Bundle By Name(cluster=w637, "X"=w647, "Y"=w646) -> (w645:T9)
      }
      frame "Main_stop_acquiring" {
        n164 = call "MAIN_stop_acquiring.vi"("error in"=w655, "queue MAIN"=w654, "queue CAMERA"=w653) -> ("error out"=w652:errorcluster)  [unwired: 2 in]
      }
      frame "Main_change_exposure" {
        n165 = Bundle By Name(cluster=w675, "Exp time"=w667) -> (w674:T9)
        n166 = call "MAIN_change_exposure_time.vi"("error in"=w669, "Start acquisition"=w668, "Exp time (s)"=w667, "queue CAMERA"=w666) -> ("error out"=w665:errorcluster, "Next task"=w664:T11)  [unwired: 2 in]
      }
      frame "Main_change_z_scan_parameters" {
        n167 = Build Array(w682, w681) -> (w680:u32[])
        n168 = To Variant(anything=w680) -> (Variant=w685:variant)
        n169 = call "MAIN_save_parameters_TDMS.vi"("error in"=w686, "Data"=w685, "Channel name"="Scan parameters" ("group name")) -> ("error out"=w679:errorcluster)  [unwired: 2 in]
        n170 = case shown="True" w689 {
          tunnel: [T11 {"variant"=variant, "Instruction"=enum."Main_not_acquiring"} ("Q_main_element") T11 {"variant"=variant, "Instruction"=enum."Main_acquiring"} ("Q_main_element")] -> w687
          frame False {
          }
          frame True {
          }
        }
      }
      frame "Main_define_ROI" {
        n171 = property on="Image" class="ImageControl"(error in=w701) -> (error out=w700:errorcluster, "ROI"=w699:T33)  [unwired: 1 in, 1 out]
        n172 = call "MAIN_define_or_reset_ROI.vi"("ROI"=w699, "error in"=w700, "Reset roi"="Reset roi", "Start acquisition"=w697, "queue CAMERA"=w696) -> ("error out"=w703:errorcluster, "Next task"=w702:T11)  [unwired: 2 in]
      }
      frame "Main_read_kinetic_time" {
        n173 = Variant To Data(error in=w723, type=w722, Variant=w724) -> (data=w718:sgl, error out=w721:errorcluster)
        n174 = Bundle By Name(cluster=w719, "Kinetic time"=w718) -> (w717:T9)
        n175 = case shown="False" w713 {
          tunnel: [T11 {"variant"=variant, "Instruction"=enum."Main_not_acquiring"} ("Q_main_element") T11 {"variant"=variant, "Instruction"=enum."Main_acquiring"} ("Q_main_element")] -> w714
          frame False {
          }
          frame True {
          }
        }
      }
      frame "Main_read_temperature" {
        n176 = Variant To Data(error in=w740, type=cluster{"temperature":sgl, bool} {"temperature"=0.0, FALSE} ("output cluster"), Variant=w741) -> (data=w737:cluster{"temperature":sgl, bool}, error out=w738:errorcluster)
        n177 = Unbundle(w737) -> ("temperature"=→"Sensor Temperature (°C)":sgl, →"Cooler ON?":bool)
      }
      frame "Main_save_XY" {
        n178 = Unbundle By Name(w755) -> ("XY positions"=w745:dbl[][])
        n179 = control-ref of="XY positions"() -> (w749:refnum<vi>)
        n180 = call "MAIN_save_XY_positions.vi"("queue ASI stage"=w744, 6:"XY positions"=w749, 7:"XY positions"=w745, "error in"=w752, "Start acquisition"=w748, 10:"ROI manager"=w747, 11:"ROI manager"=w746) -> ("error out"=w751:errorcluster, "Next task"=w742:T11, "XY positions OUT"=w743:dbl[][], "XY graph"=w750:cluster{dbl[], dbl[]}[])  [unwired: 1 in]
        n181 = Bundle By Name(cluster=w755, "XY positions"=w743, "merFISH init.ROI defined"=TRUE) -> (w753:T16)
      }
      frame "Main_define_mosaic" {
        n182 = control-ref of="XY positions"() -> (w772:refnum<vi>)
        n183 = Unbundle By Name(w766) -> ("XY positions"=w768:dbl[][])
        n184 = call "Main_define_mosaic.vi"(0:"ROI manager"=w769, "XY positions IN"=w768, "queue ASI stage"=w767, 5:"ROI manager"=w770, "Start acquisition"=w771, "XY positions"=w772, "error in"=w777, "Mosaic size X"="Mosaic size X", "Mosaic size Y"="Mosaic size Y", "FOV size (um)"="FOV size (um)") -> ("XY positions OUT"=w764:dbl[][], "Next task"=w763:T11, "XY graph"=w762:cluster{dbl[], dbl[]}[], "error out"=w776:errorcluster)  [unwired: 2 in]
        n185 = Bundle By Name(cluster=w766, "XY positions"=w764, "merFISH init.ROI defined"=TRUE) -> (w765:T16)
      }
      frame "Main_move_to_XY" {
        n186 = Unbundle By Name(w794) -> ("XY positions"=w785:dbl[][])
        n187 = call "MAIN_move_to_XY_positions.vi"("queue ASI stage"=w786, "error out"=w791, 9:"ROI manager"=w783, 10:"ROI manager"=w784, "XY positions"=w785) -> ("error out"=w790:errorcluster, "Next task"=w789:T11, "ROI manager out"=w788:i32, "XY positions"=w787:dbl[][])  [unwired: 3 in]
        n188 = Bundle By Name(cluster=w794, "XY positions"=w787) -> (w792:T16)
        n189 = local write "ROI manager"(w788) -> ()
      }
      frame "Main_load_XY" {
        n190 = Unbundle By Name(w812) -> ("XY positions"=w801:dbl[][])
        n191 = control-ref of="XY positions"() -> (w804:refnum<vi>)
        n192 = call "MAIN_load_XY_positions.vi"(7:"XY positions"=w801, "error in"=w809, 9:"XY positions"=w804, 10:"ROI manager"=w803, 11:"ROI manager"=w802) -> ("error out"=w808:errorcluster, "Next task"=w806:T11, "XY graph"=w800:cluster{dbl[], dbl[]}[], "XY positions OUT"=w805:dbl[][])  [unwired: 3 in]
        n193 = flat-sequence {
          tunnel: w808 -> [w818]
          tunnel: [w818] -> w807
          frame #0 {
            n194 = local write "ROI manager"(-1 ("ROI manager")) -> ()
          }
        }
        n195 = Bundle By Name(cluster=w812, "XY positions"=w805, "merFISH init.ROI defined"=TRUE) -> (w810:T16)
      }
      frame "Main_discard_XY" {
        n196 = call "ROI_positions_SAVE.vi"("Choice"="Delete all", "XY positions"=dbl[][] [], "error in"=w822, "ROI LstBox Refnum"=w824) -> ("error out"=w828:errorcluster, "XY positions OUT"=w820:dbl[][])  [unwired: 2 in]
        n197 = flat-sequence {
          tunnel: w828 -> [w838]
          tunnel: [w838] -> w829
          frame #0 {
            n198 = local write "ROI manager"(-1 ("ROI manager")) -> ()
          }
        }
        n199 = Bundle By Name(cluster=w826, "REF positions"=w820, "XY positions"=w820, "merFISH init.ROI defined"=FALSE) -> (w821:T16)
        n200 = case shown="False" w830 {
          tunnel: [T11 {"variant"=variant, "Instruction"=enum."Main_not_acquiring"} ("Q_main_element") T11 {"variant"=variant, "Instruction"=enum."Main_acquiring"} ("Q_main_element")] -> w831
          frame False {
          }
          frame True {
          }
        }
      }
      frame "Main_autofocus_calibration" {
        n201 = call <vilib>:"Set Busy.vi"("error in (no error)"=w858) -> ("error out"=w856:errorcluster)  [unwired: 9 in, 1 out]
        n202 = control-ref of="Calibration"() -> (w849:refnum<vi>)
        n203 = control-ref of="Illumination controls"() -> (w842:refnum<vi>)
        n204 = call "MAIN_autofocus_calibration.vi"("Illumination Refnum"=w842, "Start acquisition"=w848, "queue piezo"=w850, "queue FPGA"=w845, "Calibration Refnum"=w849, "Measure QPD"=w843, "error in"=w856, "Ref channel"="Ref channel") -> ("Slope"=w852:dbl, "Next task"=w846:T11, "Sensitivity (nm)"=→"Sensitivity (nm)":dbl, "Calibration"=→"Calibration":cluster{"Y":dbl[], "Y":dbl[]}[], "error out"=w851:errorcluster)  [unwired: 3 in]
        n205 = Unbundle By Name(w851) -> ("status"=w860:bool)
        n206 = call <vilib>:"Unset Busy.vi"("error in (no error)"=w851) -> ("error out"=w857:errorcluster)  [unwired: 10 in]
        n207 = Not(x=w860) -> (.not. x?=w861:bool)
        n208 = flat-sequence {
          tunnel: w857 -> [w869]
          tunnel: [w869] -> w862
          frame #0 {
            n209 = local write "Calib autofocus"(FALSE ("Calibration autofocus")) -> ()
          }
        }
        n210 = Bundle By Name(cluster=w863, "Slope"=w852, "merFISH init.Autofocus calibrated"=w861) -> (w859:T16)
      }
      frame "Main_autofocus_initialization" {
        n211 = call "MAIN_init_autofocus.vi"("Start acquisition"=w874, "queue piezo"=w873, "queue FPGA"=w872, "Measure QPD"=w875, "PID gains"="PID gains", "error in"=w880, "Switch"="Switch", "Init"="Init", "Autotune?"="Autotune?") -> ("Next task"=w870:T11, "error out"=w871:errorcluster)  [unwired: 5 in]
      }
      frame "Main_autofocus_stop" {
        n212 = call "MAIN_stop_autofocus.vi"("Start acquisition"=w891, "queue piezo"=w890, "queue FPGA"=w889, "Measure QPD"=w892, "error in"=w894) -> ("Next task"=w888:T11, "error out"=w893:errorcluster)  [unwired: 9 in]
      }
      frame "Main_save_PID" {
        n213 = Variant To Data(error in=w908, type=T2 {"proportional gain (Kc)"=0.0, "integral time (Ti, min)"=0.0, "derivative time (Td, min)"=0.0} ("PID gains"), Variant=w909) -> (data=w906:T2, error out=w905:errorcluster)
        n214 = local write "PID gains"(w906) -> ()
        n215 = case shown="False" w904 {
          tunnel: [T11 {"variant"=variant, "Instruction"=enum."Main_not_acquiring"} ("Q_main_element") T11 {"variant"=variant, "Instruction"=enum."Main_acquiring"} ("Q_main_element")] -> w903
          frame False {
          }
          frame True {
          }
        }
      }
      frame "Main_change_H_valve_position" {
        n216 = call "MAIN_change_valve_position.vi"("error in"=w927, "variant"=w926, "Start acquisition"=w925, "queue valve"=w924) -> ("error out"=w923:errorcluster, "Valve ready?"=w921:bool, "Next task"=w919:T11, "Valve H"=w920:u8, "Valve position OUT"=→"Valve position OUT":u8)  [unwired: 3 in]
        n217 = case shown="False" w921 {
          tunnel: w923 -> [w936 w937]
          tunnel: [w936 w937] -> w922
          tunnel: w920 -> [w935 _]
          frame False {
            n218 = local write "Valve H"(w935) -> ()
          }
          frame True {
          }
        }
      }
      frame "Main_two_way_valve" {
        n219 = call "MAIN_change_2_way_valve_position.vi"("error in"=w943, "Two-way valve"="Two-way valve", "Start acquisition"=w941, "queue valve"=w938) -> ("error out"=w940:errorcluster, "Next task"=w939:T11)  [unwired: 2 in]
      }
      frame "Main_save_movie" {
        n220 = Bundle(cluster=T19 {"Saving path"=path "", "Sample name"="", "N frames"=0, "N movies"=0, "Start acquisition"=FALSE, "Global parameters"={"405"=0.0, "488"=0.0, "561"=0.0, "641"=0.0, "BF"=0.0, "X"=0.0, "Y"=0.0, "Filter list"=0, "Exp time"=0.0, "Kinetic time"=0.0, "Gain"=0, "Step length (nm)"=0, "Total range (nm)"=0, "Scan illumination\n mode"=FALSE, "Dt (s)"=0, "# repetitions"=0}} ("output cluster"), "Saving path"=w963, "Sample name"=w962, "N frames"=w961, "N movies"=w960, "Start acquisition"=w969, "Global parameters"=w964) -> (w955:T19)
        n221 = call "MAIN_launch_movie_acquisition.vi"("error in"=w957, "Data cluster"=w955, "queue CAMERA"=w954) -> ("error out"=w956:errorcluster, "Next task"=w953:T11)  [unwired: 1 in]
        n222 = while {
          tunnel: w956 -> [w997]
          tunnel: w978 -> [w999]
          tunnel: w977 -> [w1004]
          tunnel: [w1004] -> w976
          tunnel: w975 -> [w983]
          tunnel: w974 -> [w1002]
          tunnel: w973 -> [w984]
          tunnel: [w1000] -> w971
          tunnel: [w999] -> w972
          tunnel: w961 -> [w998]
          tunnel: w967 -> [w994]
          tunnel: [w994] -> w958
          stop <- w989 stop-if-true
          n223 = call "MOVIE_calculate_acquisition_Progress.vi"("error in"=w997, "N frames"=w998) -> ("error out"=w988:errorcluster, "Slider save movie"=→"Slider save movie":u8, "kinetic time (s)"=w993:sgl, "N frames acquired"=→"Frames":i32)  [unwired: 2 in]
          n224 = local write "Kin time (s)"(w993) -> ()
          n225 = property on="Image" class="ImageControl"(error in=w988) -> (error out=w982:errorcluster, "ROI"=w981:T33)  [unwired: 1 in, 1 out]
          n226 = Multiply(x=sgl 1000.0, y=w1004) -> (x*y=w1005:sgl)
          n227 = To Unsigned Long Integer(number=w1005) -> (unsigned 32bit integer=w1003:u32)
          n228 = global read "Global_CAMERA.vi" "CAMERA done"() -> (w991:bool)
          n229 = call "sCMOS_read_extract_images.vi"("ROI"=w981, "error in"=w982, "Image contrast"=w983, "ROI IN"=w984, "Contrast IN"=w1002, "Image"=w999) -> ("error out"=w1000:errorcluster, "ROI OUT"=w986:T5, "Contrast OUT"=w985:T5, "Intensity range"=w1001:T34)  [unwired: 2 in]
          n230 = Wait (ms)(milliseconds to wait=w1003) -> ()  [unwired: 1 out]
          n231 = Unbundle By Name(w988) -> ("status"=w987:bool)
          n232 = Build Array(w991, "Abort movie", w987) -> (w990:bool[])
          n233 = local write "Image"(w985) -> ()
          n234 = local write "ROI"(w986) -> ()
          n235 = local write "Intensity range"(w1001) -> ()
          n236 = Or Array Elements(Boolean array=w990) -> (logical OR=w989:bool)
        }
        n237 = invoke on="Slider save movie" class="Slide (strict)" method="Reinit To Default"(error in=w971) -> (error out=w952:errorcluster)  [unwired: 2 in, 2 out]
        n238 = call "CAMERA_wait_for_task_DONE.vi"("error in"=w952) -> ("error out"=w951:errorcluster)
        n239 = flat-sequence {
          tunnel: w951 -> [w980]
          tunnel: [w980] -> w970
          frame #0 {
            w979 = FALSE ("Start ANDOR")
            n240 = local write "Abort movie"(w979) -> ()
            n241 = local write "Save movie"(w979) -> ()
            n242 = global write "Global_ABORT.vi" "ABORT"(w979) -> ()
          }
        }
      }
      frame "Main_init_single_scan" {
        n243 = Unbundle By Name(w1017) -> ("Laser lines array"=w1012:dbl[][])
        n244 = call "RAMP_save_path_definition_sCMOS_movie.vi"("error in"=w1022, "Sample name"=w1023, "Path to the saving folder"=w1024) -> ("error out"=w1021:errorcluster, "Movie path"=w1020:path)  [unwired: 4 in]
        n245 = Bundle By Name(cluster=w1027, "Step length (nm)"=w1028, "Total range (nm)"=w1029) -> (w1026:T9)
        n246 = invoke on="Autofocus" class="Bool (strict)" method="Reinit To Default"(error in=w1021) -> (error out=w1025:errorcluster)  [unwired: 2 in, 2 out]
        n247 = Array Size(array=w1012) -> (size(s)=w1015:i32[])
        n248 = invoke on="Illumination controls" class="Clust (strict)" method="Reinit To Default"(error in=w1025) -> (error out=w1031:errorcluster)  [unwired: 2 in, 2 out]
        n249 = Index Array(array=w1015, index=0) -> (element=w1016:i32)
        n250 = Not Equal To 0?(x=w1016) -> (x != 0?=w1014:bool)
        n251 = Or(x=w1014, y=w1010) -> (x .or. y?=w1011:bool)
        n252 = case shown="True" w1011 {
          tunnel: w1037 -> [_ w1069]
          tunnel: w1036 -> [_ w1068]
          tunnel: [w1043 w1065] -> w1035
          tunnel: [T11 {"variant"=variant, "Instruction"=enum."Main_idle"} ("Q_main_element") w1064] -> w1034
          tunnel: w1033 -> [_ w1061]
          tunnel: w1032 -> [_ w1060]
          tunnel: w1031 -> [w1045 w1059]
          tunnel: w1030 -> [_ w1058]
          tunnel: w1029 -> [_ w1057]
          tunnel: w1028 -> [_ w1056]
          tunnel: w1020 -> [_ w1054]
          tunnel: w1019 -> [_ w1053]
          tunnel: w1010 -> [_ w1052]
          tunnel: w1012 -> [_ w1051]
          tunnel: w1018 -> [_ w1050]
          tunnel: w1009 -> [_ w1049]
          tunnel: w1008 -> [_ w1048]
          tunnel: w1007 -> [_ w1047]
          frame False {
            n253 = invoke on="Start scan" class="Bool (strict)" method="Reinit To Default"(error in=w1045) -> (error out=w1044:errorcluster)  [unwired: 2 in, 2 out]
            n254 = call "Display Message to User12"("error in (no error)"=w1044) -> ("error out"=w1043:errorcluster)  [unwired: 9 in, 1 out]
          }
          frame True {
            n255 = local read "Autofocus"() -> (w1055:bool)
            n256 = call "RAMP_init_ramp_scan_FPGA.vi"("queue CAMERA"=w1060, "queue piezo"=w1069, "queue DAQ"=w1058, "queue ASI stage"=w1068, "Laser lines array"=w1051, "error in"=w1059, "Illumination source"=w1052, "Brightfield intensity"=w1053, "Display?"=w1047, "Autofocus"=w1055, "Movie path"=w1054, "Total range (nm)"=w1057, "z step (nm)"=w1056, "Start acquisition"=w1061, "Exp time (s)"=w1050, "queue FPGA"=w1049, "Measure QPD"=w1048) -> ("Ramp"=w1063:dbl[], "Total # z steps"=w1062:i32, "Ready"=w1067:bool, "error out"=w1066:errorcluster)  [unwired: 7 in]
            n257 = case shown="True" w1067 {
              tunnel: w1066 -> [w1076 w1085]
              tunnel: [w1071 w1085] -> w1065
              tunnel: [T11 {"variant"=variant, "Instruction"=enum."Main_idle"} ("Q_main_element") w1082] -> w1064
              tunnel: w1063 -> [_ w1080]
              tunnel: w1062 -> [_ w1081]
              tunnel: w1060 -> [w1073 _]
              frame False {
                n258 = call "Display Message to User"("error in (no error)"=w1076) -> ("error out"=w1074:errorcluster)  [unwired: 9 in, 1 out]
                n259 = flat-sequence {
                  tunnel: w1074 -> [w1077]
                  tunnel: [w1077] -> w1072
                  frame #0 {
                    n260 = local write "Start scan"(FALSE ("Start scan")) -> ()
                  }
                }
                n261 = Enqueue Element At Opposite End(queue=w1073, element=T10 {"variant"=variant, "Instruction"=enum."CAMERA_close_scan"} ("Q_ANDOR_element"), error in (no error)=w1072) -> (error out=w1071:errorcluster)  [unwired: 1 in, 2 out]
              }
              frame True {
                n262 = Bundle("Ramp"=w1080, "Total # z steps"=w1081) -> (w1079:cluster{"Ramp":dbl[], "Total # z steps":i32})  [unwired: 1 in]
                n263 = To Variant(anything=w1079) -> (Variant=w1083:variant)
                n264 = Bundle By Name(cluster=T11 {"variant"=variant, "Instruction"=enum."Main_single_scan"} ("Q_main_element"), "variant"=w1083) -> (w1082:T11)
              }
            }
          }
        }
      }
      frame "Main_single_scan" {
        n265 = Variant To Data(error in=w1105, type=cluster{"Ramp":dbl[], "Total # steps":i32} {"Ramp"=[], "Total # steps"=0} ("output cluster"), Variant=w1108) -> (data=w1095:cluster{"Ramp":dbl[], "Total # steps":i32}, error out=w1090:errorcluster)
        n266 = Unbundle By Name(w1095) -> ("Ramp"=w1091:dbl[])
        n267 = call "RAMP_single_scan_FPGA.vi"("error in"=w1090, "Ramp"=w1091, "queue piezo"=w1088, "queue DAQ"=w1087) -> ("error out"=w1089:errorcluster)  [unwired: 3 in]
        n268 = case shown="True" w1086 {
          tunnel: w1107 -> [_ w1116]
          tunnel: w1106 -> [_ w1115]
          tunnel: w1105 -> [w1109 w1114]
          tunnel: w1104 -> [_ w1113]
          tunnel: [w1109 w1112] -> w1098
          tunnel: w1095 -> [_ w1111]
          frame False {
          }
          frame True {
            n269 = Unbundle By Name(w1111) -> ("Total # steps"=w1110:i32)
            n270 = while {
              tunnel: w1116 -> [w1132]
              tunnel: w1115 -> [w1131]
              tunnel: w1113 -> [w1130]
              tunnel: w1114 -> [w1129]
              tunnel: [w1119] -> w1112
              tunnel: w1110 -> [w1120]
              stop <- w1124 stop-if-true
              n271 = local read "Image contrast"() -> (w1127:cluster{i32, i32})
              n272 = call "IMAQ GetImageSize"("Image"=w1130, "error in (no error)"=w1129) -> ("Y Resolution"=w1137:i32, "X Resolution"=w1138:i32, "error out"=w1133:errorcluster)  [unwired: 2 in]
              n273 = Equal To 0?(x=w1138) -> (x = 0?=w1136:bool)
              n274 = Equal To 0?(x=w1137) -> (x = 0?=w1135:bool)
              n275 = Or(x=w1136, y=w1135) -> (x .or. y?=w1134:bool)
              n276 = case shown="False" w1134 {
                tunnel: w1131 -> [w1140 _]
                tunnel: w1132 -> [w1139 _]
                tunnel: [w1149 w1150] -> w1121
                tunnel: w1130 -> [w1141 _]
                tunnel: w1133 -> [w1145 w1150]
                tunnel: w1127 -> [w1142 _]
                frame False {
                  n277 = property on="Image" class="ImageControl"(error in=w1145) -> (error out=w1144:errorcluster, "ROI"=w1143:T33)  [unwired: 1 in, 1 out]
                  n278 = call "sCMOS_read_extract_images.vi"("ROI"=w1143, "error in"=w1144, "Image contrast"=w1142, "ROI IN"=w1139, "Contrast IN"=w1140, "Image"=w1141) -> ("error out"=w1149:errorcluster, "ROI OUT"=w1148:T5, "Contrast OUT"=w1147:T5, "Intensity range"=w1146:T34)  [unwired: 2 in]
                  n279 = local write "Intensity range"(w1146) -> ()
                  n280 = local write "Image"(w1147) -> ()
                  n281 = local write "ROI"(w1148) -> ()
                }
                frame True {
                }
              }
              n282 = call "RAMP_uptade_scan_steps_indicators.vi"("Total # steps"=w1120, "error in"=w1121) -> ("slider"=→"Scan slider":u8, "scan step"=→"Number steps":i32, "error out"=w1119:errorcluster)  [unwired: 4 in]
              n283 = global read "Global_MAIN.vi" "Stop scan"() -> (w1125:bool)
              n284 = Unbundle By Name(w1121) -> ("status"=w1122:bool)
              n285 = Wait (ms)(milliseconds to wait=u32 50) -> ()  [unwired: 1 out]
              n286 = Build Array(w1125, "Abort scan", w1122) -> (w1123:bool[])
              n287 = Or Array Elements(Boolean array=w1123) -> (logical OR=w1124:bool)
            }
          }
        }
        n288 = Merge Errors(w1098, w1089) -> (w1093:errorcluster)
        n289 = invoke on="Start scan" class="Bool (strict)" method="Reinit To Default"(error in=w1093) -> (error out=w1092:errorcluster)  [unwired: 2 in, 2 out]
      }
      frame "Main_stop_single_scan" {
        n290 = flat-sequence {
          tunnel: w1165 -> [w1173]
          tunnel: [w1173] -> w1153
          frame #0 {
            w1172 = FALSE ("Abort scan")
            n291 = local write "Abort scan"(w1172) -> ()
            n292 = local write "Start scan"(w1172) -> ()
            n293 = local write "Scan slider"(u8 0 ("Scan slider")) -> ()
            n294 = local write "Number steps"(0 ("Number steps")) -> ()
          }
        }
        n295 = call "MAIN_close_scan_FPGA.vi"("Sample name"=w1161, "Saving path"=w1160, "queue piezo"=w1159, "queue ASI stage"=w1158, "queue CAMERA"=w1157, "Laser list Refnum"=w1162, "queue FPGA"=w1156, "Illumination source"=w1163, "Start acquisition"=w1164, "Measure QPD"=w1154, "error in"=w1153, "Global parameters"=w1152) -> ("Next task"=w1155:T11, "error out"=w1151:errorcluster)  [unwired: 2 in]
      }
      frame "Main_merFISH_illumination_parameters" {
        n296 = Bundle By Name(cluster=w1178, "Scan illumination\n mode"=w1179) -> (w1177:T9)
        n297 = Unbundle By Name(w1181) -> ("Laser lines array"=w1180:dbl[][])
        n298 = case shown="False" w1179 {
          tunnel: w1191 -> [w1204 w1226]
          tunnel: [w1195 w1225] -> w1182
          tunnel: w1184 -> [w1199 _]
          tunnel: w1181 -> [w1197 w1234]
          tunnel: [w1196 w1234] -> w1176
          tunnel: w1180 -> [w1194 _]
          frame False {
            w1205 = T17."Enabled" ("Disabled")
            n299 = property on="Select laser lines" class="Bool (strict)"(error in=w1204, "Visible"=TRUE) -> (error out=w1203:errorcluster)  [unwired: 1 in, 1 out]
            n300 = property on="Brightfield intensity" class="DigNum (strict)"(error in=w1204, "Visible"=FALSE) -> (error out=w1200:errorcluster)  [unwired: 1 in, 1 out]
            n301 = property on="Select laser lines" class="Bool (strict)"(error in=w1204, "DisabledEnum"=w1205) -> (error out=w1201:errorcluster)  [unwired: 1 in, 1 out]
            n302 = property on="Laser lines manager" class="LstBox (strict)"(error in=w1204, "DisabledEnum"=w1205) -> (error out=w1202:errorcluster)  [unwired: 1 in, 1 out]
            n303 = Merge Errors(w1203, w1200, w1201, w1202) -> (w1198:errorcluster)
            n304 = case shown="True" w1199 {
              tunnel: w1198 -> [w1209 w1224]
              tunnel: w1197 -> [w1208 w1220]
              tunnel: [w1208 w1221] -> w1196
              tunnel: [w1209 w1213] -> w1195
              tunnel: w1194 -> [_ w1215]
              frame False {
              }
              frame True {
                n305 = call "RAMP_scan_select-laser-lines.vi"("error in"=w1224, "Laser lines array  IN"=w1215) -> ("Item Names"=w1222:string[], "error out"=w1223:errorcluster, "Laser lines array"=w1211:dbl[][])  [unwired: 1 in]
                n306 = Array Size(array=w1211) -> (size(s)=w1219:i32[])
                n307 = property on="Laser lines manager" class="LstBox (strict)"(error in=w1223, "Item Names"=w1222) -> (error out=w1214:errorcluster)  [unwired: 1 in, 1 out]
                n308 = Index Array(array=w1219, index=0) -> (element=w1217:i32)
                n309 = Greater Than 0?(x=w1217) -> (x > 0?=w1216:bool)
                n310 = To Variant(anything=w1211) -> (Variant=w1212:variant)
                n311 = Bundle By Name(cluster=w1220, "Laser lines array"=w1211, "merFISH init.Laser defined"=w1216) -> (w1221:T16)
                n312 = call "MAIN_save_parameters_TDMS.vi"("error in"=w1214, "Data"=w1212, "Channel name"="Laser illumination" ("group name")) -> ("error out"=w1213:errorcluster)  [unwired: 2 in]
              }
            }
          }
          frame True {
            w1231 = T17."Disabled and Grayed Out" ("Disabled")
            n313 = property on="Select laser lines" class="Bool (strict)"(error in=w1226, "Visible"=FALSE) -> (error out=w1230:errorcluster)  [unwired: 1 in, 1 out]
            n314 = property on="Brightfield intensity" class="DigNum (strict)"(error in=w1226, "Visible"=TRUE) -> (error out=w1227:errorcluster)  [unwired: 1 in, 1 out]
            n315 = property on="Select laser lines" class="Bool (strict)"(error in=w1226, "DisabledEnum"=w1231) -> (error out=w1228:errorcluster)  [unwired: 1 in, 1 out]
            n316 = property on="Laser lines manager" class="LstBox (strict)"(error in=w1226, "DisabledEnum"=w1231) -> (error out=w1229:errorcluster)  [unwired: 1 in, 1 out]
            n317 = Merge Errors(w1230, w1227, w1228, w1229) -> (w1225:errorcluster)
          }
        }
        n318 = case shown="False" w1186 {
          tunnel: [T11 {"variant"=variant, "Instruction"=enum."Main_not_acquiring"} ("Q_main_element") T11 {"variant"=variant, "Instruction"=enum."Main_acquiring"} ("Q_main_element")] -> w1185
          frame False {
          }
          frame True {
          }
        }
      }
      frame "Main_merFISH_buffer_probe_list" {
        n319 = call "merFISH_define_buffer_probe_lists.vi"("error in"=w1241, "Start acquisition"=w1236, "Probe Refnum"=w1240, "Buffer Refnum"=w1239) -> ("error out"=w1237:errorcluster, "Next task"=w1235:T11)  [unwired: 2 in]
      }
      frame "Main_merFISH_injections_procedure" {
        n320 = Unbundle By Name(w1264) -> ("Hybridization procedure"=w1256:i32[][], "Photobleaching procedure"=w1255:i32[][])
        n321 = call "merFISH_define_injections_procedure.vi"("Injection procedure IN photobleaching"=w1255, "Injection procedure IN hybridization"=w1256, "Buffer Refnum"=w1254, "Start acquisition"=w1253, "error in"=w1271, "Defaut injection"="Defaut injection", "Defaut injection photobleaching"="Defaut injection photobleaching") -> ("Injection procedure OUT"=w1252:i32[][], "Injection procedure OUT\nPhotobleaching"=w1251:i32[][], "Next task"=w1250:T11, "error out"=w1257:errorcluster, "Item Names photobleaching"=w1260:string[], "Item Names"=w1263:string[])  [unwired: 3 in]
        n322 = Bundle By Name(cluster=w1264, "Hybridization procedure"=w1252, "Photobleaching procedure"=w1251, "merFISH init.Injection procedure defined"=TRUE) -> (w1258:T16)
        n323 = property on="Hybridization manager" class="LstBox (strict)"(error in=w1257, "Item Names"=w1263) -> (error out=w1261:errorcluster)  [unwired: 1 in, 1 out]
        n324 = property on="Photobleaching manager" class="LstBox (strict)"(error in=w1261, "Item Names"=w1260) -> (error out=w1259:errorcluster)  [unwired: 1 in, 1 out]
      }
      frame "Main_merFISH_save_setpoint" {
        n325 = case shown="True" w1272 {
          tunnel: w1278 -> [w1289 w1301]
          tunnel: [w1289 w1298] -> w1277
          tunnel: w1276 -> [w1288 w1297]
          tunnel: [w1287 w1296] -> w1275
          tunnel: w1274 -> [w1286 w1295]
          tunnel: [w1285 w1294] -> w1273
          frame False {
            n326 = case shown="False" w1286 {
              tunnel: [T11 {"variant"=variant, "Instruction"=enum."Main_not_acquiring"} ("Q_main_element") T11 {"variant"=variant, "Instruction"=enum."Main_acquiring"} ("Q_main_element")] -> w1285
              frame False {
              }
              frame True {
              }
            }
            n327 = call "Display Message to User13"("error in (no error)"=w1288) -> ("error out"=w1287:errorcluster)  [unwired: 9 in, 1 out]
          }
          frame True {
            n328 = call "MAIN_save_merFISH_setpoint.vi"("error in"=w1297, "Start acquisition"=w1295) -> ("error out"=w1296:errorcluster, "Next task"=w1294:T11, "QPD"=w1293:T32)  [unwired: 1 in]
            n329 = Bundle By Name(cluster=w1301, "merFISH init.Autofocus setpoint defined"=TRUE, "QPD ref"=w1293) -> (w1298:T16)
            n330 = Unbundle By Name(w1293) -> ("X"=w1299:sgl)
            n331 = To Double Precision Float(number=w1299) -> (double precision float=→"merFISH setpoint":dbl)
          }
        }
      }
      frame "Main_merFISH_DAPI_parameters" {
        w1305 = TRUE ("merFISH init.Laser defined")
        w1306 = i32[][] [] ("Hybridization procedure")
        w1309 = dbl[][] [[15.0, 1.0, 1.0], [2.0, 2.0, 1.0]] ("Laser lines array  IN")
        n332 = control-ref of="Hybridization manager"() -> (w1313:refnum<vi>)
        n333 = control-ref of="Photobleaching manager"() -> (w1314:refnum<vi>)
        n334 = call "merFISH_define_DAPI_parameters.vi"("Probe Refnum"=w1311, "Probe Names"=string[][] [["DAPI", "0"]] ("Item Names"), "Laser Refnum"=w1312, "error in"=w1315, "Photobleaching Refnum"=w1314, "Hybridization Refnum"=w1313, "Laser lines array  IN"=w1309) -> ("error out"=w1302:errorcluster)  [unwired: 4 in]
        n335 = flat-sequence {
          tunnel: w1302 -> [w1322]
          tunnel: [w1322] -> w1303
          frame #0 {
            n336 = local write "Illumination source"(FALSE ("Illumination source")) -> ()
          }
        }
        n337 = Bundle By Name(cluster=w1310, "Laser lines array"=w1309, "merFISH init.Injection procedure defined"=w1305, "merFISH init.Laser defined"=w1305, "Photobleaching procedure"=w1306, "Hybridization procedure"=w1306) -> (w1308:T16)
      }
      frame "Main_merFISH_Brightfield_parameters" {
        w1326 = dbl[][] [] ("Laser lines array")
        w1327 = TRUE ("merFISH init.Laser defined")
        w1328 = i32[][] [] ("Hybridization procedure")
        n338 = control-ref of="Hybridization manager"() -> (w1334:refnum<vi>)
        n339 = control-ref of="Photobleaching manager"() -> (w1335:refnum<vi>)
        n340 = call "merFISH_define_DAPI_parameters.vi"("Probe Refnum"=w1332, "Probe Names"=string[][] [["BF", "0"]] ("Item Names"), "Laser Refnum"=w1333, "error in"=w1336, "Photobleaching Refnum"=w1335, "Hybridization Refnum"=w1334, "Laser lines array  IN"=w1326) -> ("error out"=w1324:errorcluster)  [unwired: 4 in]
        n341 = flat-sequence {
          tunnel: [w1344] -> w1325
          tunnel: w1324 -> [w1344]
          frame #0 {
            n342 = local write "Illumination source"(TRUE ("Illumination source")) -> ()
            n343 = local write "Brightfield intensity"(7.0 ("Brightfield intensity")) -> ()
          }
        }
        n344 = Bundle By Name(cluster=w1331, "Laser lines array"=w1326, "merFISH init.Injection procedure defined"=w1327, "merFISH init.Laser defined"=w1327, "Photobleaching procedure"=w1328, "Hybridization procedure"=w1328) -> (w1330:T16)
      }
      frame "Main_merFISH_save_embryo_ROI" {
        n345 = Unbundle By Name(w1349) -> ("XY positions"=w1354:dbl[][], "REF positions"=w1355:dbl[][])
        n346 = call <vilib>:"Set Busy.vi"("error in (no error)"=w1370) -> ("error out"=w1367:errorcluster)  [unwired: 9 in, 1 out]
        n347 = Bundle By Name(cluster=T20 {"XY positions"=[], "REF positions"=[]} ("output cluster"), "XY positions"=w1354, "REF positions"=w1355) -> (w1352:T20)
        n348 = control-ref of="XY positions"() -> (w1363:refnum<vi>)
        n349 = call "MAIN_save_embryos_positions.vi"("Contrast image"=w1360, "Image contrast"=w1359, "XY REF cluster"=w1352, "New Image"=w1358, "queue ASI stage"=w1357, 5:"ROI manager"=w1361, 7:"ROI manager"=w1362, "Start acquisition"=w1365, "error in"=w1367, "XY positions"=w1363, "XY graph"=w1364) -> ("XY REF cluster OUT"=w1350:T20, "Next task"=w1356:T11, "XY graph OUT"=w1368:cluster{dbl[], dbl[]}[], "error out"=w1366:errorcluster)  [unwired: 1 in]
        n350 = Unbundle By Name(w1350) -> ("XY positions"=w1347:dbl[][], "REF positions"=w1351:dbl[][])
        n351 = Bundle By Name(cluster=w1349, "XY positions"=w1347, "REF positions"=w1351) -> (w1348:T16)
        n352 = call <vilib>:"Unset Busy.vi"("error in (no error)"=w1366) -> ("error out"=w1369:errorcluster)  [unwired: 10 in]
      }
      frame "Main_merFISH_init" {
        n353 = Unbundle By Name(w1394) -> ("Hybridization procedure"=w1393:i32[][], "XY positions"=w1418:dbl[][], "Laser lines array"=w1391:dbl[][], "merFISH init"=w1392:T6)
        n354 = call "merFISH_path_definition.vi"("error in"=w1384, "Sample name"=w1404, "Saving path"=w1405) -> ("error out"=w1382:errorcluster, "merFISH path"=w1385:path)  [unwired: 1 out]
        n355 = Bundle("queue FPGA"=w1376, "queue pump"=w1402, "queue valve"=w1401, "queue DAQ"=w1400, "queue CAMERA"=w1397, "queue ASI stage"=w1399, "queue piezo"=w1398) -> (w1396:T35)  [unwired: 1 in]
        n356 = Bundle By Name(cluster=w1409, "Step length (nm)"=w1406, "Total range (nm)"=w1407) -> (w1408:T9)
        n357 = To Variant(anything=w1385) -> (Variant=w1386:variant)
        n358 = Unbundle(w1392) -> ("Autofocus calibrated"=w1417:bool, "Autofocus setpoint defined"=w1416:bool, "Laser defined"=w1415:bool, "ROI defined"=w1414:bool, "Injection procedure defined"=w1403:bool)
        n359 = call "MAIN_save_parameters_TDMS.vi"("error in"=w1382, "Data"=w1386, "Channel name"="merFISH path") -> ("error out"=w1381:errorcluster)  [unwired: 2 in]
        n360 = call "merFISH_count_probes.vi"("MCListbox Refnum"=w1379, "error in"=w1381) -> ("error out"=w1380:errorcluster, "At least one probe?"=w1378:bool)  [unwired: 5 in]
        n361 = Build Array(w1417, w1416, w1415, w1414, w1403, w1378) -> (w1413:bool[])
        n362 = And Array Elements(Boolean array=w1413) -> (logical AND=w1412:bool)
        n363 = case shown="True" w1412 {
          tunnel: w1408 -> [w1438 w1476]
          tunnel: [w1438 w1476] -> w1423
          tunnel: w1407 -> [_ w1453]
          tunnel: w1406 -> [_ w1452]
          tunnel: w1422 -> [_ w1465]
          tunnel: [w1431 w1479] -> w1421
          tunnel: [w1435 w1478] -> w1420
          tunnel: w1419 -> [w1436 w1451]
          tunnel: w1397 -> [_ w1475]
          tunnel: w1418 -> [_ w1447]
          tunnel: w1411 -> [w1437 w1477]
          tunnel: [w1437 w1477] -> w1410
          tunnel: w1385 -> [_ w1468]
          tunnel: w1380 -> [w1430 w1459]
          tunnel: w1396 -> [_ w1470]
          tunnel: w1395 -> [_ w1457]
          tunnel: w1394 -> [w1434 w1472]
          tunnel: [w1434 w1471] -> w1388
          tunnel: w1393 -> [_ w1448]
          tunnel: w1391 -> [_ w1466]
          tunnel: w1390 -> [_ w1456]
          tunnel: w1389 -> [_ w1450]
          tunnel: w1383 -> [_ w1460]
          tunnel: w1378 -> [w1429 _]
          tunnel: w1377 -> [_ w1449]
          tunnel: w1375 -> [_ w1445]
          frame False {
            n364 = case shown="True" w1429 {
              tunnel: w1430 -> [w1440 w1441]
              tunnel: [w1439 w1441] -> w1428
              frame False {
                n365 = call "Display Message to User34"("error in (no error)"=w1440) -> ("error out"=w1439:errorcluster)  [unwired: 9 in, 1 out]
              }
              frame True {
              }
            }
            n366 = invoke on="merFISH" class="Bool (strict)" method="Reinit To Default"(error in=w1428) -> (error out=w1432:errorcluster)  [unwired: 2 in, 2 out]
            n367 = invoke on="Illumination controls" class="Clust (strict)" method="Reinit To Default"(error in=w1432) -> (error out=w1433:errorcluster)  [unwired: 2 in, 2 out]
            n368 = invoke on="Autofocus" class="Bool (strict)" method="Reinit To Default"(error in=w1433) -> (error out=w1431:errorcluster)  [unwired: 2 in, 2 out]
            n369 = case shown="False" w1436 {
              tunnel: [T11 {"variant"=variant, "Instruction"=enum."Main_not_acquiring"} ("Q_main_element") T11 {"variant"=variant, "Instruction"=enum."Main_start_acquiring"} ("Q_main_element")] -> w1435
              frame False {
              }
              frame True {
              }
            }
          }
          frame True {
            n370 = invoke on="ROI" class="ImageControl" method="Reinit To Default"(error in=w1459) -> (error out=w1458:errorcluster)  [unwired: 2 in, 2 out]
            n371 = call "merFISH_sort_laser_lines.vi"("Laser lines array"=w1466) -> ("Laser lines merFISH"=w1463:dbl[][], "N laser lines merFISH"=w1464:i32)  [unwired: 2 in, 1 out]
            n372 = control-ref of="Probe list"() -> (w1455:refnum<vi>)
            n373 = local read "Autofocus"() -> (w1454:bool)
            n374 = Bundle By Name(cluster=T21 {"z step (nm)"=0, "Total range (nm)"=0, "N laser lines merFISH"=0, "Start acquisition"=FALSE, "Brightfield intensity"=0.0, "Autofocus"=FALSE, "Probe List Refnum"=refnum, "Injection procedure IN"=[], "Valve H"=0, "Measure QPD"=FALSE, "Laser lines array"=[], "Exp time (s)"=0.0, "Illumination source"=FALSE, "XY positions"=[], "merFISH mode"=0} ("Input data cluster"), "merFISH mode"=w1445, "Injection procedure IN"=w1448, "XY positions"=w1447, "Laser lines array"=w1463, "N laser lines merFISH"=w1464, "Brightfield intensity"=w1465, "Illumination source"=w1449, "Exp time (s)"=w1450, "Start acquisition"=w1451, "z step (nm)"=w1452, "Total range (nm)"=w1453, "Autofocus"=w1454, "Probe List Refnum"=w1455, "Measure QPD"=w1456, "Valve H"=w1457) -> (w1444:T21)
            n375 = call "merFISH_initialization.vi"("queue cluster"=w1470, "Input data cluster"=w1444, "error in"=w1458, "merFISH path"=w1468) -> ("refnum log file"=w1461:refnum<file>, "Ramp"=w1462:dbl[], "Total # z steps"=w1473:i32, "Ready"=w1467:bool, "Total # frames"=w1469:i32, "error out"=w1474:errorcluster)  [unwired: 2 in]
            n376 = case shown="True" w1467 {
              tunnel: w1474 -> [_ w1495]
              tunnel: [w1485 w1501] -> w1479
              tunnel: [T11 {"variant"=variant, "Instruction"=enum."Main_idle"} ("Q_main_element") w1500] -> w1478
              tunnel: w1462 -> [_ w1506]
              tunnel: w1473 -> [_ w1504]
              tunnel: w1475 -> [w1486 _]
              tunnel: w1472 -> [w1484 w1507]
              tunnel: [w1484 w1505] -> w1471
              tunnel: w1461 -> [_ w1497]
              tunnel: w1451 -> [w1480 _]
              tunnel: w1468 -> [_ w1503]
              tunnel: w1469 -> [_ w1502]
              tunnel: w1460 -> [_ w1493]
              frame False {
                n377 = call "Display Message to User3"() -> ("error out"=w1483:errorcluster)  [unwired: 10 in, 1 out]
                n378 = Bundle By Name(cluster=T22 {"Start acquisition"=FALSE, "Frame transfer"=FALSE, "Movie path"=""} ("output cluster"), "Frame transfer"=FALSE, "Start acquisition"=w1480) -> (w1488:T22)
                n379 = invoke on="merFISH" class="Bool (strict)" method="Reinit To Default"(error in=w1483) -> (error out=w1482:errorcluster)  [unwired: 2 in, 2 out]
                n380 = To Variant(anything=w1488) -> (Variant=w1489:variant)
                n381 = Bundle By Name(cluster=T10 {"variant"=variant, "Instruction"=enum."CAMERA_close_scan"} ("Q_ANDOR_element"), "variant"=w1489) -> (w1487:T10)
                n382 = Enqueue Element At Opposite End(queue=w1486, element=w1487, error in (no error)=w1482) -> (error out=w1485:errorcluster)  [unwired: 1 in, 2 out]
              }
              frame True {
                n383 = Flush Queue(queue=w1493, error in (no error)=w1495) -> (error out=w1494:errorcluster)  [unwired: 2 out]
                n384 = invoke on="Illumination controls" class="Clust (strict)" method="Reinit To Default"(error in=w1494) -> (error out=w1499:errorcluster)  [unwired: 2 in, 2 out]
                n385 = invoke on="Autofocus" class="Bool (strict)" method="Reinit To Default"(error in=w1499) -> (error out=w1498:errorcluster)  [unwired: 2 in, 2 out]
                n386 = call <vilib>:"High Resolution Relative Seconds.vi"() -> ("relative seconds"=w1496:dbl)
                n387 = Bundle By Name(cluster=w1507, "Starting time"=w1496, "merFISH path"=w1503, "Total # frames"=w1502, "Total # z steps"=w1504, "Ramp"=w1506, "Log file"=w1497) -> (w1505:T16)
                n388 = call "merFISH_read_next_task_TDMS.vi"("error in"=w1498, "Starting time"=w1496, "Log file"=w1497) -> ("error out"=w1501:errorcluster, "task"=w1500:T11)  [unwired: 1 in]
              }
            }
          }
        }
      }
      frame "Main_merFISH_start_autofocus" {
        n389 = flat-sequence {
          tunnel: w1509 -> [w1525]
          tunnel: [w1525] -> w1517
          frame #0 {
            w1526 = FALSE ("Autofocus lost")
            n390 = global write "Global_MCL_piezo.vi" "Autofocus lost"(w1526) -> ()
            "Autofocus lost" <- w1526
          }
        }
        n391 = Unbundle By Name(w1518) -> ("QPD ref"=w1511:T32, "Log file"=w1515:refnum<file>, "Starting time"=w1516:dbl)
        n392 = local read "PID gains"() -> (w1513:T2)
        n393 = call "MAIN_merFISH_start_autofocus.vi"("queue FPGA"=w1510, "PID gains"=w1513, "queue piezo"=w1514, "error in"=w1517, "Starting time"=w1516, "Log file"=w1515, "QPD ref"=w1511) -> ("error out"=w1508:errorcluster, "Next task"=w1512:T11)  [unwired: 3 in]
      }
      frame "Main_merFISH_open_close_valve_merFISH" {
        n394 = Unbundle By Name(w1540) -> ("Hybridization procedure"=w1544:i32[][], "Log file"=w1532:refnum<file>, "Starting time"=w1533:dbl)
        n395 = Array Size(array=w1544) -> (size(s)=w1543:i32[])
        n396 = Index Array(array=w1543, index=0) -> (element=w1541:i32)
        n397 = control-ref of="Two-way valve"() -> (w1534:refnum<vi>)
        n398 = Not Equal To 0?(x=w1541) -> (x != 0?=w1531:bool)
        n399 = call "MAIN_merFISH_open_close_valve.vi"("Log file"=w1532, "Hybridization procedure not empty?"=w1531, "queue piezo"=w1530, "queue ASI stage"=w1529, "queue valve"=w1527, "Starting time"=w1533, "Measure QPD"=w1535, "variant"=w1536, "error in"=w1539, "Two-way valve"=w1534) -> ("Next task"=w1528:T11, "error out"=w1538:errorcluster)  [unwired: 4 in]
        n400 = flat-sequence {
          tunnel: w1538 -> [w1552]
          tunnel: [w1552] -> w1537
          frame #0 {
            w1551 = -1
            n401 = local write "Photobleaching manager"(w1551) -> ()
            n402 = local write "Hybridization manager"(w1551) -> ()
          }
        }
      }
      frame "Main_merFISH_open_close_valve_photobleaching" {
        n403 = Unbundle By Name(w1565) -> ("Photobleaching procedure"=w1569:i32[][], "Log file"=w1559:refnum<file>, "Starting time"=w1560:dbl)
        n404 = Array Size(array=w1569) -> (size(s)=w1568:i32[])
        n405 = Index Array(array=w1568, index=0) -> (element=w1566:i32)
        n406 = control-ref of="Two-way valve"() -> (w1561:refnum<vi>)
        n407 = Not Equal To 0?(x=w1566) -> (x != 0?=w1558:bool)
        n408 = call "MAIN_merFISH_open_close_valve.vi"("Log file"=w1559, "Hybridization procedure not empty?"=w1558, "queue piezo"=w1557, "queue ASI stage"=w1556, "queue valve"=w1553, "Starting time"=w1560, "Measure QPD"=w1562, "variant"=w1563, "error in"=w1564, "Two-way valve"=w1561) -> ("Next task"=w1555:T11, "error out"=w1554:errorcluster)  [unwired: 4 in]
      }
      frame "Main_merFISH_hybridization" {
        n409 = Unbundle By Name(w1584) -> ("Hybridization procedure"=w1583:i32[][], "Log file"=w1581:refnum<file>, "Starting time"=w1580:dbl)
        n410 = Bundle By Name(cluster=T23 {"Log file"=refnum, "Starting time"=0.0, "Hybridization procedure"=[]} ("output cluster"), "Hybridization procedure"=w1583, "Log file"=w1581, "Starting time"=w1580) -> (w1579:T23)
        n411 = control-ref of="Hybridization manager"() -> (w1590:refnum<vi>)
        n412 = control-ref of="Valve position OUT"() -> (w1588:refnum<vi>)
        n413 = control-ref of="Valve H"() -> (w1589:refnum<vi>)
        n414 = call "MAIN_merFISH_hybridization.vi"("Data cluster"=w1579, "queue valve"=w1578, "queue pump"=w1577, "Probe list"=w1585, "Valve H"=w1586, "variant"=w1587, "error in"=w1592, "Hybridization manager Refnum"=w1590, "Valve Refnum"=w1589, "Valve position OUT Refnum"=w1588) -> ("Next task"=w1576:T11, "error out"=w1591:errorcluster)  [unwired: 4 in]
      }
      frame "Main_merFISH_move_to_ROI" {
        n415 = Unbundle By Name(w1606) -> ("XY positions"=w1620:dbl[][], "QPD ref"=w1619:T32, "Slope"=w1618:dbl, "Starting time"=w1617:dbl, "Log file"=w1616:refnum<file>)
        n416 = Bundle By Name(cluster=T24 {"XY positions"=[], "Slope"=0.0, "Starting time"=0.0, "Log file"=refnum, "QPD ref"={"X"=0.0, "Y"=0.0, "SUM"=0.0, "count"=0}} ("Data cluster"), "XY positions"=w1620, "QPD ref"=w1619, "Slope"=w1618, "Starting time"=w1617, "Log file"=w1616) -> (w1602:T24)
        n417 = control-ref of="XY positions"() -> (w1603:refnum<vi>)
        n418 = call "MAIN_merFISH_move_to_ROI.vi"("Data cluster"=w1602, "queue piezo"=w1610, "queue ASI stage"=w1609, "merFISH mode"=w1601, "ROI manager Refnum"=w1612, "variant"=w1614, "error in"=w1615, "XY positions Refnum"=w1603, "Global parameters IN"=w1613) -> ("XY positions OUT"=w1605:dbl[][], "Next task"=w1607:T11, "XY graph"=w1608:cluster{dbl[], dbl[]}[], "Global parameters out"=w1611:T9, "error out"=w1600:errorcluster)  [unwired: 2 in]
        n419 = Bundle By Name(cluster=w1606, "XY positions"=w1605) -> (w1604:T16)
        n420 = flat-sequence {
          tunnel: w1600 -> [w1627]
          tunnel: [w1627] -> w1599
          frame #0 {
            n421 = global write "Global_MAIN.vi" "Stop scan"(FALSE ("Stop scan")) -> ()
          }
        }
      }
      frame "Main_merFISH_move_to_REF" {
        n422 = Unbundle By Name(w1636) -> ("REF positions"=w1632:dbl[][], "XY positions"=w1649:dbl[][], "QPD ref"=w1630:T32, "Slope"=w1648:dbl, "Starting time"=w1647:dbl, "Log file"=w1646:refnum<file>)
        n423 = Bundle By Name(cluster=T25 {"REF positions"=[], "Slope"=0.0, "Starting time"=0.0, "Log file"=refnum, "XY positions"=[], "QPD ref"={"X"=0.0, "Y"=0.0, "SUM"=0.0, "count"=0}} ("Data cluster"), "REF positions"=w1632, "XY positions"=w1649, "QPD ref"=w1630, "Slope"=w1648, "Starting time"=w1647, "Log file"=w1646) -> (w1629:T25)
        n424 = control-ref of="XY positions"() -> (w1633:refnum<vi>)
        n425 = call "MAIN_merFISH_move_to_REF.vi"("Data cluster"=w1629, "queue piezo"=w1640, "queue ASI stage"=w1639, "ROI manager"=w1628, "variant"=w1643, "error in"=w1645, "XY positions Refnum"=w1633, "Global parameters IN"=w1642) -> ("XY positions OUT"=w1635:dbl[][], "Next task"=w1637:T11, "XY graph"=w1638:cluster{dbl[], dbl[]}[], "Global parameters out"=w1641:T9, "error out"=w1644:errorcluster)  [unwired: 3 in]
        n426 = Bundle By Name(cluster=w1636, "XY positions"=w1635) -> (w1634:T16)
      }
      frame "Main_merFISH_wait_stabilization" {
        n427 = Unbundle By Name(w1660) -> ("QPD ref"=w1662:T32, "Slope"=w1666:dbl, "Log file"=w1663:refnum<file>, "Starting time"=w1665:dbl)
        n428 = Bundle By Name(cluster=T26 {"QPD ref"={"X"=0.0, "Y"=0.0, "SUM"=0.0, "count"=0}, "Slope"=0.0, "Log file"=refnum, "Starting time"=0.0} ("Data cluster"), "QPD ref"=w1662, "Slope"=w1666, "Log file"=w1663, "Starting time"=w1665) -> (w1658:T26)
        n429 = call "MAIN_merFISH_wait_for_stabilization.vi"("queue ASI stage"=w1656, "error in"=w1661, "Measure QPD"=w1664, "Data cluster"=w1658, "queue piezo"=w1657) -> ("error out"=w1654:errorcluster, "Next task"=w1655:T11)  [unwired: 3 in]
      }
      frame "Main_merFISH_scan" {
        n430 = Variant To Data(error in=w1692, type=T28 {"ROI #"=0, "Probe #"=0, "Folder# "=0, "Embryo #"=0}, Variant=w1691) -> (data=w1674:T28, error out=w1690:errorcluster)
        n431 = while {
          tunnel: w1706 -> [w1759]
          tunnel: w1705 -> [w1760]
          tunnel: w1704 -> [w1762]
          tunnel: w1692 -> [w1761]
          tunnel: w1677 -> [w1751]
          tunnel: w1703 -> [w1755]
          tunnel: [w1754] -> w1697
          stop <- w1750 stop-if-true
          n432 = call "merFISH_display_scan_new_image.vi"("Display?"=w1751, "error in"=w1761, "Treated image"=w1759, "Image contrast"=w1760, "Real time image"=w1762) -> ("error out"=w1754:errorcluster, "intensity range"=w1764:T34, "Image Dst Out"=w1763:T5)  [unwired: 1 in]
          n433 = Not(x=w1751) -> (.not. x?=w1749:bool)
          n434 = local write "Image"(w1763) -> ()
          n435 = local write "Intensity range"(w1764) -> ()
          n436 = global read "Global_MAIN.vi" "Stop scan"() -> (w1748:bool)
          n437 = global read "Global_ABORT.vi" "ABORT"() -> (w1752:bool)
          n438 = Subtract(x=w1755, y=sgl 10.0) -> (x-y=w1757:sgl)
          n439 = To Unsigned Long Integer(number=w1757) -> (unsigned 32bit integer=w1756:u32)
          n440 = Wait (ms)(milliseconds to wait=w1756) -> ()  [unwired: 1 out]
          n441 = Build Array(w1748, w1749, w1752) -> (w1753:bool[])
          n442 = Or Array Elements(Boolean array=w1753) -> (logical OR=w1750:bool)
        }
        n443 = Unbundle By Name(w1684) -> ("Ramp"=w1682:dbl[], "Total # frames"=w1679:i32, "merFISH path"=w1678:path)
        n444 = Bundle By Name(cluster=T27 {"Ramp"=[], "merFISH path"=path "", "Total # frames"=0, "Display?"=FALSE, "Probe list"=refnum} ("output cluster"), "Probe list"=w1680, "Ramp"=w1682, "Total # frames"=w1679, "merFISH path"=w1678, "Display?"=w1677) -> (w1673:T27)
        n445 = call "merFISH_initialize_Z_ramp_FPGA.vi"("queue DAQ"=w1699, "queue piezo"=w1675, "queue CAMERA"=w1676, "Variant data"=w1674, "Data cluster"=w1673, "error in"=w1690) -> ("Ramp"=w1702:dbl[], "PATH cluster"=w1685:T36, "error out"=w1700:errorcluster)  [unwired: 7 in]
        n446 = Unbundle By Name(w1684) -> ("Total # z steps"=w1701:i32)
        n447 = for {
          tunnel: w1702 -> [w1728] mode=indexing
          tunnel: w1701 -> [w1723]
          tunnel: w1700 -> [w1727]
          tunnel: w1675 -> [w1725]
          tunnel: w1699 -> [w1726]
          tunnel: w1675 -> [w1719]
          tunnel: w1676 -> [w1718]
          tunnel: [w1717] -> w1698
          tunnel: w1680 -> [w1716]
          tunnel: w1681 -> [w1715]
          tunnel: w1689 -> [w1714]
          tunnel: w1674 -> [w1713]
          tunnel: w1688 -> [w1712]
          tunnel: w1685 -> [w1711]
          i -> [w1724]
          stop <- w1736 stop-if-true
          n448 = call "merFISH_scan_single_step.vi"("iteration"=w1724, "queue DAQ"=w1726, "error in"=w1727, "Z position"=w1728, "# steps"=w1723, "queue piezo"=w1725) -> ("error out"=w1721:errorcluster)  [unwired: 2 in]
          n449 = Increment(x=w1724) -> (x+1=w1729:i32)
          n450 = Increment(x=w1724) -> (x+1=w1722:i32)
          n451 = Multiply(x=w1729, y=100) -> (x*y=w1732:i32)
          n452 = Equal?(x=w1723, y=w1722) -> (x = y?=w1720:bool)
          n453 = To Double Precision Float(number=w1732) -> (double precision float=w1734:dbl)
          n454 = To Double Precision Float(number=w1723) -> (double precision float=w1735:dbl)
          n455 = Divide(x=w1734, y=w1735) -> (x/y=w1733:dbl)
          n456 = To Unsigned Byte Integer(number=w1733) -> (unsigned 8bit integer=w1730:u8)
          n457 = local write "Number steps"(w1729) -> ()
          n458 = local write "Scan slider"(w1730) -> ()
          n459 = case shown="True" w1720 {
            tunnel: w1721 -> [w1737 w1747]
            tunnel: w1719 -> [_ w1744]
            tunnel: w1718 -> [_ w1745]
            tunnel: [w1737 w1746] -> w1717
            tunnel: w1716 -> [_ w1743]
            tunnel: w1715 -> [_ w1742]
            tunnel: w1714 -> [_ w1741]
            tunnel: w1713 -> [_ w1740]
            tunnel: w1712 -> [_ w1739]
            tunnel: w1711 -> [_ w1738]
            frame False {
            }
            frame True {
              n460 = call "merFISH_save_scan_and_prepare next.vi"("List probe Refnum"=w1743, "PATH cluster"=w1738, "queue CAMERA"=w1745, "queue piezo"=w1744, "error in"=w1747, "Global parameters"=w1739, "ROI list Refnum"=w1742, "Laser list Refnum"=w1741, "Data"=w1740) -> ("error out"=w1746:errorcluster)  [unwired: 2 in]
            }
          }
          n461 = global read "Global_ABORT.vi" "ABORT"() -> (w1736:bool)
        }
        n462 = Unbundle By Name(w1684) -> ("Log file"=w1686:refnum<file>, "Starting time"=w1687:dbl)
        n463 = Merge Errors(w1697, w1698) -> (w1694:errorcluster)
        n464 = call "merFISH_read_next_task_TDMS.vi"("error in"=w1694, "Starting time"=w1687, "Log file"=w1686) -> ("error out"=w1696:errorcluster, "task"=w1695:T11)  [unwired: 1 in]
      }
      frame "Main_merFISH_send_email" {
        n465 = global read "Global_MAIN.vi" "Alert email adress"() -> (w1767:string)
        n466 = Variant To Data(error in=w1779, type=0, Variant=w1776) -> (data=w1781:i32, error out=w1771:errorcluster)
        n467 = xnode "Match Regular Expression"("input string"=w1767, "regular expression"="@", "error in"=w1771) -> ("whole match"=w1769:string, "error out"=w1770:errorcluster)  [unwired: 3 in, 3 out]
        n468 = String Length(string=w1769) -> (length=w1766:i32)
        n469 = Equal?(x=1 ("y"), y=w1766) -> (x = y?=w1768:bool)
        n470 = case shown="True" w1768 {
          tunnel: [w1789 w1795] -> w1782
          tunnel: w1781 -> [_ w1794]
          tunnel: w1770 -> [w1789 w1791]
          tunnel: w1767 -> [_ w1790]
          frame False {
          }
          frame True {
            n471 = property on="Probe list" class="MCListbox (strict)"(error in=w1791) -> ("ItemNames"=w1792:string[][])  [unwired: 1 in, 2 out]
            n472 = call "merFISH_email_title.vi"("Probe number"=w1794, "Item Names"=w1792) -> ("Title"=w1793:string)  [unwired: 1 in]
            n473 = call "Send Email"("Subject"=w1793, "Recipients"=w1790) -> ("error out"=w1795:errorcluster)  [unwired: 9 in]
          }
        }
        n474 = Unbundle By Name(w1773) -> ("Log file"=w1774:refnum<file>, "Starting time"=w1775:dbl)
        n475 = call "merFISH_read_next_task_TDMS.vi"("error in"=w1782, "Starting time"=w1775, "Log file"=w1774) -> ("error out"=w1778:errorcluster, "task"=w1777:T11)  [unwired: 1 in]
      }
      frame "Main_merFISH_photobleaching_injection" {
        n476 = Unbundle By Name(w1917) -> ("Photobleaching procedure"=w1915:i32[][], "Log file"=w1914:refnum<file>, "Starting time"=w1913:dbl)
        n477 = Bundle By Name(cluster=T29 {"Photobleaching procedure"=[], "Log file"=refnum, "Starting time"=0.0} ("Data cluster"), "Photobleaching procedure"=w1915, "Log file"=w1914, "Starting time"=w1913) -> (w1912:T29)
        n478 = control-ref of="Valve position OUT"() -> (w1919:refnum<vi>)
        n479 = control-ref of="Photobleaching manager"() -> (w1921:refnum<vi>)
        n480 = control-ref of="Valve H"() -> (w1920:refnum<vi>)
        n481 = call "MAIN_merFISH_photobleaching_injections.vi"("Data cluster"=w1912, "queue valve"=w1911, "queue pump"=w1910, "Valve H"=w1918, "error in"=w1924, "Photobleaching manager Refnum"=w1921, "Valve Refnum"=w1920, "Valve position OUT Refnum"=w1919) -> ("Next task"=w1922:T11, "error out"=w1923:errorcluster)  [unwired: 6 in]
      }
      frame "Main_merFISH_close" {
        n482 = call "merFISH_close.vi"("queue DAQ"=w1944, "queue ASI stage"=w1946, "queue FPGA"=w1935, "queue CAMERA"=w1945, "queue pump"=w1940, "queue piezo"=w1941, "error in"=w1942, "Measure QPD"=w1934) -> ("error out"=w1943:errorcluster)  [unwired: 7 in]
        n483 = flat-sequence {
          tunnel: w1943 -> [w1965]
          tunnel: [w1965] -> w1939
          frame #0 {
            w1964 = FALSE ("merFISH")
            n484 = local write "Autofocus lost"(w1964) -> ()
            n485 = local write "Abort merFISH"(w1964) -> ()
            n486 = global write "Global_ABORT.vi" "ABORT"(w1964) -> ()
            n487 = local write "merFISH"(w1964) -> ()
          }
        }
        n488 = global read "Global_MAIN.vi" "Alert email adress"() -> (w1931:string)
        n489 = Equal?(x="", y=w1931) -> (x = y?=w1932:bool)
        n490 = case shown="False" w1932 {
          tunnel: w1939 -> [w1957 w1958]
          tunnel: [w1956 w1958] -> w1938
          tunnel: w1931 -> [w1955 _]
          frame False {
            n491 = call "Send Email2"("error in"=w1957, "Recipients"=w1955) -> ("error out"=w1956:errorcluster)  [unwired: 9 in]
          }
          frame True {
          }
        }
        n492 = case shown="False" w1936 {
          tunnel: [w1960 T11 {"variant"=variant, "Instruction"=enum."Main_STOP"} ("Q_main_element")] -> w1948
          tunnel: w1947 -> [w1959 _]
          frame False {
            n493 = case shown="True" w1959 {
              tunnel: [T11 {"variant"=variant, "Instruction"=enum."Main_not_acquiring"} ("Q_main_element") T11 {"variant"=variant, "Instruction"=enum."Main_start_acquiring"} ("Q_main_element")] -> w1960
              frame False {
              }
              frame True {
              }
            }
          }
          frame True {
          }
        }
      }
      frame "Main_STOP" {
        n494 = Close Reference(reference=w1974, error in (no error)=w1975) -> (error out=w1973:errorcluster)
        n495 = Close Reference(reference=w1972, error in (no error)=w1973) -> (error out=w1971:errorcluster)
        n496 = Close Reference(reference=w1970, error in (no error)=w1971) -> (error out=w1969:errorcluster)
        n497 = Close Reference(reference=w1968, error in (no error)=w1969) -> (error out=w1966:errorcluster)
        n498 = call "IMAQ Dispose"("Image"=w1994, "error in (no error)"=w1966) -> ("error out"=w1993:errorcluster)  [unwired: 4 in]
        n499 = call "IMAQ Dispose"("Image"=w1992, "error in (no error)"=w1993) -> ("error out"=w1983:errorcluster)  [unwired: 4 in]
        n500 = for {
          tunnel: w1983 -> [w2001]
          tunnel: w1982 -> [w2000] mode=indexing
          tunnel: [w1999] -> w1981
          n501 = Close Reference(reference=w2000, error in (no error)=w2001) -> (error out=w1999:errorcluster)
        }
        n502 = call "MAIN_Shut_down.vi"("queue FPGA"=w1967, "Q_pump"=w1978, "Start acquisition"=w1977, "Q_valve"=w1979, "Q_DAQ"=w1984, "error in"=w1981, "Q_CAMERA"=w1985, "Q_ASI"=w1986, "Q_piezo"=w1987) -> ("error out"=w1989:errorcluster)  [unwired: 2 in]
        n503 = flat-sequence {
          tunnel: w1989 -> [w2002]
          tunnel: [w2002] -> w1988
          frame #0 {
            n504 = global write "Global_MAIN.vi" "Stop main vi"(TRUE ("Stop main vi")) -> ()
          }
        }
      }
    }
    "Kin time (s)" <- w129
    "XY positions" <- w111
    "Error" <- w101
    n505 = Unbundle By Name(w77) -> ("merFISH init"=→"merFISH init":T6)
    n506 = To Variant(anything=w103) -> (Variant=w106:variant)
    n507 = Bundle By Name(cluster=T11 {"variant"=variant, "Instruction"=enum."Main_error"} ("Q_main_element"), "variant"=w106) -> (w104:T11)
    n508 = case shown="No Error" w103 {
      tunnel: w137 -> [w141 _]
      tunnel: [w140 w142] -> w136
      tunnel: [w139 w145] -> w135
      tunnel: w75 -> [w138 w144]
      tunnel: w104 -> [_ w143]
      frame No Error {
        n509 = Enqueue Element(queue=w138, element=w141) -> (queue out=w140:refnum<queue>, error out=w139:errorcluster)  [unwired: 2 in, 1 out]
      }
      frame Error {
        n510 = Enqueue Element(queue=w144, element=w143) -> (queue out=w142:refnum<queue>, error out=w145:errorcluster)  [unwired: 2 in, 1 out]
      }
    }
    "Global parameters" <- w120
    "Initialization status" <- w116
  }
  n511 = control-ref of="Illumination controls"() -> (w31:refnum<vi>)
  n512 = while {
    tunnel: w8 -> [w2017]
    tunnel: w6 -> [w2015]
    shift-right: [w2007] -> _
    shift-left: w1 -> [w2016]
    tunnel: w10 -> [w2014]
    tunnel: w31 -> [w2013]
    tunnel: w11 -> [w2012]
    tunnel: w5 -> [w2009]
    tunnel: w7 -> [w2010]
    tunnel: w4 -> [w2004]
    stop <- w2019 stop-if-true
    n513 = local read "Initialization status"() -> (w2011:T3)
    n514 = local read "Autofocus lost"() -> (w2005:bool)
    n515 = event shown="[0] Timeout" {
      selector: _ -> [_ _ _ _ _ _ _ _ _ _ _ _ _ _ _ _ _ _ _ _ _ _ _ _ _ _ _ _ _ _ _ _ _ _ _ _ _ _ _ _ _ _]
      dyn-events: _ -> [_ _ _ _ _ _ _ _ _ _ _ _ _ _ _ _ _ _ _ _ _ _ _ _ _ _ _ _ _ _ _ _ _ _ _ _ _ _ _ _ _ _]
      timeout: 100 -> [_ _ _ _ _ _ _ _ _ _ _ _ _ _ _ _ _ _ _ _ _ _ _ _ _ _ _ _ _ _ _ _ _ _ _ _ _ _ _ _ _ _]
      tunnel: w2017 -> [_ w2023 _ w2050 w2059 w2070 w2089 w2108 w2127 w2146 _ w2192 w2210 w2228 w2246 w2260 w2267 w2278 _ _ w2340 w2352 w2368 _ w2404 w2421 _ w2452 _ _ _ _ _ _ _ _ w2511 w2523 w2544 w2571 _ w2592]
      tunnel: w2016 -> [w2020 w2022 w2045 w2049 w2061 w2069 w2088 w2107 w2126 w2144 w2168 w2191 w2209 w2227 w2245 w2261 w2268 w2279 w2299 w2316 w2341 w2354 w2375 w2393 w2407 w2423 w2433 w2453 w2466 w2471 w2476 w2479 w2490 w2497 w2503 w2508 w2512 w2522 w2545 w2572 w2587 w2589]
      tunnel: [w2020 w2021 w2034 w2048 w2060 w2068 w2087 w2106 w2125 w2143 w2166 w2190 w2208 w2226 w2244 w2256 w2266 w2277 w2297 w2315 w2342 w2353 w2374 w2391 w2406 w2422 w2432 w2448 w2466 w2469 w2475 w2477 w2489 w2496 w2502 w2507 w2510 w2521 w2543 w2570 w2587 w2590] -> w2007
      tunnel: w2015 -> [_ _ _ _ _ _ _ _ _ _ _ _ _ _ _ _ _ _ _ _ _ _ _ _ _ _ _ _ _ _ _ _ _ _ _ _ _ _ _ _ _ _]
      tunnel: w2014 -> [_ _ _ _ _ _ _ _ _ _ w2165 _ _ _ _ _ _ _ _ _ _ _ _ _ _ _ _ _ _ _ _ _ _ _ _ _ _ _ _ _ _ _]
      tunnel: w2013 -> [_ _ _ _ _ _ _ _ _ _ w2164 _ _ _ _ _ _ _ _ w2310 _ _ _ _ _ _ _ _ _ _ _ _ _ _ _ _ _ _ _ _ _ _]
      tunnel: w2012 -> [_ _ _ _ _ _ _ _ _ _ _ _ _ _ _ _ _ _ w2298 _ _ _ _ w2394 _ _ _ _ _ _ _ _ _ _ _ _ _ _ _ _ _ _]
      tunnel: w2011 -> [_ _ _ w2047 _ w2067 w2086 w2105 w2124 w2142 w2163 w2189 w2207 w2225 w2243 _ _ _ w2296 w2313 w2339 w2351 w2372 _ w2409 w2425 w2436 w2451 _ _ _ _ _ _ _ _ _ w2519 w2542 w2568 _ _]
      tunnel: w2010 -> [_ _ _ _ _ _ _ _ _ _ _ _ _ _ _ _ _ _ _ _ _ _ _ _ _ _ w2434 _ _ _ _ _ _ _ _ _ _ _ _ _ _ _]
      tunnel: w2009 -> [_ _ _ _ _ _ _ _ _ _ _ _ _ _ _ _ _ _ _ _ _ _ _ _ _ _ _ _ _ _ _ _ _ _ _ _ _ _ _ _ _ _]
      tunnel: "Autofocus" -> [_ _ _ _ _ _ _ _ _ _ _ _ _ _ _ _ _ _ w2295 _ _ _ _ w2390 _ _ _ _ _ _ _ _ _ _ _ _ _ _ _ _ _ _]
      tunnel: "merFISH" -> [_ _ _ _ _ _ _ _ _ _ _ _ _ _ _ _ _ _ w2294 _ _ _ _ _ _ _ _ _ _ _ _ _ _ _ _ _ _ _ _ _ _ _]
      tunnel: w2005 -> [_ _ _ _ _ _ _ _ _ _ _ _ _ _ _ _ _ _ w2287 _ _ _ _ _ _ _ _ _ _ _ _ _ _ _ _ _ _ _ _ _ _ _]
      tunnel: w2004 -> [_ _ _ _ _ _ _ _ _ _ w2161 _ _ _ _ _ _ _ _ w2311 _ _ _ _ _ _ _ _ _ _ _ _ _ _ _ _ _ _ _ _ _ _]
      event Timeout {
        n516 = event-data() -> ()  [unwired: 1 in, 1 out]
      }
      event "Initialized": Value Change {
        n517 = event-data() -> ("NewVal"=w2024:bool)  [unwired: 1 in]
        n518 = case shown="True" w2024 {
          tunnel: w2023 -> [_ w2031]
          tunnel: w2022 -> [w2025 w2030]
          tunnel: [w2025 w2027] -> w2021
          frame False {
          }
          frame True {
            n519 = Flush Queue(queue=w2031, error in (no error)=w2030) -> (queue out=w2029:refnum<queue>, error out=w2028:errorcluster)  [unwired: 1 out]
            n520 = Enqueue Element(queue=w2029, element=T11 {"variant"=variant, "Instruction"=enum."Main_initialize"}, error in (no error)=w2028) -> (error out=w2027:errorcluster)  [unwired: 1 in, 2 out]
          }
        }
      }
      event "Saving path": Value Change {
        # "When the saving path is changed, the\nTDMS file is copied in the new folder and the\nnew reference is saved."
        n521 = event-data() -> ("OldVal"=w2042:path, "NewVal"=w2040:path)  [unwired: 1 in]
        n522 = global read "Global_MAIN.vi" "tdms file out"() -> (w2044:refnum<k34>)
        n523 = TDMS Close(8:w2045, 11:w2044) -> (0:w2043:errorcluster)  [unwired: 1 out]
        n524 = call "MAIN_TDMS_save_path_definition.vi"("error in"=w2043, "Path to the saving folder"=w2042) -> ("error out"=w2041:errorcluster, "path to tdms file"=w2032:path)  [unwired: 4 in, 1 out]
        n525 = call "MAIN_TDMS_save_path_definition.vi"("error in"=w2041, "Path to the saving folder"=w2040) -> ("error out"=w2036:errorcluster, "path to tdms file"=w2033:path)  [unwired: 4 in, 1 out]
        n526 = Copy(8:w2036, 10:w2033, 11:w2032) -> (0:w2037:errorcluster, 3:w2038:path)  [unwired: 2 in, 1 out]
        n527 = TDMS Open(8:w2037, 10:T37."open" ("operation (0:open)"), 11:w2038) -> (0:w2034:errorcluster, 3:w2035:refnum<k34>)  [unwired: 4 in]
        n528 = global write "Global_MAIN.vi" "tdms file out"(w2035) -> ()
      }
      event "Exp time (s)": Value Change {
        n529 = event-data() -> ()  [unwired: 1 in, 1 out]
        n530 = Unbundle By Name(w2047) -> ("Camera"=w2046:bool)
        n531 = case shown="True" w2046 {
          tunnel: w2050 -> [_ w2057]
          tunnel: w2049 -> [w2052 w2055]
          tunnel: [w2051 w2053] -> w2048
          frame False {
            n532 = call "Display Message to User5"("error in (no error)"=w2052) -> ("error out"=w2051:errorcluster)  [unwired: 9 in, 1 out]
          }
          frame True {
            n533 = Flush Queue(queue=w2057, error in (no error)=w2055) -> (queue out=w2056:refnum<queue>, error out=w2054:errorcluster)  [unwired: 1 out]
            n534 = Enqueue Element(queue=w2056, element=T11 {"variant"=variant, "Instruction"=enum."Main_change_exposure"} ("Q_main_element"), error in (no error)=w2054) -> (error out=w2053:errorcluster)  [unwired: 1 in, 2 out]
          }
        }
      }
      event "Total  range (nm)", "step length (nm)": Value Change {
        n535 = event-data() -> ()  [unwired: 1 in, 2 out]
        n536 = Flush Queue(queue=w2059, error in (no error)=w2061) -> (queue out=w2063:refnum<queue>, error out=w2062:errorcluster)  [unwired: 1 out]
        n537 = Enqueue Element(queue=w2063, element=T11 {"variant"=variant, "Instruction"=enum."Main_change_z_scan_parameters"} ("Q_main_element"), error in (no error)=w2062) -> (error out=w2060:errorcluster)  [unwired: 1 in, 2 out]
      }
      event "Set roi": Value Change {
        n538 = event-data() -> ()  [unwired: 1 in, 1 out]
        n539 = Unbundle By Name(w2067) -> ("Camera"=w2066:bool)
        n540 = case shown="True" w2066 {
          tunnel: w2070 -> [_ w2076]
          tunnel: w2069 -> [w2072 w2075]
          tunnel: [w2071 w2074] -> w2068
          tunnel: "Set roi" -> [_ w2073]
          frame False {
            n541 = call "Display Message to User4"("error in (no error)"=w2072) -> ("error out"=w2071:errorcluster)  [unwired: 9 in, 1 out]
          }
          frame True {
            n542 = case shown="True" w2073 {
              tunnel: w2076 -> [_ w2083]
              tunnel: w2075 -> [w2077 w2080]
              tunnel: [w2077 w2078] -> w2074
              frame False {
              }
              frame True {
                n543 = Flush Queue(queue=w2083, error in (no error)=w2080) -> (queue out=w2081:refnum<queue>, error out=w2079:errorcluster)  [unwired: 1 out]
                n544 = Enqueue Element(queue=w2081, element=T11 {"variant"=variant, "Instruction"=enum."Main_define_ROI"} ("Q_main_element"), error in (no error)=w2079) -> (error out=w2078:errorcluster)  [unwired: 1 in, 2 out]
              }
            }
          }
        }
      }
      event "Save embryo": Value Change {
        n545 = event-data() -> ()  [unwired: 1 in, 1 out]
        n546 = Unbundle By Name(w2086) -> ("Camera"=w2085:bool)
        n547 = case shown="True" w2085 {
          tunnel: w2089 -> [_ w2095]
          tunnel: w2088 -> [w2091 w2094]
          tunnel: [w2090 w2093] -> w2087
          tunnel: "Save embryo" -> [_ w2092]
          frame False {
            n548 = call "Display Message to User35"("error in (no error)"=w2091) -> ("error out"=w2090:errorcluster)  [unwired: 9 in, 1 out]
          }
          frame True {
            n549 = case shown="True" w2092 {
              tunnel: w2095 -> [_ w2102]
              tunnel: w2094 -> [w2096 w2099]
              tunnel: [w2096 w2097] -> w2093
              frame False {
              }
              frame True {
                n550 = Flush Queue(queue=w2102, error in (no error)=w2099) -> (queue out=w2100:refnum<queue>, error out=w2098:errorcluster)  [unwired: 1 out]
                n551 = Enqueue Element(queue=w2100, element=T11 {"variant"=variant, "Instruction"=enum."Main_merFISH_save_embryo_ROI"} ("Q_main_element"), error in (no error)=w2098) -> (error out=w2097:errorcluster)  [unwired: 1 in, 2 out]
              }
            }
          }
        }
      }
      event "Define mosaic": Value Change {
        n552 = event-data() -> ()  [unwired: 1 in, 1 out]
        n553 = Unbundle By Name(w2105) -> ("Camera"=w2104:bool)
        n554 = case shown="True" w2104 {
          tunnel: w2108 -> [_ w2114]
          tunnel: w2107 -> [w2110 w2113]
          tunnel: [w2109 w2112] -> w2106
          tunnel: "Define mosaic" -> [_ w2111]
          frame False {
            n555 = call "Display Message to User9"("error in (no error)"=w2110) -> ("error out"=w2109:errorcluster)  [unwired: 9 in, 1 out]
          }
          frame True {
            n556 = case shown="True" w2111 {
              tunnel: w2114 -> [_ w2121]
              tunnel: w2113 -> [w2115 w2118]
              tunnel: [w2115 w2116] -> w2112
              frame False {
              }
              frame True {
                n557 = Flush Queue(queue=w2121, error in (no error)=w2118) -> (queue out=w2119:refnum<queue>, error out=w2117:errorcluster)  [unwired: 1 out]
                n558 = Enqueue Element(queue=w2119, element=T11 {"variant"=variant, "Instruction"=enum."Main_define_mosaic"} ("Q_main_element"), error in (no error)=w2117) -> (error out=w2116:errorcluster)  [unwired: 1 in, 2 out]
              }
            }
          }
        }
      }
      event "Reset roi": Value Change {
        n559 = event-data() -> ("NewVal"=w2122:bool)  [unwired: 1 in]
        n560 = Unbundle By Name(w2124) -> ("Camera"=w2123:bool)
        n561 = case shown="True" w2123 {
          tunnel: w2127 -> [_ w2133]
          tunnel: w2126 -> [w2129 w2132]
          tunnel: [w2128 w2131] -> w2125
          tunnel: w2122 -> [_ w2130]
          frame False {
            n562 = call "Display Message to User7"("error in (no error)"=w2129) -> ("error out"=w2128:errorcluster)  [unwired: 9 in, 1 out]
          }
          frame True {
            n563 = case shown="True" w2130 {
              tunnel: w2133 -> [_ w2140]
              tunnel: w2132 -> [w2134 w2137]
              tunnel: [w2134 w2135] -> w2131
              frame False {
              }
              frame True {
                n564 = Flush Queue(queue=w2140, error in (no error)=w2137) -> (queue out=w2138:refnum<queue>, error out=w2136:errorcluster)  [unwired: 1 out]
                n565 = Enqueue Element(queue=w2138, element=T11 {"variant"=variant, "Instruction"=enum."Main_define_ROI"} ("Q_main_element"), error in (no error)=w2136) -> (error out=w2135:errorcluster)  [unwired: 1 in, 2 out]
              }
            }
          }
        }
      }
      event "Start acquisition": Value Change {
        n566 = event-data() -> ("NewVal"=w2145:bool)  [unwired: 1 in]
        n567 = Unbundle By Name(w2142) -> ("Camera"=w2141:bool)
        n568 = case shown="True" w2141 {
          tunnel: w2146 -> [_ w2152]
          tunnel: w2145 -> [_ w2151]
          tunnel: w2144 -> [w2148 w2150]
          tunnel: [w2147 w2149] -> w2143
          frame False {
            n569 = call "Display Message to User2"("error in (no error)"=w2148) -> ("error out"=w2147:errorcluster)  [unwired: 9 in, 1 out]
          }
          frame True {
            n570 = case shown="True" w2151 {
              tunnel: w2152 -> [w2154 w2158]
              tunnel: w2150 -> [w2153 w2157]
              tunnel: [w2155 w2159] -> w2149
              frame False {
                n571 = Enqueue Element At Opposite End(queue=w2154, element=T11 {"variant"=variant, "Instruction"=enum."Main_stop_acquiring"} ("Q_main_element"), error in (no error)=w2153) -> (error out=w2155:errorcluster)  [unwired: 1 in, 2 out]
              }
              frame True {
                n572 = Enqueue Element At Opposite End(queue=w2158, element=T11 {"variant"=variant, "Instruction"=enum."Main_start_acquiring"} ("Q_main_element"), error in (no error)=w2157) -> (error out=w2159:errorcluster)  [unwired: 1 in, 2 out]
              }
            }
          }
        }
      }
      event Value Change {
        n573 = event-data() -> ("NewVal"=w2167:T4, "OldVal"=w2169:T4)  [unwired: 1 in]
        n574 = Unbundle By Name(w2163) -> ("FPGA"=w2162:bool)
        n575 = case shown="True" w2162 {
          tunnel: w2161 -> [_ w2178]
          tunnel: w2169 -> [_ w2177]
          tunnel: w2168 -> [w2171 w2176]
          tunnel: w2167 -> [_ w2175]
          tunnel: [w2170 w2174] -> w2166
          tunnel: w2165 -> [_ w2173]
          tunnel: w2164 -> [_ w2172]
          frame False {
            n576 = call "Display Message to User11"("error in (no error)"=w2171) -> ("error out"=w2170:errorcluster)  [unwired: 9 in, 1 out]
          }
          frame True {
            n577 = call "DAQ_compare_illumination_controls_clusters.vi"("Illumination controls OLD"=w2177, "Illumination controls NEW"=w2175, "error in"=w2176) -> ("Array"=w2180:i32[], "error out"=w2179:errorcluster)
            n578 = for {
              tunnel: w2180 -> [w2184] mode=indexing
              tunnel: w2179 -> [w2185]
              tunnel: w2178 -> [w2181]
              tunnel: w2175 -> [w2186]
              tunnel: [w2183] -> w2174
              tunnel: w2173 -> [w2187]
              tunnel: w2172 -> [w2182]
              n579 = call "MAIN_change_illumination.vi"("Illumination Refnum"=w2182, "task number"=w2184, "error in"=w2185, "Illumination control"=w2186, "queue ASI stage"=w2187, "queue FPGA"=w2181) -> ("error out"=w2183:errorcluster)  [unwired: 5 in]
            }
          }
        }
      }
      event "Save X/Y position": Value Change {
        n580 = event-data() -> ()  [unwired: 1 in, 1 out]
        n581 = Unbundle By Name(w2189) -> ("ASI"=w2188:bool)
        n582 = case shown="True" w2188 {
          tunnel: w2192 -> [_ w2198]
          tunnel: w2191 -> [w2194 w2197]
          tunnel: [w2193 w2195] -> w2190
          frame False {
            n583 = call "Display Message to User17"("error in (no error)"=w2194) -> ("error out"=w2193:errorcluster)  [unwired: 9 in, 1 out]
          }
          frame True {
            n584 = case shown="True" "Save X/Y position" {
              tunnel: w2198 -> [_ w2202]
              tunnel: w2197 -> [w2199 w2201]
              tunnel: [w2199 w2200] -> w2195
              frame False {
              }
              frame True {
                n585 = Flush Queue(queue=w2202, error in (no error)=w2201) -> (queue out=w2204:refnum<queue>, error out=w2203:errorcluster)  [unwired: 1 out]
                n586 = Enqueue Element(queue=w2204, element=T11 {"variant"=variant, "Instruction"=enum."Main_save_XY"} ("Q_main_element"), error in (no error)=w2203) -> (error out=w2200:errorcluster)  [unwired: 1 in, 2 out]
              }
            }
          }
        }
      }
      event "Load X/Y positions": Value Change {
        n587 = event-data() -> ()  [unwired: 1 in, 1 out]
        n588 = Unbundle By Name(w2207) -> ("ASI"=w2206:bool)
        n589 = case shown="True" w2206 {
          tunnel: w2210 -> [_ w2216]
          tunnel: w2209 -> [w2212 w2215]
          tunnel: [w2211 w2214] -> w2208
          frame False {
            n590 = call "Display Message to User18"("error in (no error)"=w2212) -> ("error out"=w2211:errorcluster)  [unwired: 9 in, 1 out]
          }
          frame True {
            n591 = case shown="True" "Load X/Y positions" {
              tunnel: w2216 -> [_ w2220]
              tunnel: w2215 -> [w2217 w2219]
              tunnel: [w2217 w2218] -> w2214
              frame False {
              }
              frame True {
                n592 = Flush Queue(queue=w2220, error in (no error)=w2219) -> (queue out=w2222:refnum<queue>, error out=w2221:errorcluster)  [unwired: 1 out]
                n593 = Enqueue Element(queue=w2222, element=T11 {"variant"=variant, "Instruction"=enum."Main_load_XY"} ("Q_main_element"), error in (no error)=w2221) -> (error out=w2218:errorcluster)  [unwired: 1 in, 2 out]
              }
            }
          }
        }
      }
      event "Discard ROIs": Value Change {
        n594 = event-data() -> ()  [unwired: 1 in, 1 out]
        n595 = Unbundle By Name(w2225) -> ("ASI"=w2224:bool)
        n596 = case shown="True" w2224 {
          tunnel: w2228 -> [_ w2234]
          tunnel: w2227 -> [w2230 w2233]
          tunnel: [w2229 w2232] -> w2226
          frame False {
            n597 = call "Display Message to User19"("error in (no error)"=w2230) -> ("error out"=w2229:errorcluster)  [unwired: 9 in, 1 out]
          }
          frame True {
            n598 = case shown="True" "Discard ROIs" {
              tunnel: w2234 -> [_ w2238]
              tunnel: w2233 -> [w2235 w2237]
              tunnel: [w2235 w2236] -> w2232
              frame False {
              }
              frame True {
                n599 = Flush Queue(queue=w2238, error in (no error)=w2237) -> (queue out=w2240:refnum<queue>, error out=w2239:errorcluster)  [unwired: 1 out]
                n600 = Enqueue Element(queue=w2240, element=T11 {"variant"=variant, "Instruction"=enum."Main_discard_XY"} ("Q_main_element"), error in (no error)=w2239) -> (error out=w2236:errorcluster)  [unwired: 1 in, 2 out]
              }
            }
          }
        }
      }
      event "ROI manager": Double Click {
        n601 = event-data() -> ()  [unwired: 1 in, 1 out]
        n602 = Unbundle By Name(w2243) -> ("ASI"=w2242:bool)
        n603 = case shown="True" w2242 {
          tunnel: w2246 -> [_ w2251]
          tunnel: w2245 -> [w2248 w2250]
          tunnel: [w2247 w2249] -> w2244
          frame False {
            n604 = call "Display Message to User23"("error in (no error)"=w2248) -> ("error out"=w2247:errorcluster)  [unwired: 9 in, 1 out]
          }
          frame True {
            n605 = Flush Queue(queue=w2251, error in (no error)=w2250) -> (queue out=w2253:refnum<queue>, error out=w2252:errorcluster)  [unwired: 1 out]
            n606 = Enqueue Element(queue=w2253, element=T11 {"variant"=variant, "Instruction"=enum."Main_move_to_XY"} ("Q_main_element"), error in (no error)=w2252) -> (error out=w2249:errorcluster)  [unwired: 1 in, 2 out]
          }
        }
      }
      event "Illumination source", "Select laser lines": Value Change {
        n607 = event-data() -> ("NewVal"=w2255:bool)  [unwired: 1 in]
        n608 = Flush Queue(queue=w2260, error in (no error)=w2261) -> (queue out=w2263:refnum<queue>, error out=w2262:errorcluster)  [unwired: 1 out]
        n609 = Enqueue Element(queue=w2263, element=T11 {"variant"=variant, "Instruction"=enum."Main_merFISH_illumination_parameters"} ("Q_main_element"), error in (no error)=w2262) -> (error out=w2257:errorcluster)  [unwired: 1 in, 2 out]
        n610 = To Variant(anything=w2255) -> (Variant=w2259:variant)
        n611 = call "MAIN_save_parameters_TDMS.vi"("error in"=w2257, "Data"=w2259, "Channel name"="Illumination source" ("group name")) -> ("error out"=w2256:errorcluster)  [unwired: 2 in]
      }
      event "DAPI": Value Change {
        n612 = event-data() -> ()  [unwired: 1 in, 1 out]
        n613 = case shown="False" "DAPI" {
          tunnel: w2268 -> [w2269 w2272]
          tunnel: w2267 -> [_ w2271]
          tunnel: [w2269 w2270] -> w2266
          frame False {
          }
          frame True {
            n614 = Flush Queue(queue=w2271, error in (no error)=w2272) -> (queue out=w2274:refnum<queue>, error out=w2273:errorcluster)  [unwired: 1 out]
            n615 = Enqueue Element(queue=w2274, element=T11 {"variant"=variant, "Instruction"=enum."Main_merFISH_DAPI_parameters"} ("Q_main_element"), error in (no error)=w2273) -> (error out=w2270:errorcluster)  [unwired: 1 in, 2 out]
          }
        }
      }
      event "Brightfield": Value Change {
        n616 = event-data() -> ()  [unwired: 1 in, 1 out]
        n617 = case shown="True" "Brightfield" {
          tunnel: w2279 -> [w2280 w2283]
          tunnel: w2278 -> [_ w2282]
          tunnel: [w2280 w2281] -> w2277
          frame False {
          }
          frame True {
            n618 = Flush Queue(queue=w2282, error in (no error)=w2283) -> (queue out=w2285:refnum<queue>, error out=w2284:errorcluster)  [unwired: 1 out]
            n619 = Enqueue Element(queue=w2285, element=T11 {"variant"=variant, "Instruction"=enum."Main_merFISH_Brightfield_parameters"} ("Q_main_element"), error in (no error)=w2284) -> (error out=w2281:errorcluster)  [unwired: 1 in, 2 out]
          }
        }
      }
      event Key Down {
        n620 = event-data() -> ()  [unwired: 1 in, 1 out]
        n621 = Unbundle By Name(w2296) -> ("PiFoc"=w2291:bool)
        n622 = Not(x=w2295) -> (.not. x?=w2293:bool)
        n623 = Not(x=w2294) -> (.not. x?=w2292:bool)
        n624 = Build Array(w2291, w2293, w2292) -> (w2290:bool[])
        n625 = And Array Elements(Boolean array=w2290) -> (logical AND=w2289:bool)
        n626 = Or(x=w2289, y=w2287) -> (x .or. y?=w2288:bool)
        n627 = case shown="False" w2288 {
          tunnel: w2299 -> [w2300 w2307]
          tunnel: w2298 -> [_ w2306]
          tunnel: [w2300 w2305] -> w2297
          frame False {
          }
          frame True {
            n628 = Flush Queue(queue=w2306, error in (no error)=w2307) -> (queue out=w2309:refnum<queue>, error out=w2308:errorcluster)  [unwired: 1 out]
            n629 = To Variant(anything="Piezo step (um)") -> (Variant=w2303:variant)
            n630 = Bundle By Name(cluster=T13 {"variant"=variant, "Instruction"=enum."Piezo_keyboard_move"} ("element"), "variant"=w2303) -> (w2302:T13)
            n631 = Enqueue Element(queue=w2309, element=w2302, error in (no error)=w2308) -> (error out=w2305:errorcluster)  [unwired: 1 in, 2 out]
          }
        }
      }
      event "Measure QPD": Value Change {
        n632 = event-data() -> ("NewVal"=w2314:bool)  [unwired: 1 in]
        n633 = Unbundle By Name(w2313) -> ("FPGA"=w2312:bool)
        n634 = case shown="True" w2312 {
          tunnel: w2316 -> [w2318 w2335]
          tunnel: w2311 -> [_ w2334]
          tunnel: [w2317 w2324] -> w2315
          tunnel: w2314 -> [_ w2330]
          tunnel: w2310 -> [_ w2321]
          frame False {
            n635 = call "Display Message to User20"("error in (no error)"=w2318) -> ("error out"=w2317:errorcluster)  [unwired: 9 in, 1 out]
          }
          frame True {
            n636 = Flush Queue(queue=w2334, error in (no error)=w2335) -> (queue out=w2333:refnum<queue>, error out=w2332:errorcluster)  [unwired: 1 out]
            n637 = To Variant(anything=w2330) -> (Variant=w2331:variant)
            n638 = Bundle By Name(cluster=T38 {"variant"=variant, "Instruction"=enum."FPGA_start_stop_measure_QPD"} ("element"), "variant"=w2331) -> (w2328:T38)
            n639 = Enqueue Element(queue=w2333, element=w2328, error in (no error)=w2332) -> (queue out=w2322:refnum<queue>, error out=w2327:errorcluster)  [unwired: 1 in, 1 out]
            n640 = property class="Clust (strict)"(reference=w2321) -> (reference out=w2320:refnum<vi>, "Value"=w2319:T4)  [unwired: 1 in, 1 out]
            n641 = call "FPGA_wait_for_task_START.vi"("error in"=w2327) -> ("error out"=w2326:errorcluster)
            n642 = call "FPGA_wait_for_task_DONE.vi"("error in"=w2326) -> ("error out"=w2325:errorcluster)
            n643 = call "MAIN_change_illumination.vi"("Illumination Refnum"=w2320, "task number"=2, "error in"=w2325, "Illumination control"=w2319, "queue FPGA"=w2322) -> ("error out"=w2324:errorcluster)  [unwired: 6 in]
          }
        }
      }
      event "Save setpoint": Value Change {
        n644 = event-data() -> ()  [unwired: 1 in, 1 out]
        n645 = Unbundle By Name(w2339) -> ("FPGA"=w2338:bool)
        n646 = And(x=w2338, y="Save setpoint") -> (x .and. y?=w2337:bool)
        n647 = case shown="True" w2337 {
          tunnel: [w2343 w2347] -> w2342
          tunnel: w2341 -> [w2343 w2346]
          tunnel: w2340 -> [_ w2345]
          frame False {
          }
          frame True {
            n648 = Enqueue Element At Opposite End(queue=w2345, element=T11 {"variant"=variant, "Instruction"=enum."Main_merFISH_save_setpoint"}, error in (no error)=w2346) -> (error out=w2347:errorcluster)  [unwired: 1 in, 2 out]
          }
        }
      }
      event "Calib autofocus": Value Change {
        n649 = event-data() -> ()  [unwired: 1 in, 1 out]
        n650 = Unbundle By Name(w2351) -> ("DAQ"=w2349:bool, "PiFoc"=w2350:bool)
        n651 = And(x=w2349, y=w2350) -> (x .and. y?=w2348:bool)
        n652 = case shown="True" w2348 {
          tunnel: w2354 -> [w2356 w2360]
          tunnel: [w2355 w2359] -> w2353
          tunnel: w2352 -> [_ w2357]
          frame False {
            n653 = call "Display Message to User24"("error in (no error)"=w2356) -> ("error out"=w2355:errorcluster)  [unwired: 9 in, 1 out]
          }
          frame True {
            n654 = case shown="True" "Calib autofocus" {
              tunnel: w2360 -> [w2361 w2364]
              tunnel: [w2361 w2363] -> w2359
              tunnel: w2357 -> [_ w2362]
              frame False {
              }
              frame True {
                n655 = Flush Queue(queue=w2362, error in (no error)=w2364) -> (queue out=w2367:refnum<queue>, error out=w2366:errorcluster)  [unwired: 1 out]
                n656 = Enqueue Element(queue=w2367, element=T11 {"variant"=variant, "Instruction"=enum."Main_autofocus_calibration"}, error in (no error)=w2366) -> (error out=w2363:errorcluster)  [unwired: 1 in, 2 out]
              }
            }
          }
        }
      }
      event "Autofocus": Value Change {
        n657 = event-data() -> ("NewVal"=w2373:bool)  [unwired: 1 in]
        n658 = Unbundle By Name(w2372) -> ("FPGA"=w2370:bool, "PiFoc"=w2369:bool)
        n659 = And(x=w2370, y=w2369) -> (x .and. y?=w2371:bool)
        n660 = case shown="True" w2371 {
          tunnel: w2375 -> [w2377 w2381]
          tunnel: [w2376 w2380] -> w2374
          tunnel: w2368 -> [_ w2379]
          tunnel: w2373 -> [_ w2378]
          frame False {
            n661 = call "Display Message to User25"("error in (no error)"=w2377) -> ("error out"=w2376:errorcluster)  [unwired: 9 in, 1 out]
          }
          frame True {
            n662 = case shown="False" w2378 {
              tunnel: w2381 -> [w2383 w2388]
              tunnel: [w2385 w2389] -> w2380
              tunnel: w2379 -> [w2384 w2387]
              frame True {
                n663 = Enqueue Element At Opposite End(queue=w2384, element=T11 {"variant"=variant, "Instruction"=enum."Main_autofocus_initialization"}, error in (no error)=w2383) -> (error out=w2385:errorcluster)  [unwired: 1 in, 2 out]
              }
              frame False {
                n664 = Enqueue Element(queue=w2387, element=T11 {"variant"=variant, "Instruction"=enum."Main_autofocus_stop"}, error in (no error)=w2388) -> (error out=w2389:errorcluster)  [unwired: 1 in, 2 out]
              }
            }
          }
        }
      }
      event "Init": Value Change {
        n665 = event-data() -> ("NewVal"=w2392:bool)  [unwired: 1 in]
        n666 = case shown="True" w2390 {
          tunnel: w2394 -> [_ w2402]
          tunnel: w2393 -> [w2395 w2401]
          tunnel: w2392 -> [_ w2398]
          tunnel: [w2395 w2396] -> w2391
          frame False {
          }
          frame True {
            n667 = To Variant(anything=w2398) -> (Variant=w2399:variant)
            n668 = Bundle By Name(cluster=T13 {"variant"=variant, "Instruction"=enum."Piezo_change_init_state"} ("element"), "variant"=w2399) -> (w2397:T13)
            n669 = Enqueue Element At Opposite End(queue=w2402, element=w2397, error in (no error)=w2401) -> (error out=w2396:errorcluster)  [unwired: 1 in, 2 out]
          }
        }
      }
      event "Valve H": Value Change {
        n670 = event-data() -> ("NewVal"=w2403:u8, "OldVal"=w2405:u8)  [unwired: 1 in]
        n671 = Unbundle By Name(w2409) -> ("Valve"=w2408:bool)
        n672 = case shown="True" w2408 {
          tunnel: w2404 -> [_ w2420]
          tunnel: w2407 -> [w2411 w2419]
          tunnel: [w2410 w2416] -> w2406
          tunnel: w2403 -> [_ w2414]
          tunnel: w2405 -> [_ w2413]
          frame False {
            n673 = call "Display Message to User8"("error in (no error)"=w2411) -> ("error out"=w2410:errorcluster)  [unwired: 9 in, 1 out]
          }
          frame True {
            n674 = Bundle("NewVal"=w2414, "OldVal"=w2413) -> (w2415:cluster{"NewVal":u8, "OldVal":u8})  [unwired: 1 in]
            n675 = To Variant(anything=w2415) -> (Variant=w2418:variant)
            n676 = Bundle By Name(cluster=T11 {"variant"=variant, "Instruction"=enum."Main_change_H_valve_position"} ("element"), "variant"=w2418) -> (w2417:T11)
            n677 = Enqueue Element At Opposite End(queue=w2420, element=w2417, error in (no error)=w2419) -> (error out=w2416:errorcluster)  [unwired: 1 in, 2 out]
          }
        }
      }
      event "Two-way valve": Value Change {
        n678 = event-data() -> ()  [unwired: 1 in, 1 out]
        n679 = Unbundle By Name(w2425) -> ("DAQ"=w2424:bool)
        n680 = case shown="True" w2424 {
          tunnel: w2423 -> [w2427 w2431]
          tunnel: [w2426 w2430] -> w2422
          tunnel: w2421 -> [_ w2429]
          frame False {
            n681 = call "Display Message to User28"("error in (no error)"=w2427) -> ("error out"=w2426:errorcluster)  [unwired: 9 in, 1 out]
          }
          frame True {
            n682 = Enqueue Element At Opposite End(queue=w2429, element=T11 {"variant"=variant, "Instruction"=enum."Main_two_way_valve"}, error in (no error)=w2431) -> (error out=w2430:errorcluster)  [unwired: 1 in, 2 out]
          }
        }
      }
      event "Pressure (mbar)": Value Change {
        n683 = event-data() -> ()  [unwired: 1 in, 1 out]
        n684 = Unbundle By Name(w2436) -> ("Pump"=w2435:bool)
        n685 = case shown="False" w2435 {
          tunnel: w2434 -> [_ w2445]
          tunnel: w2433 -> [w2438 w2444]
          tunnel: [w2437 w2439] -> w2432
          frame False {
            n686 = call "Display Message to User10"("error in (no error)"=w2438) -> ("error out"=w2437:errorcluster)  [unwired: 9 in, 1 out]
          }
          frame True {
            n687 = To Variant(anything="Pressure (mbar)") -> (Variant=w2442:variant)
            n688 = Bundle By Name(cluster=T14 {"variant"=variant, "Instruction"=enum."PUMP_change_pressure"} ("element"), "variant"=w2442) -> (w2440:T14)
            n689 = Enqueue Element At Opposite End(queue=w2445, element=w2440, error in (no error)=w2444) -> (error out=w2439:errorcluster)  [unwired: 1 in, 2 out]
          }
        }
      }
      event "Define injections": Value Change {
        n690 = event-data() -> ()  [unwired: 1 in, 1 out]
        n691 = Unbundle By Name(w2451) -> ("Pump"=w2450:bool, "Valve"=w2449:bool)
        n692 = And(x=w2450, y=w2449) -> (x .and. y?=w2447:bool)
        n693 = case shown="True" w2447 {
          tunnel: w2453 -> [w2455 w2459]
          tunnel: w2452 -> [_ w2458]
          tunnel: [w2454 w2457] -> w2448
          tunnel: "Define injections" -> [_ w2456]
          frame False {
            n694 = call "Display Message to User16"("error in (no error)"=w2455) -> ("error out"=w2454:errorcluster)  [unwired: 9 in, 1 out]
          }
          frame True {
            n695 = case shown="True" w2456 {
              tunnel: w2459 -> [w2460 w2464]
              tunnel: w2458 -> [_ w2463]
              tunnel: [w2460 w2461] -> w2457
              frame False {
              }
              frame True {
                n696 = Enqueue Element At Opposite End(queue=w2463, element=T11 {"variant"=variant, "Instruction"=enum."Main_merFISH_injections_procedure"}, error in (no error)=w2464) -> (error out=w2461:errorcluster)  [unwired: 1 in, 2 out]
              }
            }
          }
        }
      }
      event "Autofocus automatic correction": Value Change {
        n697 = event-data() -> ()  [unwired: 1 in, 1 out]
        n698 = global write "Global_MAIN.vi" "Correct autofocus automatically"("Autofocus automatic correction") -> ()
      }
      event "Alert email adress": Value Change {
        n699 = event-data() -> ()  [unwired: 1 in, 1 out]
        n700 = global write "Global_MAIN.vi" "Alert email adress"("Alert email adress") -> ()
        n701 = To Variant(anything="Alert email adress") -> (Variant=w2468:variant)
        n702 = call "MAIN_save_parameters_TDMS.vi"("error in"=w2471, "Data"=w2468, "Channel name"="email address" ("group name")) -> ("error out"=w2469:errorcluster)  [unwired: 2 in]
      }
      event "Sample name": Value Change {
        n703 = event-data() -> ("NewVal"=w2472:string)  [unwired: 1 in]
        n704 = To Variant(anything=w2472) -> (Variant=w2474:variant)
        n705 = call "MAIN_save_parameters_TDMS.vi"("error in"=w2476, "Data"=w2474, "Channel name"="Sample name" ("group name")) -> ("error out"=w2475:errorcluster)  [unwired: 2 in]
      }
      event "N movies", "N frames": Value Change {
        n706 = event-data() -> ()  [unwired: 1 in, 1 out]
        n707 = local read "N frames"() -> (w2478:i32)
        n708 = local read "N movies"() -> (w2480:i32)
        n709 = To Variant(anything=w2480) -> (Variant=w2482:variant)
        n710 = call "MAIN_save_parameters_TDMS.vi"("error in"=w2479, "Data"=w2482, "Channel name"="N movies" ("group name")) -> ("error out"=w2481:errorcluster)  [unwired: 2 in]
        n711 = To Variant(anything=w2478) -> (Variant=w2485:variant)
        n712 = call "MAIN_save_parameters_TDMS.vi"("error in"=w2481, "Data"=w2485, "Channel name"="N frames" ("group name")) -> ("error out"=w2477:errorcluster)  [unwired: 2 in]
      }
      event "FOV size (um)": Value Change {
        n713 = event-data() -> ("NewVal"=w2486:dbl)  [unwired: 1 in]
        n714 = To Variant(anything=w2486) -> (Variant=w2488:variant)
        n715 = call "MAIN_save_parameters_TDMS.vi"("error in"=w2490, "Data"=w2488, "Channel name"="Time lapse FOV" ("group name")) -> ("error out"=w2489:errorcluster)  [unwired: 2 in]
      }
      event "Mosaic size X", "Mosaic size Y": Value Change {
        n716 = event-data() -> ()  [unwired: 1 in, 1 out]
        n717 = local read "Mosaic size X"() -> (w2493:i32)
        n718 = local read "Mosaic size Y"() -> (w2492:i32)
        n719 = Build Array(w2493, w2492) -> (w2491:i32[])
        n720 = To Variant(anything=w2491) -> (Variant=w2495:variant)
        n721 = call "MAIN_save_parameters_TDMS.vi"("error in"=w2497, "Data"=w2495, "Channel name"="Mosaic size" ("group name")) -> ("error out"=w2496:errorcluster)  [unwired: 2 in]
      }
      event "PID gains": Value Change {
        n722 = event-data() -> ("NewVal"=w2498:T2)  [unwired: 1 in]
        n723 = Cluster To Array(cluster=w2498) -> (array=w2499:dbl[])
        n724 = To Variant(anything=w2499) -> (Variant=w2501:variant)
        n725 = call "MAIN_save_parameters_TDMS.vi"("error in"=w2503, "Data"=w2501, "Channel name"="PID gains" ("group name")) -> ("error out"=w2502:errorcluster)  [unwired: 2 in]
      }
      event "Brightfield intensity": Value Change {
        n726 = event-data() -> ("NewVal"=w2504:dbl)  [unwired: 1 in]
        n727 = To Variant(anything=w2504) -> (Variant=w2506:variant)
        n728 = call "MAIN_save_parameters_TDMS.vi"("error in"=w2508, "Data"=w2506, "Channel name"="Brightfield intensity" ("group name")) -> ("error out"=w2507:errorcluster)  [unwired: 2 in]
      }
      event "Define list": Value Change {
        n729 = event-data() -> ()  [unwired: 1 in, 1 out]
        n730 = case shown="True" "Define list" {
          tunnel: w2512 -> [w2513 w2517]
          tunnel: w2511 -> [_ w2516]
          tunnel: [w2513 w2514] -> w2510
          frame False {
          }
          frame True {
            n731 = Enqueue Element At Opposite End(queue=w2516, element=T11 {"variant"=variant, "Instruction"=enum."Main_merFISH_buffer_probe_list"}, error in (no error)=w2517) -> (error out=w2514:errorcluster)  [unwired: 1 in, 2 out]
          }
        }
      }
      event "Save movie": Value Change {
        n732 = event-data() -> ("NewVal"=w2520:bool)  [unwired: 1 in]
        n733 = Unbundle By Name(w2519) -> ("Camera"=w2518:bool)
        n734 = case shown="True" w2518 {
          tunnel: w2523 -> [_ w2529]
          tunnel: w2522 -> [w2525 w2528]
          tunnel: [w2524 w2527] -> w2521
          tunnel: w2520 -> [_ w2526]
          frame False {
            n735 = call "Display Message to User26"("error in (no error)"=w2525) -> ("error out"=w2524:errorcluster)  [unwired: 9 in, 1 out]
          }
          frame True {
            n736 = case shown="True" w2526 {
              tunnel: w2529 -> [_ w2533]
              tunnel: w2528 -> [w2530 w2532]
              tunnel: [w2530 w2531] -> w2527
              frame False {
              }
              frame True {
                n737 = Flush Queue(queue=w2533, error in (no error)=w2532) -> (queue out=w2535:refnum<queue>, error out=w2534:errorcluster)  [unwired: 1 out]
                n738 = Enqueue Element(queue=w2535, element=T11 {"variant"=variant, "Instruction"=enum."Main_save_movie"} ("Q_main_element"), error in (no error)=w2534) -> (error out=w2531:errorcluster)  [unwired: 1 in, 2 out]
              }
            }
          }
        }
      }
      event "Start scan": Value Change {
        n739 = event-data() -> ()  [unwired: 1 in, 1 out]
        n740 = Unbundle By Name(w2542) -> ("Camera"=w2539:bool, "DAQ"=w2541:bool, "PiFoc"=w2540:bool)
        n741 = Build Array(w2539, w2541, w2540) -> (w2538:bool[])
        n742 = And Array Elements(Boolean array=w2538) -> (logical AND=w2537:bool)
        n743 = case shown="True" w2537 {
          tunnel: w2545 -> [w2547 w2551]
          tunnel: w2544 -> [_ w2550]
          tunnel: [w2546 w2549] -> w2543
          frame False {
            n744 = call "Display Message to User22"("error in (no error)"=w2547) -> ("error out"=w2546:errorcluster)  [unwired: 9 in, 1 out]
          }
          frame True {
            n745 = case shown="True" "Start scan" {
              tunnel: w2551 -> [w2552 w2555]
              tunnel: w2550 -> [_ w2554]
              tunnel: [w2552 w2553] -> w2549
              frame False {
              }
              frame True {
                n746 = Flush Queue(queue=w2554, error in (no error)=w2555) -> (queue out=w2557:refnum<queue>, error out=w2556:errorcluster)  [unwired: 1 out]
                n747 = Enqueue Element(queue=w2557, element=T11 {"variant"=variant, "Instruction"=enum."Main_init_single_scan"} ("Q_main_element"), error in (no error)=w2556) -> (error out=w2553:errorcluster)  [unwired: 1 in, 2 out]
              }
            }
          }
        }
      }
      event "merFISH": Value Change {
        n748 = event-data() -> ("NewVal"=w2563:bool)  [unwired: 1 in]
        n749 = Unbundle(w2568) -> ("ASI"=w2567:bool, "DAQ"=w2566:bool, "Camera"=w2565:bool, "Pump"=w2562:bool, "Valve"=w2561:bool, "PiFoc"=w2560:bool, "FPGA"=w2559:bool)
        n750 = Build Array(w2567, w2566, w2565, w2562, w2561, w2560, w2559) -> (w2564:bool[])
        n751 = And Array Elements(Boolean array=w2564) -> (logical AND=w2569:bool)
        n752 = case shown="True" w2569 {
          tunnel: w2572 -> [w2575 w2579]
          tunnel: w2571 -> [_ w2578]
          tunnel: [w2573 w2577] -> w2570
          tunnel: w2563 -> [_ w2576]
          frame False {
            n753 = call "Display Message to User27"("error in (no error)"=w2575) -> ("error out"=w2574:errorcluster)  [unwired: 9 in, 1 out]
            n754 = invoke on="merFISH" class="Bool (strict)" method="Reinit To Default"(error in=w2574) -> (error out=w2573:errorcluster)  [unwired: 2 in, 2 out]
          }
          frame True {
            n755 = case shown="False" w2576 {
              tunnel: w2579 -> [w2580 w2583]
              tunnel: w2578 -> [_ w2582]
              tunnel: [w2580 w2581] -> w2577
              frame False {
              }
              frame True {
                (unwired) T39 {"405"=FALSE, "488"=FALSE, "561"=FALSE, "641"=FALSE, "BF"=FALSE} ("Laser error status")
                n756 = Flush Queue(queue=w2582, error in (no error)=w2583) -> (queue out=w2585:refnum<queue>, error out=w2584:errorcluster)  [unwired: 1 out]
                n757 = Enqueue Element(queue=w2585, element=T11 {"variant"=variant, "Instruction"=enum."Main_merFISH_init"} ("Q_main_element"), error in (no error)=w2584) -> (error out=w2581:errorcluster)  [unwired: 1 in, 2 out]
              }
            }
          }
        }
      }
      event "Abort scan", "Abort merFISH", "Abort movie": Value Change {
        n758 = event-data() -> ("NewVal"=w2588:bool)  [unwired: 1 in]
        n759 = global write "Global_ABORT.vi" "ABORT"(w2588) -> ()
      }
      event "stop": Value Change {
        n760 = event-data() -> ()  [unwired: 1 in, 1 out]
        n761 = case shown="True" "stop" {
          tunnel: w2592 -> [_ w2598]
          tunnel: w2589 -> [w2593 _]
          tunnel: [w2593 w2594] -> w2590
          frame False {
          }
          frame True {
            n762 = Flush Queue(queue=w2598) -> (queue out=w2597:refnum<queue>, error out=w2595:errorcluster)  [unwired: 1 in, 1 out]
            n763 = Enqueue Element(queue=w2597, element=T11 {"variant"=variant, "Instruction"=enum."Main_STOP"} ("Q_main_element"), error in (no error)=w2595) -> (error out=w2594:errorcluster)  [unwired: 1 in, 2 out]
          }
        }
      }
    }
    "MAIN_producer" <- w2007
    n764 = global read "Global_MAIN.vi" "Stop main vi"() -> (w2019:bool)
  }
  n765 = call "DAQ_main.vi"() -> ()  [unwired: 12 in]
  n766 = call "ASI_stage_main.vi"() -> ()  [unwired: 12 in]
  n767 = call "PIEZO_main.vi"() -> ()  [unwired: 12 in]
  n768 = call "VALVE_main.vi"() -> ()  [unwired: 12 in]
  n769 = call "PUMP_main.vi"() -> ()  [unwired: 12 in]
  n770 = call "FPGA_main.vi"() -> ()  [unwired: 12 in]
  n771 = call "sCMOS_main.vi"() -> ()  [unwired: 12 in]
  n772 = Release Queue(queue=w45, error in (no error)=w44) -> ()  [unwired: 1 in, 3 out]
